vi "Lab Panel V3.1.vi"() -> ()   [LabVIEW 2013]
uses:
  <vilib>/Platform/TimedLoop/XDataNode/timing_clust.ctl
  <vilib>/Platform/TimedLoop/XDataNode/nitl_modes.ctl
  <vilib>/Platform/TimedLoop/XDataNode/wakeup.ctl
  Global 1.vi
  <vilib>/platform/TimedLoop/XDataNode/XDataNode.xnode
  <vilib>/Platform/TimedLoop/XDataNode/XDNodeRunTimeDep.lvlib
panel:
  out "TEMP update":bool
  out "AI update":bool
  in  "stop":bool
  in  "Tab Control 2":T1(tab)
  out "LAB05-2 (SIG)":T2 {"PF" format="%.2f"; "AMPS" format="%.1f"}
  out "LAB05-1 (SIG)":T2 {"PF" format="%.2f"; "AMPS" format="%.1f"}
  out "LAB04-2 (SIG)":T2 {"PF" format="%.2f"; "AMPS" format="%.1f"}
  out "LAB04-1 (SIG)":T2 {"PF" format="%.2f"; "AMPS" format="%.1f"}
  out "LAB03-2 (SIG)":T2 {"PF" format="%.2f"; "AMPS" format="%.1f"}
  out "LAB03-1 (SIG)":T2 {"PF" format="%.2f"; "AMPS" format="%.1f"}
  out "LAB02-2 (SIG)":T2 {"PF" format="%.2f"; "AMPS" format="%.1f"}
  in  "LAB01-1RUN":bool
  in  "LAB05-1 (O/I)":bool
  in  "LAB05-2 (O/I)":bool
  in  "LAB04-1 (O/I)":bool
  in  "LAB04-2 (O/I)":bool
  in  "LAB02-1 (O/I)":bool
  in  "LAB02-2 (O/I)":bool
  in  "LAB01-2 (O/I)":bool
  in  "LAB01-1 (O/I)":bool
  in  "LAB03-1 (O/I)":bool
  in  "LAB05-2 RUN":bool
  in  "LAB05-1 RUN":bool
  in  "LAB04-2 RUN":bool
  in  "LAB04-1 RUN":bool
  in  "LAB03-2 RUN":bool
  in  "LAB03-1 RUN":bool
  in  "LAB02-2 RUN":bool
  in  "LAB02-1 RUN":bool
  in  "LAB01-2 RUN":bool
  in  "LAB05-2 SELECT":T3(radio)
  in  "LAB05-1 SELECT":T3(radio)
  in  "LAB04-2 SELECT":T3(radio)
  in  "LAB04-1 SELECT":T3(radio)
  in  "LAB03-2 SELECT":T3(radio)
  in  "LAB03-1 SELECT":T3(radio)
  in  "LAB02-2 SELECT":T3(radio)
  in  "LAB02-1 SELECT":T3(radio)
  in  "LAB01-2 SELECT":T3(radio)
  in  "LAB01-1 SELECT":T3(radio)
  in  "LAB03-2 (O/I)":bool
  out "LAB01-1 (SIG)":T2 {"PF" format="%.2f"; "AMPS" format="%.1f"}
  out "LAB01-2 (SIG)":T2 {"PF" format="%.2f"; "AMPS" format="%.1f"}
  out "LAB02-1 (SIG)":T2 {"PF" format="%.2f"; "AMPS" format="%.1f"}
  out "LAB05-2 (DISP)":T4 {"MINS" format="%.2g"}
  out "LAB05-1 (DISP)":T4 {"MINS" format="%.2g"}
  out "LAB04-2 (DISP)":T4 {"MINS" format="%.2g"}
  out "LAB04-1 (DISP)":T4 {"MINS" format="%.2g"}
  out "LAB03-2 (DISP)":T4 {"MINS" format="%.2g"}
  out "LAB03-1 (DISP)":T4 {"MINS" format="%.2g"}
  in  "LAB05-2 (SET)":T5
  in  "LAB05-1 (SET)":T5
  in  "LAB04-2 (SET)":T5
  in  "LAB04-1 (SET)":T5
  in  "LAB03-2 (SET)":T5
  in  "LAB03-1 (SET)":T5
  out "LAB02-2 (DISP)":T4 {"MINS" format="%.2g"}
  out "LAB02-1 (DISP)":T4 {"MINS" format="%.2g"}
  in  "LAB02-2 (SET)":T5
  in  "LAB02-1 (SET)":T5
  out "LAB05-2 (RESULT)":bool
  out "LAB05-1 (RESULT)":bool
  out "LAB04-2 (RESULT)":bool
  out "LAB04-1 (RESULT)":bool
  out "LAB03-2 (RESULT)":bool
  out "LAB03-1 (RESULT)":bool
  out "LAB02-2 (RESULT)":bool
  out "LAB02-1 (RESULT)":bool
  out "LAB01-2 (RESULT)":bool
  out "LAB01-1 (RESULT)":bool
  in  "LAB01-1 (SET)":T5
  in  "LAB01-2 (SET)":T5
  out "LAB01-1 (DISP)":T4 {"MINS" format="%.2g"}
  out "LAB01-2 (DISP)":T4 {"MINS" format="%.2f"}
  in  "Network Directory":path
  in  "JIG OFF TIME (S)":dbl=2.0 min=2.0 max=10.0 step=0.5 format="%.1g"
  in  "JIG ON TIME (S)":dbl=1.0 min=1.0 max=10.0 step=0.5 format="%.1g"
  out "LAB05-2 (FAIL)":cluster{"LO":dbl, "HI":dbl}
  out "LAB05-1 (FAIL)":cluster{"LO":dbl, "HI":dbl}
  out "LAB04-2 (FAIL)":cluster{"LO":dbl, "HI":dbl}
  out "LAB04-1 (FAIL)":cluster{"LO":dbl, "HI":dbl}
  out "LAB03-2 (FAIL)":cluster{"LO":dbl, "HI":dbl}
  out "LAB03-1 (FAIL)":cluster{"LO":dbl, "HI":dbl}
  out "LAB02-2 (FAIL)":cluster{"LO":dbl, "HI":dbl}
  out "LAB02-1 (FAIL)":cluster{"LO":dbl, "HI":dbl}
  out "LAB01-2 (FAIL)":cluster{"LO":dbl, "HI":dbl}
  out "LAB01-1 (FAIL)":cluster{"LO":dbl, "HI":dbl}
  out "LAB05-2 (TEMP START)":cluster{"TL":dbl, "TN":dbl}
  out "LAB04-2 (TEMP START)":cluster{"TL":dbl, "TN":dbl}
  out "LAB03-2 (TEMP START)":cluster{"TL":dbl, "TN":dbl}
  out "LAB02-2 (TEMP START)":cluster{"TL":dbl, "TN":dbl}
  out "LAB01-2 (TEMP START)":cluster{"TL":dbl, "TN":dbl}
  out "LAB05-1 (TEMP START)":cluster{"TL":dbl, "TN":dbl}
  out "LAB04-1 (TEMP START)":cluster{"TL":dbl, "TN":dbl}
  out "LAB03-1 (TEMP START)":cluster{"TL":dbl, "TN":dbl}
  out "LAB02-1 (TEMP START)":cluster{"TL":dbl, "TN":dbl}
  out "LAB01-1 (TEMP START)":cluster{"TL":dbl, "TN":dbl}
  out "LAB01-1 (JIG)":bool
  out "LAB01-2 (JIG)":bool
  out "LAB02-1 (JIG)":bool
  out "LAB02-2 (JIG)":bool
  out "LAB03-1 (JIG)":bool
  out "LAB03-2 (JIG)":bool
  out "LAB04-1 (JIG)":bool
  out "LAB04-2 (JIG)":bool
  out "LAB05-1 (JIG)":bool
  out "LAB05-2 (JIG)":bool
  out "LAB01 (CAL)":T6 {"2 (TN) cal" min=0.0 step=0.01 format="%.2f"; "2 (TL) cal" min=0.0 step=0.01 format="%.2f"; "2 (PF) cal" min=0.0 step=0.01 format="%.2f"; "2 (V) cal" min=0.0 step=0.01 format="%.2f"; "2 (A) cal" min=0.0 step=0.01 format="%.2f"; "1 (TN) cal" min=0.0 step=0.01 format="%.2f"; "1 (TL) cal" min=0.0 step=0.01 format="%.2f"; "1 (PF) cal" min=0.0 step=0.01 format="%.2f"; "1 (V) cal" min=0.0 step=0.01 format="%.2f"; "1  (A) cal" min=0.0 step=0.01 format="%.2f"}
  out "LAB03 (CAL)":T6 {"2 (TN) cal" min=0.0 step=0.01 format="%.2f"; "2 (TL) cal" min=0.0 step=0.01 format="%.2f"; "2 (PF) cal" min=0.0 step=0.01 format="%.2f"; "2 (V) cal" min=0.0 step=0.01 format="%.2f"; "2 (A) cal" min=0.0 step=0.01 format="%.2f"; "1 (TN) cal" min=0.0 step=0.01 format="%.2f"; "1 (TL) cal" min=0.0 step=0.01 format="%.2f"; "1 (PF) cal" min=0.0 step=0.01 format="%.2f"; "1 (V) cal" min=0.0 step=0.01 format="%.2f"; "1  (A) cal" min=0.0 step=0.01 format="%.2f"}
  out "LAB02 (CAL)":T7 {"2 (TN) cal" min=0.0 step=0.01 format="%.2f"; "2 (TL) cal" min=0.0 step=0.01 format="%.2f"; "2 (PF) cal" min=0.0 step=0.01 format="%.2f"; "2 (V) cal" min=0.0 step=0.01 format="%.2f"; "2 (A) cal" min=0.0 step=0.01 format="%.2f"; "1 (TN) cal" min=0.0 step=0.01 format="%.2f"; "1 (TL) cal" min=0.0 step=0.01 format="%.2f"; "1 (PF) cal" min=0.0 step=0.01 format="%.2f"; "1 (V) cal" min=0.0 step=0.01 format="%.2f"; "1 (A) cal" min=0.0 step=0.01 format="%.2f"}
  out "LAB05 (CAL)":T6 {"2 (TN) cal" min=0.0 step=0.01 format="%.2f"; "2 (TL) cal" min=0.0 step=0.01 format="%.2f"; "2 (PF) cal" min=0.0 step=0.01 format="%.2f"; "2 (V) cal" min=0.0 step=0.01 format="%.2f"; "2 (A) cal" min=0.0 step=0.01 format="%.2f"; "1 (TN) cal" min=0.0 step=0.01 format="%.2f"; "1 (TL) cal" min=0.0 step=0.01 format="%.2f"; "1 (PF) cal" min=0.0 step=0.01 format="%.2f"; "1 (V) cal" min=0.0 step=0.01 format="%.2f"; "1  (A) cal" min=0.0 step=0.01 format="%.2f"}
  out "LAB04 (CAL)":T6 {"2 (TN) cal" min=0.0 step=0.01 format="%.2f"; "2 (TL) cal" min=0.0 step=0.01 format="%.2f"; "2 (PF) cal" min=0.0 step=0.01 format="%.2f"; "2 (V) cal" min=0.0 step=0.01 format="%.2f"; "2 (A) cal" min=0.0 step=0.01 format="%.2f"; "1 (TN) cal" min=0.0 step=0.01 format="%.2f"; "1 (TL) cal" min=0.0 step=0.01 format="%.2f"; "1 (PF) cal" min=0.0 step=0.01 format="%.2f"; "1 (V) cal" min=0.0 step=0.01 format="%.2f"; "1  (A) cal" min=0.0 step=0.01 format="%.2f"}
  out "calibration file error out":errorcluster
  in  "CALIBRATE":bool
  in  "Tab Control":T8(tab)
  out "LAB01-2 (GRAPH)":dynamicdata(graph)
  out "LAB01-1 (GRAPH)":dynamicdata(graph)
  out "LAB02-2 (GRAPH)":dynamicdata(graph)
  out "LAB02-1 (GRAPH)":dynamicdata(graph)
  out "LAB03-2 (GRAPH)":dynamicdata(graph)
  out "LAB03-1 (GRAPH)":dynamicdata(graph)
  out "LAB04-2 (GRAPH)":dynamicdata(graph)
  out "LAB04-1 (GRAPH)":dynamicdata(graph)
  out "LAB05-2 (GRAPH)":dynamicdata(graph)
  out "LAB05-1 (GRAPH)":dynamicdata(graph)
  out "LAB05 TEMP":T9
  out "LAB04 TEMP":T9
  out "LAB02 TEMP":T9
  out "LAB01 TEMP":T9
  out "LAB03 TEMP":T9
  out "Analog Error Array":errorcluster[](array[cluster])
  out "AI loop time":dbl format="%.6g"
  out "loops":dbl
  in  "loop  delay(mS)":dbl
  out "on loops":dbl
  out "off loops":dbl
  out "jig cycle":dbl
  out "LAB01-1 (TDMS)":refnum<k34>
  out "data file error":errorcluster
  out "LAB02-1 (TDMS)":refnum<k34>
  out "LAB01-2 (TDMS)":refnum<k34>
  out "LAB02-2 (TDMS)":refnum<k34>
  out "LAB03-1 (TDMS)":refnum<k34>
  out "LAB03-2 (TDMS)":refnum<k34>
  out "LAB04-1 (TDMS)":refnum<k34>
  out "LAB04-2 (TDMS)":refnum<k34>
  out "LAB05-1 (TDMS)":refnum<k34>
  out "LAB05-2 (TDMS)":refnum<k34>
  # "LAB01"
  # "LAB02"
  # "LAB05"
  # "LAB03"
  # "LAB04"
  # "LAB01"
  # "LAB02"
  # "LAB03"
  # "LAB04"
  # "LAB05"
  # "JIG SET"
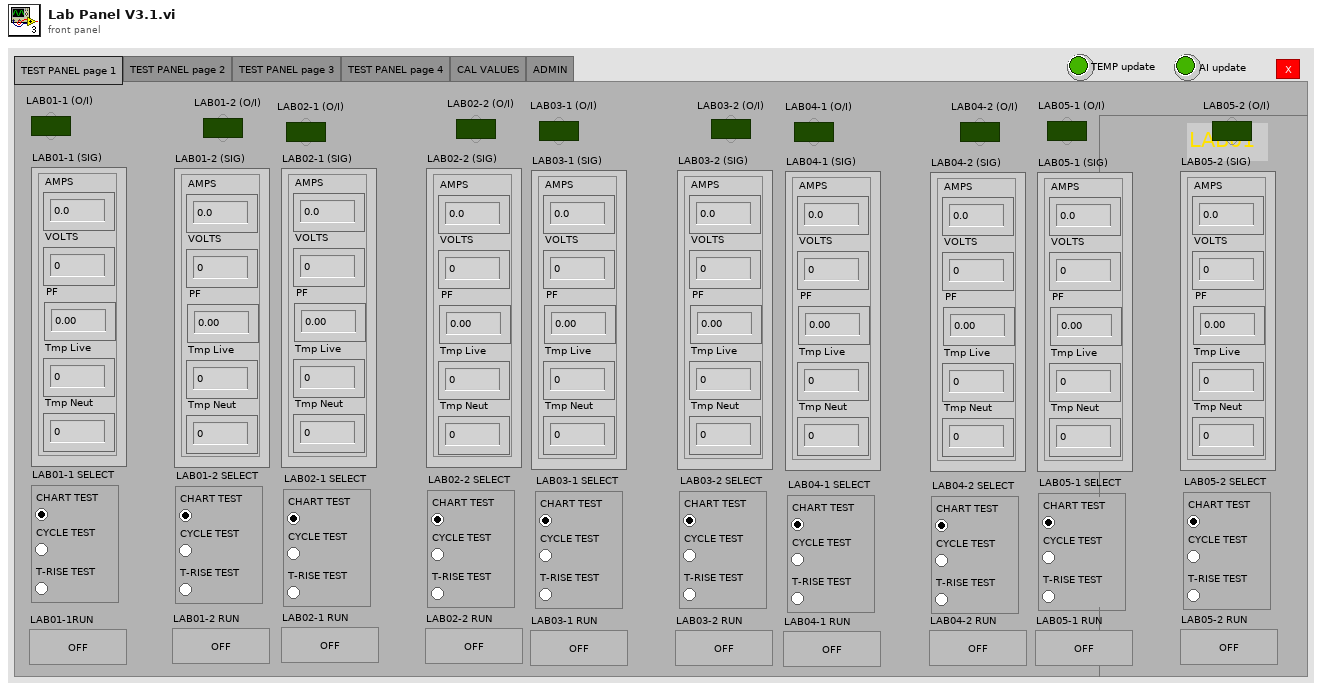
[diagram p1: front panel]
types:
  T1 = enum32{"TEST PANEL page 1", "TEST PANEL page 2", "TEST PANEL page 3", "TEST PANEL page 4", "CAL VALUES", "ADMIN"}
  T2 = cluster{"AMPS":dbl, "VOLTS":dbl, "PF":dbl, "Tmp Live":dbl, "Tmp Neut":dbl}
  T3 = enum32{"CHART TEST", "CYCLE TEST", "T-RISE TEST"}
  T4 = cluster{"CYCLE":dbl, "MINS":dbl, "STATUS":string}
  T5 = cluster{"NAME":string, "DESCRIPTION":string, "CYCLES":dbl, "T-RISE mins":dbl, "T-RISE deg C":dbl}
  T6 = cluster{"1  (A) cal":dbl, "1 (V) cal":dbl, "1 (PF) cal":dbl, "1 (TL) cal":dbl, "1 (TN) cal":dbl, "2 (A) cal":dbl, "2 (V) cal":dbl, "2 (PF) cal":dbl, "2 (TL) cal":dbl, "2 (TN) cal":dbl}
  T7 = cluster{"1 (A) cal":dbl, "1 (V) cal":dbl, "1 (PF) cal":dbl, "1 (TL) cal":dbl, "1 (TN) cal":dbl, "2 (A) cal":dbl, "2 (V) cal":dbl, "2 (PF) cal":dbl, "2 (TL) cal":dbl, "2 (TN) cal":dbl}
  T8 = enum32{"LAB01", "LAB02", "LAB03", "LAB04", "LAB05", "TEMPERATURE", "ERROR"}
  T9 = cluster{"T1 Live":dbl, "T1 Neut":dbl, "T2 Live":dbl, "T2 Neut":dbl, "ID":dbl, "ER":dbl}
  T10 = enum8{"Enabled", "Disabled", "Disabled and Grayed Out"}
  T11 = typedef "XDNodeRunTimeDep.lvlib/timing_clust.ctl" = cluster{"Expected End [f-1]":u64, "Actual End [f-1]":u64, "Finished Late? [f-1]":bool, "Expected End [i-1]":u64, "Actual End [i-1]":u64, "Finished Late? [i-1]":bool, "Expected Start [i]":u64, "Actual Start [i]":u64, "Expected Start [f]":u64, "Actual Start [f]":u64, "Source Name":string, "Structure Name":string, "Period":i64, "Deadline":i64, "Offset":i64, "Start":i64, "Priority":i32, "Timeout":i32, "Mode":T12, "Wakeup Reason":T13, "Error":errorcluster, "Source Type":string, "Secondary Source Type":string, "Global End Time":u64, "Global Start Time":u64, "Frame Duration":u64, "Iteration Duration":u64, "Assigned CPU":i32, "I/O Scan Engine Mode":u32}
  T12 = typedef "XDNodeRunTimeDep.lvlib/nitl_modes.ctl" = enum32{"No Change", "Process missed periods, maintain original phase", "Discard missed periods, maintain original phase", "Process missed periods, ignore original phase", "Discard missed periods, ignore original phase"}
  T13 = typedef "XDNodeRunTimeDep.lvlib/wakeup.ctl" = enum32{"Normal", "Aborted", "Asynchronous wakeup", "Timing source error", "Timed loop error", "Timeout"}
  T14 = enum16{"open", "open or create", "create or replace", "create", "open (read-only)"}
  T15 = enum16{"open", "replace", "create", "open or create", "replace or create", "replace or create with confirmation"}
  T16 = cluster{"LAB01-1 (SET)":cluster{"NAME":string, "DESCRIPTION":string, "CYCLES":dbl, "T-RISE mins":dbl, "T-RISE deg C":dbl}, "LAB01-2 (SET)":cluster{"NAME":string, "DESCRIPTION":string, "CYCLES":dbl, "T-RISE mins":dbl, "T-RISE deg C":dbl}, "LAB02-1 (SET)":cluster{"NAME":string, "DESCRIPTION":string, "CYCLES":dbl, "T-RISE mins":dbl, "T-RISE deg C":dbl}, "LAB02-2 (SET)":cluster{"NAME":string, "DESCRIPTION":string, "CYCLES":dbl, "T-RISE mins":dbl, "T-RISE deg C":dbl}, "LAB03-1 (SET)":cluster{"NAME":string, "DESCRIPTION":string, "CYCLES":dbl, "T-RISE mins":dbl, "T-RISE deg C":dbl}, "LAB03-2 (SET)":cluster{"NAME":string, "DESCRIPTION":string, "CYCLES":dbl, "T-RISE mins":dbl, "T-RISE deg C":dbl}, "LAB04-1 (SET)":cluster{"NAME":string, "DESCRIPTION":string, "CYCLES":dbl, "T-RISE mins":dbl, "T-RISE deg C":dbl}, "LAB04-2 (SET)":cluster{"NAME":string, "DESCRIPTION":string, "CYCLES":dbl, "T-RISE mins":dbl, "T-RISE deg C":dbl}, "LAB05-1 (SET)":cluster{"NAME":string, "DESCRIPTION":string, "CYCLES":dbl, "T-RISE mins":dbl, "T-RISE deg C":dbl}, "LAB05-2 (SET)":cluster{"NAME":string, "DESCRIPTION":string, "CYCLES":dbl, "T-RISE mins":dbl, "T-RISE deg C":dbl}, "Network Directory":path}
  T17 = cluster{"T1":dbl, "T2":dbl, "T3":dbl, "T4":dbl, "ID":dbl, "ER":dbl}
  T18 = cluster{"LAB01-1 (A)":dbl, "LAB01-1 (V)":dbl, "LAB01-1 (PF)":dbl, "LAB01-2 (A)":dbl, "LAB01-2 (V)":dbl, "LAB01-2 (PF)":dbl}
  T19 = cluster{"LAB02-1 (A)":dbl, "LAB02-1 (V)":dbl, "LAB02-1 (PF)":dbl, "LAB02-2 (A)":dbl, "LAB02-2 (V)":dbl, "LAB02-2 (PF)":dbl}
  T20 = cluster{"LAB03-1 (A)":dbl, "LAB03-1 (V)":dbl, "LAB03-1 (PF)":dbl, "LAB03-2 (A)":dbl, "LAB03-2 (V)":dbl, "LAB03-2 (PF)":dbl}
  T21 = cluster{"LAB04-1 (A)":dbl, "LAB04-1 (V)":dbl, "LAB04-1 (PF)":dbl, "LAB04-2 (A)":dbl, "LAB04-2 (V)":dbl, "LAB04-2 (PF)":dbl}
  T22 = cluster{"LAB05-1 (A)":dbl, "LAB05-1 (V)":dbl, "LAB05-1 (PF)":dbl, "LAB05-2 (A)":dbl, "LAB05-2 (V)":dbl, "LAB05-2 (PF)":dbl}
  T23 = cluster{"LAB01-1 (FAIL)":cluster{"LO":dbl, "HI":dbl}, "LAB01-1 (SIG)":cluster{"AMPS":dbl, "VOLTS":dbl, "PF":dbl, "Tmp Live":dbl, "Tmp Neut":dbl}, "LAB01-1 (TEMP START)":cluster{"TL":dbl, "TN":dbl}, "LAB01-1 (DISP)":cluster{"CYCLE":dbl, "MINS":dbl, "STATUS":string}, "LAB01-1 (SET)":cluster{"NAME":string, "DESCRIPTION":string, "CYCLES":dbl, "T-RISE mins":dbl, "T-RISE deg C":dbl}, "LAB01-1 (TDMS)":refnum<k34>}
  T24 = cluster{"LAB01-2 (FAIL)":cluster{"LO":dbl, "HI":dbl}, "LAB01-2 (SIG)":cluster{"AMPS":dbl, "VOLTS":dbl, "PF":dbl, "Tmp Live":dbl, "Tmp Neut":dbl}, "LAB01-2 (TEMP START)":cluster{"TL":dbl, "TN":dbl}, "LAB01-2 (DISP)":cluster{"CYCLE":dbl, "MINS":dbl, "STATUS":string}, "LAB01-2 (SET)":cluster{"NAME":string, "DESCRIPTION":string, "CYCLES":dbl, "T-RISE mins":dbl, "T-RISE deg C":dbl}, "LAB01-2 (TDMS)":refnum<k34>}
  T25 = cluster{"LAB02-1 (FAIL)":cluster{"LO":dbl, "HI":dbl}, "LAB02-1 (SIG)":cluster{"AMPS":dbl, "VOLTS":dbl, "PF":dbl, "Tmp Live":dbl, "Tmp Neut":dbl}, "LAB02-1 (TEMP START)":cluster{"TL":dbl, "TN":dbl}, "LAB02-1 (DISP)":cluster{"CYCLE":dbl, "MINS":dbl, "STATUS":string}, "LAB02-1 (SET)":cluster{"NAME":string, "DESCRIPTION":string, "CYCLES":dbl, "T-RISE mins":dbl, "T-RISE deg C":dbl}, "LAB02-1 (TDMS)":refnum<k34>}
  T26 = cluster{"LAB02-2 (FAIL)":cluster{"LO":dbl, "HI":dbl}, "LAB02-2 (SIG)":cluster{"AMPS":dbl, "VOLTS":dbl, "PF":dbl, "Tmp Live":dbl, "Tmp Neut":dbl}, "LAB02-2 (TEMP START)":cluster{"TL":dbl, "TN":dbl}, "LAB02-2 (DISP)":cluster{"CYCLE":dbl, "MINS":dbl, "STATUS":string}, "LAB02-2 (SET)":cluster{"NAME":string, "DESCRIPTION":string, "CYCLES":dbl, "T-RISE mins":dbl, "T-RISE deg C":dbl}, "LAB02-2 (TDMS)":refnum<k34>}
  T27 = cluster{"LAB03-1 (FAIL)":cluster{"LO":dbl, "HI":dbl}, "LAB03-1 (SIG)":cluster{"AMPS":dbl, "VOLTS":dbl, "PF":dbl, "Tmp Live":dbl, "Tmp Neut":dbl}, "LAB03-1 (TEMP START)":cluster{"TL":dbl, "TN":dbl}, "LAB03-1 (DISP)":cluster{"CYCLE":dbl, "MINS":dbl, "STATUS":string}, "LAB03-1 (SET)":cluster{"NAME":string, "DESCRIPTION":string, "CYCLES":dbl, "T-RISE mins":dbl, "T-RISE deg C":dbl}, "LAB03-1 (TDMS)":refnum<k34>}
  T28 = cluster{"LAB03-2 (FAIL)":cluster{"LO":dbl, "HI":dbl}, "LAB03-2 (SIG)":cluster{"AMPS":dbl, "VOLTS":dbl, "PF":dbl, "Tmp Live":dbl, "Tmp Neut":dbl}, "LAB03-2 (TEMP START)":cluster{"TL":dbl, "TN":dbl}, "LAB03-2 (DISP)":cluster{"CYCLE":dbl, "MINS":dbl, "STATUS":string}, "LAB03-2 (SET)":cluster{"NAME":string, "DESCRIPTION":string, "CYCLES":dbl, "T-RISE mins":dbl, "T-RISE deg C":dbl}, "LAB03-2 (TDMS)":refnum<k34>}
  T29 = cluster{"LAB04-1 (FAIL)":cluster{"LO":dbl, "HI":dbl}, "LAB04-1 (SIG)":cluster{"AMPS":dbl, "VOLTS":dbl, "PF":dbl, "Tmp Live":dbl, "Tmp Neut":dbl}, "LAB04-1 (TEMP START)":cluster{"TL":dbl, "TN":dbl}, "LAB04-1 (DISP)":cluster{"CYCLE":dbl, "MINS":dbl, "STATUS":string}, "LAB04-1 (SET)":cluster{"NAME":string, "DESCRIPTION":string, "CYCLES":dbl, "T-RISE mins":dbl, "T-RISE deg C":dbl}, "LAB04-1 (TDMS)":refnum<k34>}
  T30 = cluster{"LAB04-2 (FAIL)":cluster{"LO":dbl, "HI":dbl}, "LAB04-2 (SIG)":cluster{"AMPS":dbl, "VOLTS":dbl, "PF":dbl, "Tmp Live":dbl, "Tmp Neut":dbl}, "LAB04-2 (TEMP START)":cluster{"TL":dbl, "TN":dbl}, "LAB04-2 (DISP)":cluster{"CYCLE":dbl, "MINS":dbl, "STATUS":string}, "LAB04-2 (SET)":cluster{"NAME":string, "DESCRIPTION":string, "CYCLES":dbl, "T-RISE mins":dbl, "T-RISE deg C":dbl}, "LAB04-2 (TDMS)":refnum<k34>}
  T31 = cluster{"LAB05-1 (FAIL)":cluster{"LO":dbl, "HI":dbl}, "LAB05-1 (SIG)":cluster{"AMPS":dbl, "VOLTS":dbl, "PF":dbl, "Tmp Live":dbl, "Tmp Neut":dbl}, "LAB05-1 (TEMP START)":cluster{"TL":dbl, "TN":dbl}, "LAB05-1 (DISP)":cluster{"CYCLE":dbl, "MINS":dbl, "STATUS":string}, "LAB05-1 (SET)":cluster{"NAME":string, "DESCRIPTION":string, "CYCLES":dbl, "T-RISE mins":dbl, "T-RISE deg C":dbl}, "LAB05-1 (TDMS)":refnum<k34>}
  T32 = cluster{"LAB05-2 (FAIL)":cluster{"LO":dbl, "HI":dbl}, "LAB05-2 (SIG)":cluster{"AMPS":dbl, "VOLTS":dbl, "PF":dbl, "Tmp Live":dbl, "Tmp Neut":dbl}, "LAB05-2 (TEMP START)":cluster{"TL":dbl, "TN":dbl}, "LAB05-2 (DISP)":cluster{"CYCLE":dbl, "MINS":dbl, "STATUS":string}, "LAB05-2 (SET)":cluster{"NAME":string, "DESCRIPTION":string, "CYCLES":dbl, "T-RISE mins":dbl, "T-RISE deg C":dbl}, "LAB05-2 (TDMS)":refnum<k34>}
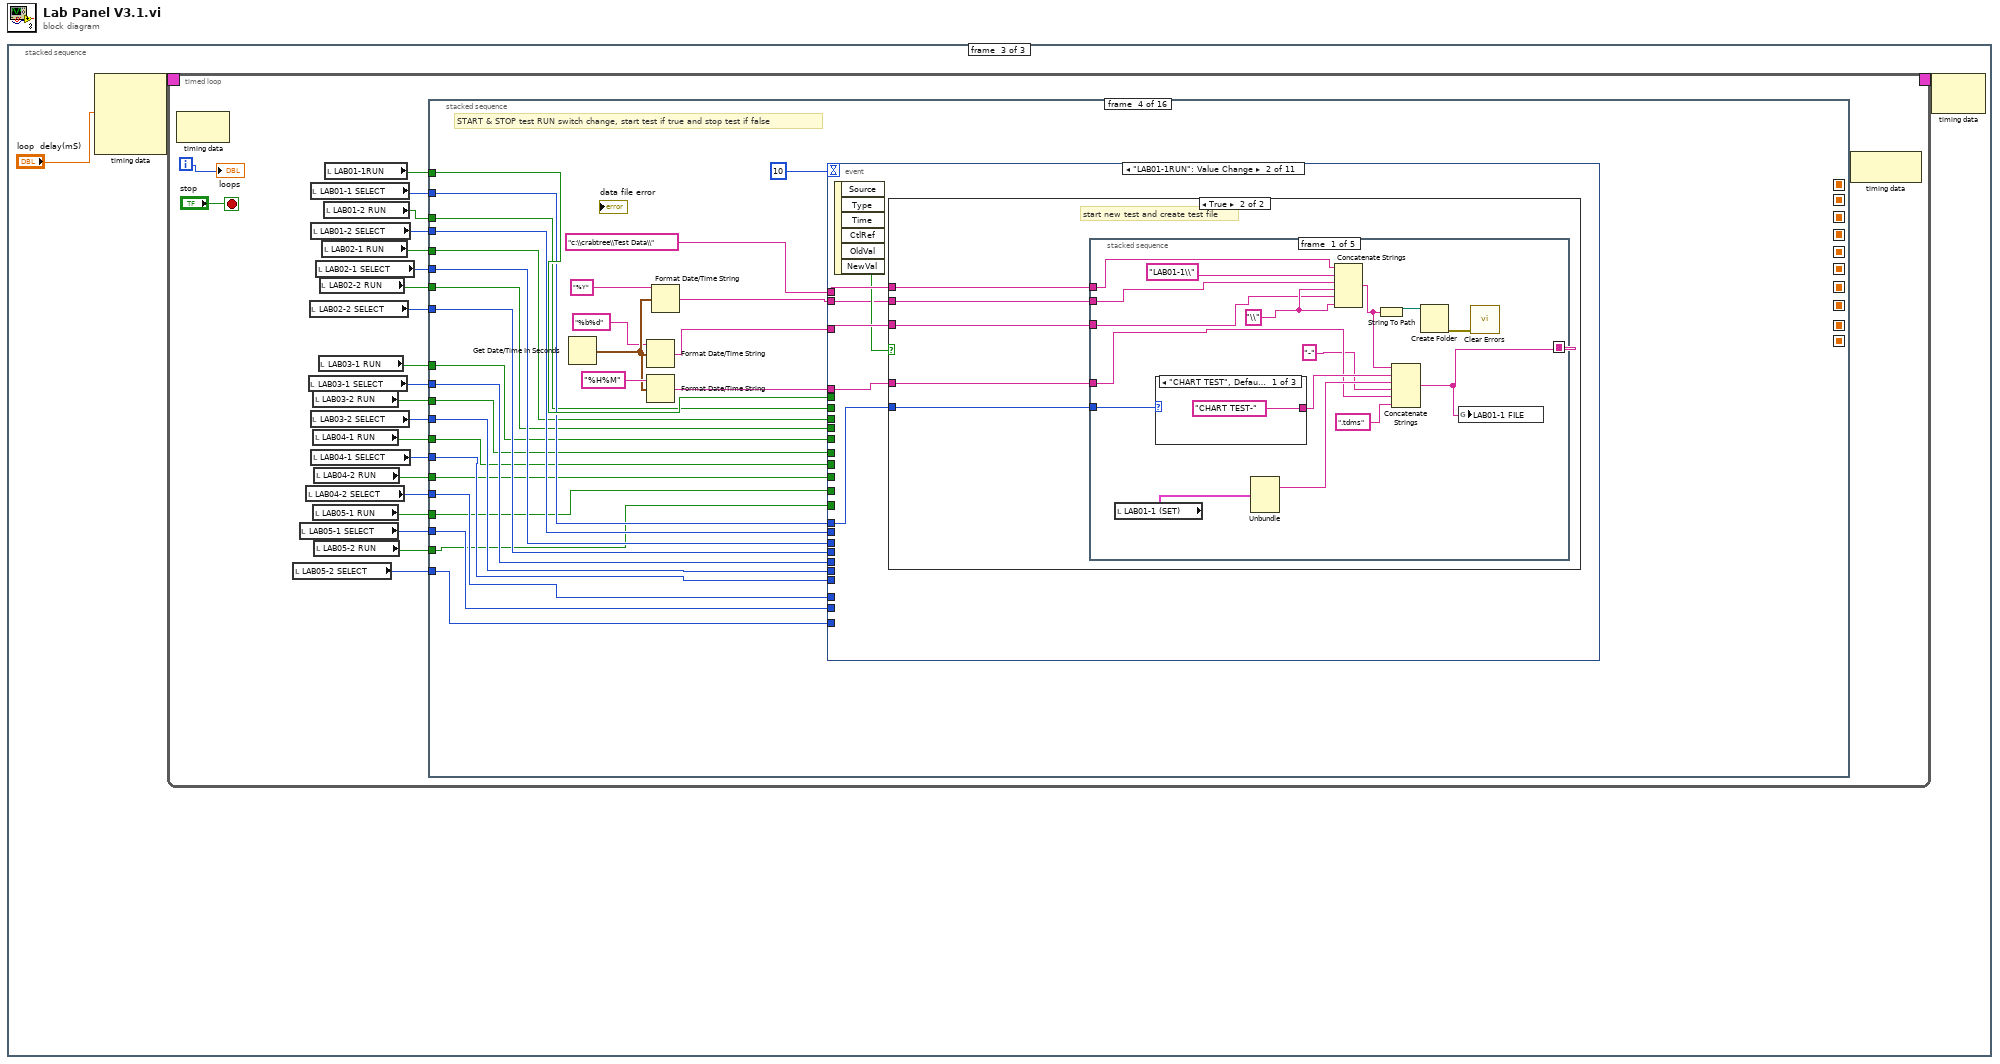
[diagram p0: block diagram]
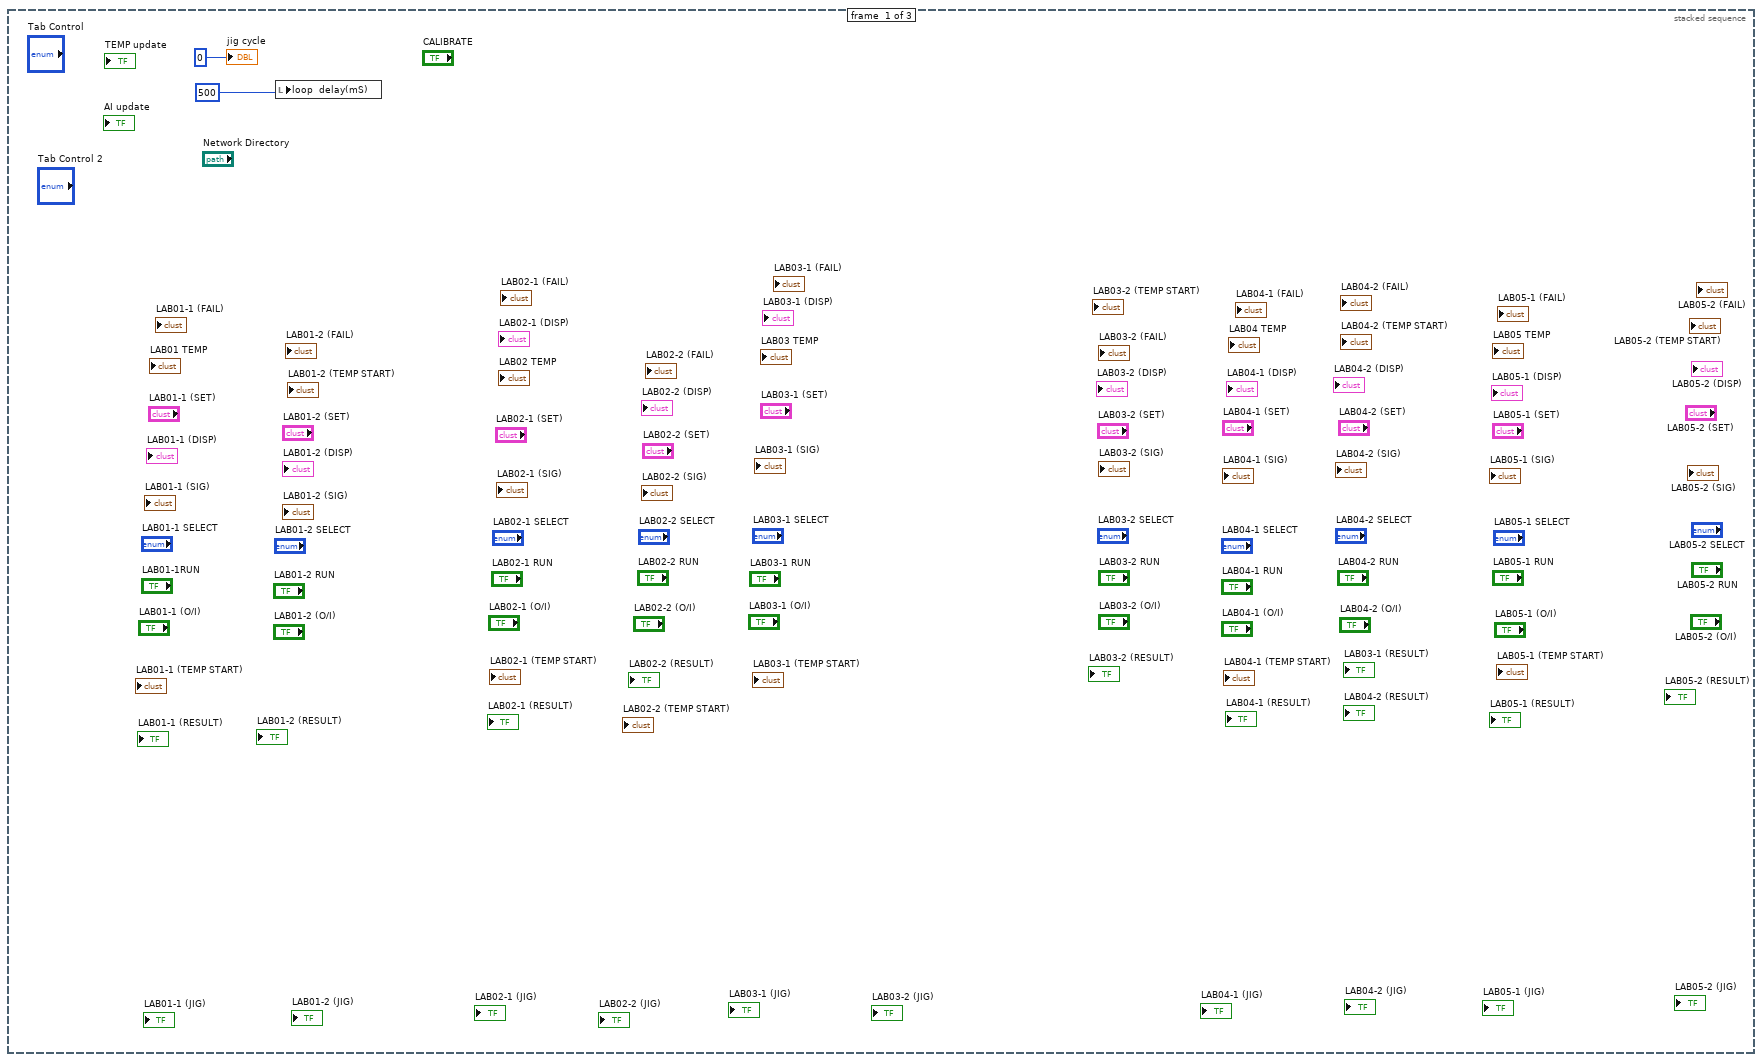
[diagram p2: hidden frame]
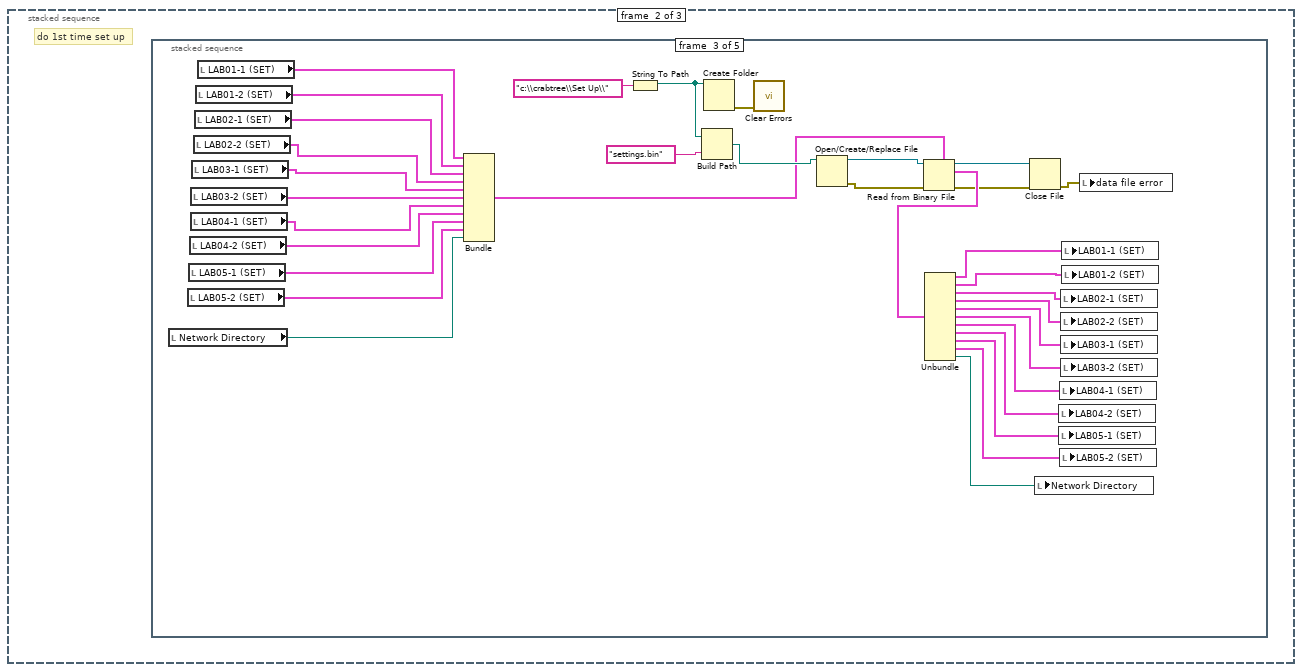
[diagram p3: hidden frame]
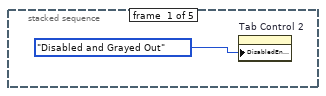
[diagram p4: hidden frame]
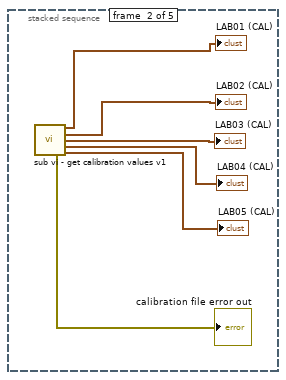
[diagram p5: hidden frame]
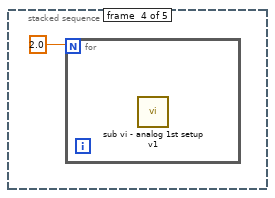
[diagram p6: hidden frame]
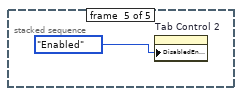
[diagram p7: hidden frame]
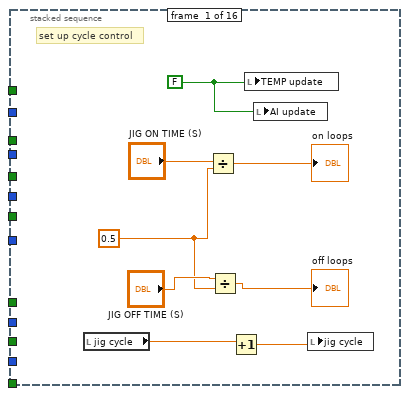
[diagram p8: hidden frame]
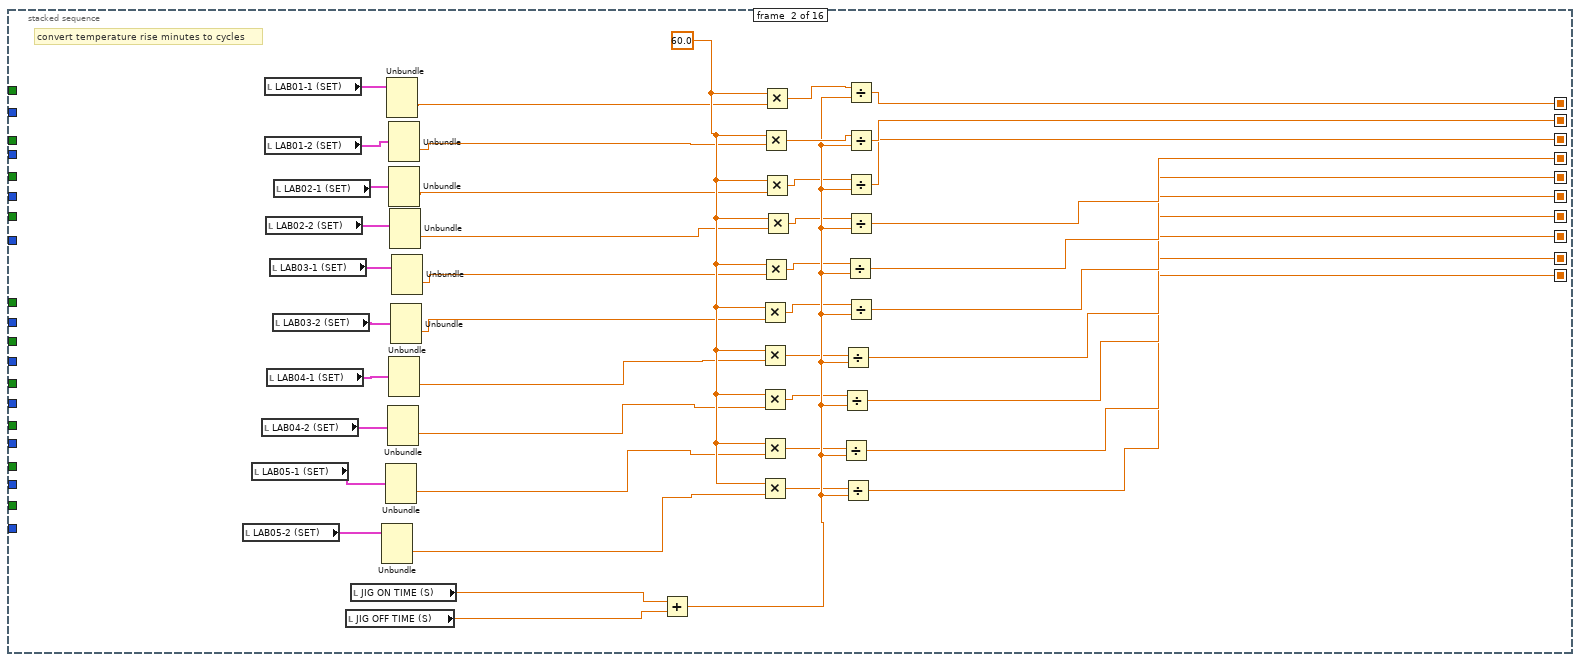
[diagram p9: hidden frame]
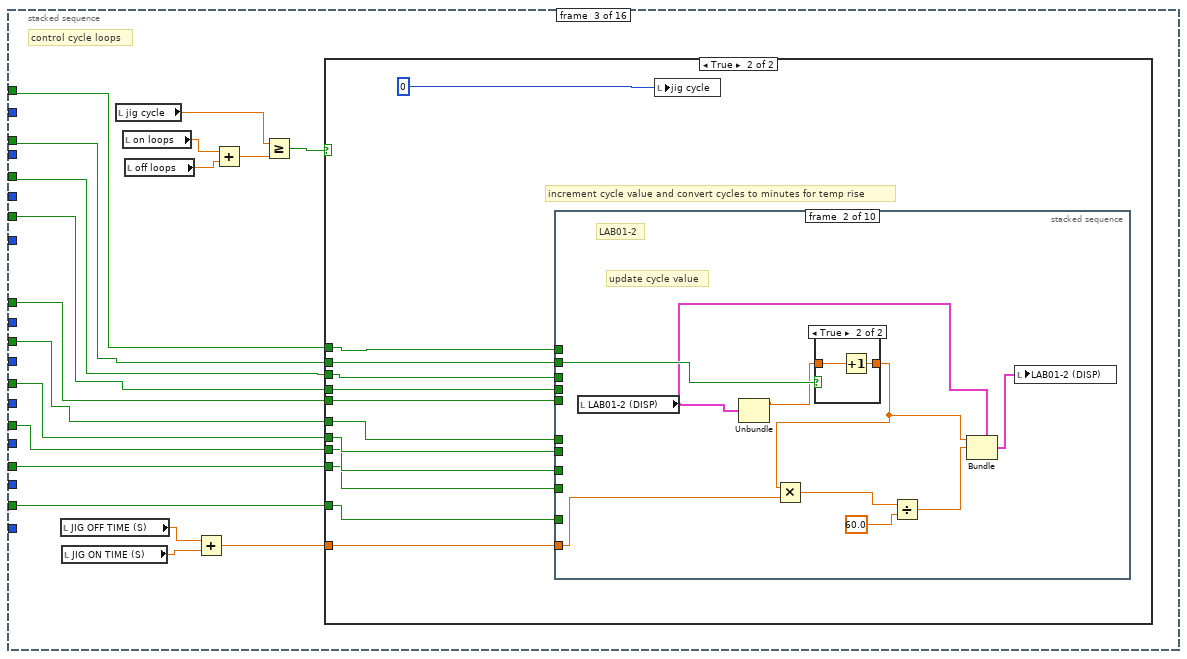
[diagram p10: hidden frame]
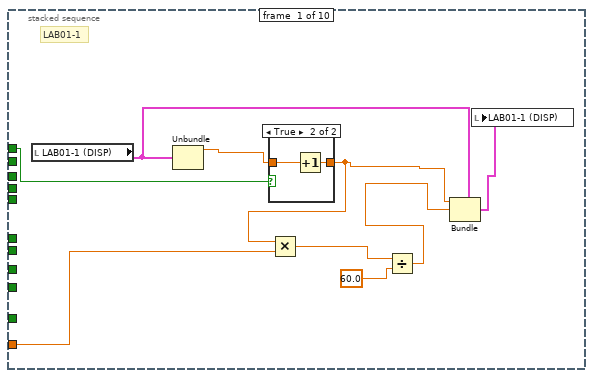
[diagram p12: hidden frame]
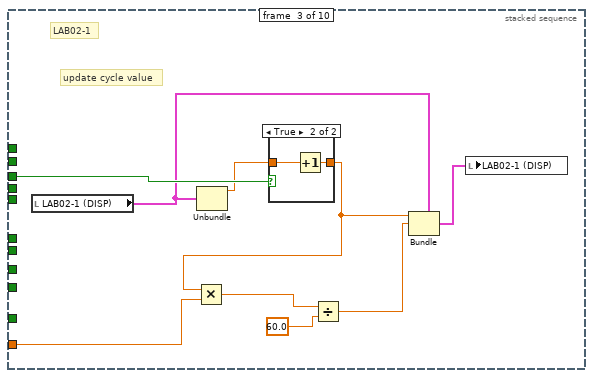
[diagram p15: hidden frame]
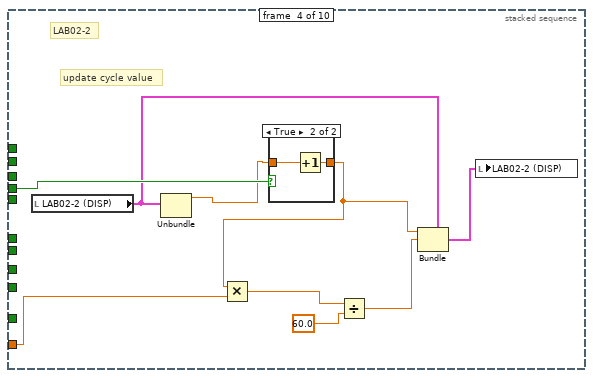
[diagram p17: hidden frame]
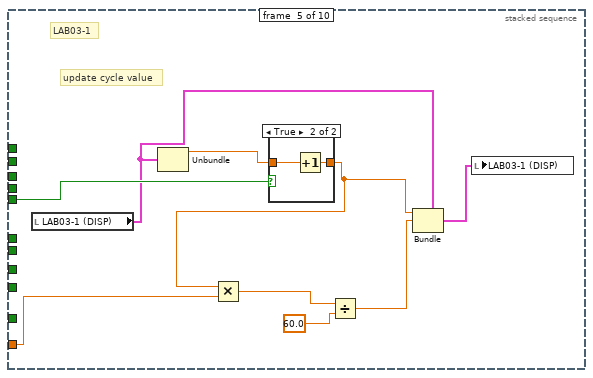
[diagram p19: hidden frame]
diagram:
  n1 = stacked-sequence {
    frame #0 {
      n2 = local write "loop  delay(mS)"(500) -> ()
      "jig cycle" <- 0
    }
    frame #1 {
      # "do 1st time set up"
      n3 = stacked-sequence {
        frame #0 {
          n4 = property on="Tab Control 2" class="TabCtl (strict)"("DisabledEnum"=T10."Disabled and Grayed Out" ("Disabled")) -> ()  [unwired: 2 in, 2 out]
        }
        frame #1 {
          n5 = call "sub vi - get calibration values v1.vi"() -> ("LAB01 (CAL)"=→"LAB01 (CAL)":T6, "LAB02 (CAL)"=→"LAB02 (CAL)":T7, "LAB03 (CAL)"=→"LAB03 (CAL)":T6, "LAB04 (CAL)"=→"LAB04 (CAL)":T6, "calibration file error out"=→"calibration file error out":errorcluster, "LAB05 (CAL)"=→"LAB05 (CAL)":T6)  [unwired: 10 in]
        }
        frame #2 {
          n6 = local read "Network Directory"() -> (w39:path)
          n7 = local read "LAB05-2 (SET)"() -> (w40:T5)
          n8 = local read "LAB05-1 (SET)"() -> (w41:T5)
          n9 = local read "LAB04-2 (SET)"() -> (w42:T5)
          n10 = local read "LAB03-2 (SET)"() -> (w38:T5)
          n11 = local read "LAB04-1 (SET)"() -> (w43:T5)
          n12 = local read "LAB03-1 (SET)"() -> (w37:T5)
          n13 = local read "LAB02-2 (SET)"() -> (w36:T5)
          n14 = local read "LAB02-1 (SET)"() -> (w35:T5)
          n15 = local read "LAB01-2 (SET)"() -> (w34:T5)
          n16 = local read "LAB01-1 (SET)"() -> (w33:T5)
          n17 = Bundle("LAB01-1 (SET)"=w33, "LAB01-2 (SET)"=w34, "LAB02-1 (SET)"=w35, "LAB02-2 (SET)"=w36, "LAB03-1 (SET)"=w37, "LAB03-2 (SET)"=w38, "LAB04-1 (SET)"=w43, "LAB04-2 (SET)"=w42, "LAB05-1 (SET)"=w41, "LAB05-2 (SET)"=w40, "Network Directory"=w39) -> (w26:T16)  [unwired: 1 in]
          n18 = String To Path(string="c:\\crabtree\\Set Up\\") -> (path=w30:path)
          n19 = Build Path(base path=w30, name or relative path="settings.bin") -> (appended path=w28:path)
          n20 = Create Folder(path (use dialog)=w30) -> (error out=w32:errorcluster)  [unwired: 2 in, 2 out]
          n21 = call <vilib>:"Clear Errors.vi"("error in (no error)"=w32) -> ()  [unwired: 6 in, 1 out]
          n22 = Open/Create/Replace File(file path (use dialog)=w28) -> (refnum out=w25:refnum<file>, error out=w27:errorcluster)  [unwired: 5 in, 1 out]
          n23 = Read from Binary File(5:w26, 8:w27, 11:w25) -> (0:w22:errorcluster, 2:w24:T16, 3:w23:refnum<file>)  [unwired: 3 in, 1 out]
          n24 = Unbundle(w24) -> ("LAB01-1 (SET)"=w20:T5, "LAB01-2 (SET)"=w19:T5, "LAB02-1 (SET)"=w18:T5, "LAB02-2 (SET)"=w17:T5, "LAB03-1 (SET)"=w16:T5, "LAB03-2 (SET)"=w15:T5, "LAB04-1 (SET)"=w14:T5, "LAB04-2 (SET)"=w13:T5, "LAB05-1 (SET)"=w12:T5, "LAB05-2 (SET)"=w11:T5, "Network Directory"=w10:path)
          n25 = Close File(refnum=w23, error in=w22) -> (error out=w21:errorcluster)  [unwired: 1 out]
          n26 = local write "Network Directory"(w10) -> ()
          n27 = local write "LAB04-2 (SET)"(w13) -> ()
          n28 = local write "LAB05-1 (SET)"(w12) -> ()
          n29 = local write "LAB04-1 (SET)"(w14) -> ()
          n30 = local write "LAB05-2 (SET)"(w11) -> ()
          n31 = local write "LAB02-1 (SET)"(w18) -> ()
          n32 = local write "LAB02-2 (SET)"(w17) -> ()
          n33 = local write "LAB03-1 (SET)"(w16) -> ()
          n34 = local write "LAB03-2 (SET)"(w15) -> ()
          n35 = local write "LAB01-1 (SET)"(w20) -> ()
          n36 = local write "LAB01-2 (SET)"(w19) -> ()
          n37 = local write "data file error"(w21) -> ()
        }
        frame #3 {
          n38 = for {
            N: 2.0 -> [_]
            n39 = call "sub vi - analog 1st setup v1.vi"() -> ()  [unwired: 11 in, 5 out]
          }
        }
        frame #4 {
          n40 = property on="Tab Control 2" class="TabCtl (strict)"("DisabledEnum"=T10."Enabled" ("Disabled")) -> ()  [unwired: 2 in, 2 out]
        }
      }
    }
    frame #2 {
      n41 = node-c288("loop  delay(mS)") -> (w48:T11)  [unwired: 3 in]
      n42 = timed-loop {
        timing: w48 -> [_]
        timing-out: [_] -> w47
        i -> [w70]
        stop <- "stop" stop-if-true
        n43 = node-c288() -> ()  [unwired: 1 in, 1 out]
        n44 = local read "LAB05-2 SELECT"() -> (w49:T3)
        n45 = local read "LAB05-1 SELECT"() -> (w50:T3)
        n46 = local read "LAB04-2 SELECT"() -> (w51:T3)
        n47 = local read "LAB03-1 SELECT"() -> (w54:T3)
        n48 = local read "LAB02-2 SELECT"() -> (w55:T3)
        n49 = local read "LAB01-1 SELECT"() -> (w58:T3)
        n50 = local read "LAB03-2 SELECT"() -> (w53:T3)
        n51 = local read "LAB01-2 SELECT"() -> (w57:T3)
        n52 = local read "LAB04-1 SELECT"() -> (w52:T3)
        n53 = local read "LAB03-2 RUN"() -> (w63:bool)
        n54 = local read "LAB04-1 RUN"() -> (w62:bool)
        n55 = local read "LAB05-1 RUN"() -> (w60:bool)
        n56 = local read "LAB04-2 RUN"() -> (w61:bool)
        n57 = local read "LAB05-2 RUN"() -> (w59:bool)
        n58 = local read "LAB02-1 SELECT"() -> (w56:T3)
        n59 = local read "LAB03-1 RUN"() -> (w64:bool)
        n60 = local read "LAB02-2 RUN"() -> (w65:bool)
        n61 = local read "LAB02-1 RUN"() -> (w66:bool)
        n62 = local read "LAB01-2 RUN"() -> (w67:bool)
        n63 = local read "LAB01-1RUN"() -> (w68:bool)
        n64 = stacked-sequence {
          seq-local: [_ w122 _ _ _ _ _ _ _ _ _ _ _ _ _ _] -> [_ _ _ _ _ w1553 _ _ _ _ _ _ _ _ _ _]
          seq-local: [_ w121 _ _ _ _ _ _ _ _ _ _ _ _ _ _] -> [_ _ _ _ _ w1552 _ _ _ _ _ _ _ _ _ _]
          seq-local: [_ w108 _ _ _ _ _ _ _ _ _ _ _ _ _ _] -> [_ _ _ _ _ w1551 _ _ _ _ _ _ _ _ _ _]
          seq-local: [_ w107 _ _ _ _ _ _ _ _ _ _ _ _ _ _] -> [_ _ _ _ _ w1550 _ _ _ _ _ _ _ _ _ _]
          seq-local: [_ w106 _ _ _ _ _ _ _ _ _ _ _ _ _ _] -> [_ _ _ _ _ w1549 _ _ _ _ _ _ _ _ _ _]
          seq-local: [_ w105 _ _ _ _ _ _ _ _ _ _ _ _ _ _] -> [_ _ _ _ _ w1548 _ _ _ _ _ _ _ _ _ _]
          seq-local: [_ w104 _ _ _ _ _ _ _ _ _ _ _ _ _ _] -> [_ _ _ _ _ w1547 _ _ _ _ _ _ _ _ _ _]
          seq-local: [_ w103 _ _ _ _ _ _ _ _ _ _ _ _ _ _] -> [_ _ _ _ _ w1546 _ _ _ _ _ _ _ _ _ _]
          seq-local: [_ w102 _ _ _ _ _ _ _ _ _ _ _ _ _ _] -> [_ _ _ _ _ w1545 _ _ _ _ _ _ _ _ _ _]
          seq-local: [_ w101 _ _ _ _ _ _ _ _ _ _ _ _ _ _] -> [_ _ _ _ _ w1544 _ _ _ _ _ _ _ _ _ _]
          tunnel: w68 -> [_ _ w138 w298 w1153 w1573 w1883 w1965 _ _ _ _ w2489 w2977 _ _]
          tunnel: w67 -> [_ _ w137 w296 w1152 w1572 w1882 w1966 _ _ _ _ w2488 w2975 _ _]
          tunnel: w66 -> [_ _ w136 w294 w1151 w1571 w1881 w1964 _ _ _ _ w2487 w2973 _ _]
          tunnel: w65 -> [_ _ w135 w292 w1150 w1570 w1880 w1963 _ _ _ _ w2486 w2971 _ _]
          tunnel: w64 -> [_ _ w134 w290 w1149 w1569 w1879 w1962 _ _ _ _ w2485 w2969 _ _]
          tunnel: w63 -> [_ _ w133 w288 w1148 w1568 w1878 w1961 _ _ _ _ w2484 w2967 _ _]
          tunnel: w62 -> [_ _ w132 w286 w1147 w1567 w1877 w1960 _ _ _ _ w2483 w2965 _ _]
          tunnel: w61 -> [_ _ w131 w284 w1146 w1566 w1876 w1959 _ _ _ _ w2482 w2963 _ _]
          tunnel: w60 -> [_ _ w130 w282 w1145 w1565 w1875 w1958 _ _ _ _ w2481 w2961 _ _]
          tunnel: w59 -> [_ _ w129 w280 w1144 w1564 w1874 w1957 _ _ _ _ w2480 w2959 _ _]
          tunnel: w58 -> [_ _ _ w297 w1143 w1563 _ _ _ _ _ _ _ w2979 _ _]
          tunnel: w57 -> [_ _ _ w295 w1142 w1562 _ _ _ _ _ _ _ w2974 _ _]
          tunnel: w56 -> [_ _ _ w293 w1141 w1561 _ _ _ _ _ _ _ w2972 _ _]
          tunnel: w55 -> [_ _ _ w291 w1140 w1560 _ _ _ _ _ _ _ w2970 _ _]
          tunnel: w54 -> [_ _ _ w289 w1139 w1559 _ _ _ _ _ _ _ w2968 _ _]
          tunnel: w53 -> [_ _ _ w287 w1138 w1558 _ _ _ _ _ _ _ w2966 _ _]
          tunnel: w52 -> [_ _ _ w285 w1137 w1557 _ _ _ _ _ _ _ w2964 _ _]
          tunnel: w51 -> [_ _ _ w283 w1136 w1556 _ _ _ _ _ _ _ w2962 _ _]
          tunnel: w50 -> [_ _ _ w281 w1135 w1555 _ _ _ _ _ _ _ w2960 _ _]
          tunnel: w49 -> [_ _ _ w279 w1134 w1554 _ _ _ _ _ _ _ w2958 _ _]
          frame #0 {
            w73 = FALSE
            w78 = 0.5
            # "set up cycle control"
            n65 = local read "jig cycle"() -> (w77:dbl)
            n66 = Divide(x="JIG ON TIME (S)", y=w78) -> (x/y=→"on loops":dbl)
            n67 = Divide(x="JIG OFF TIME (S)", y=w78) -> (x/y=→"off loops":dbl)
            n68 = Increment(x=w77) -> (x+1=w76:dbl)
            n69 = local write "TEMP update"(w73) -> ()
            n70 = local write "AI update"(w73) -> ()
            n71 = local write "jig cycle"(w76) -> ()
          }
          frame #1 {
            w118 = 60.0
            # "convert temperature rise minutes to cycles"
            n72 = local read "LAB05-2 (SET)"() -> (w82:T5)
            n73 = local read "LAB05-1 (SET)"() -> (w84:T5)
            n74 = local read "LAB04-2 (SET)"() -> (w86:T5)
            n75 = local read "LAB01-1 (SET)"() -> (w100:T5)
            n76 = local read "LAB01-2 (SET)"() -> (w98:T5)
            n77 = local read "LAB02-2 (SET)"() -> (w94:T5)
            n78 = local read "LAB04-1 (SET)"() -> (w88:T5)
            n79 = local read "LAB03-1 (SET)"() -> (w92:T5)
            n80 = local read "LAB03-2 (SET)"() -> (w90:T5)
            n81 = local read "LAB02-1 (SET)"() -> (w96:T5)
            n82 = local read "JIG OFF TIME (S)"() -> (w123:dbl)
            n83 = local read "JIG ON TIME (S)"() -> (w124:dbl)
            n84 = Unbundle(w82) -> ("T-RISE mins"=w81:dbl)  [unwired: 4 out]
            n85 = Unbundle(w84) -> ("T-RISE mins"=w83:dbl)  [unwired: 4 out]
            n86 = Unbundle(w100) -> ("T-RISE mins"=w99:dbl)  [unwired: 4 out]
            n87 = Unbundle(w86) -> ("T-RISE mins"=w85:dbl)  [unwired: 4 out]
            n88 = Unbundle(w98) -> ("T-RISE mins"=w97:dbl)  [unwired: 4 out]
            n89 = Unbundle(w96) -> ("T-RISE mins"=w95:dbl)  [unwired: 4 out]
            n90 = Unbundle(w88) -> ("T-RISE mins"=w87:dbl)  [unwired: 4 out]
            n91 = Unbundle(w94) -> ("T-RISE mins"=w93:dbl)  [unwired: 4 out]
            n92 = Unbundle(w90) -> ("T-RISE mins"=w89:dbl)  [unwired: 4 out]
            n93 = Unbundle(w92) -> ("T-RISE mins"=w91:dbl)  [unwired: 4 out]
            n94 = Add(x=w124, y=w123) -> (x+y=w117:dbl)
            n95 = Multiply(x=w118, y=w89) -> (x*y=w113:dbl)
            n96 = Multiply(x=w118, y=w87) -> (x*y=w112:dbl)
            n97 = Multiply(x=w118, y=w85) -> (x*y=w111:dbl)
            n98 = Multiply(x=w118, y=w83) -> (x*y=w110:dbl)
            n99 = Multiply(x=w118, y=w81) -> (x*y=w109:dbl)
            n100 = Multiply(x=w118, y=w97) -> (x*y=w119:dbl)
            n101 = Multiply(x=w118, y=w91) -> (x*y=w114:dbl)
            n102 = Multiply(x=w118, y=w99) -> (x*y=w120:dbl)
            n103 = Multiply(x=w118, y=w95) -> (x*y=w116:dbl)
            n104 = Multiply(x=w118, y=w93) -> (x*y=w115:dbl)
            n105 = Divide(x=w110, y=w117) -> (x/y=w102:dbl)
            n106 = Divide(x=w111, y=w117) -> (x/y=w103:dbl)
            n107 = Divide(x=w112, y=w117) -> (x/y=w104:dbl)
            n108 = Divide(x=w109, y=w117) -> (x/y=w101:dbl)
            n109 = Divide(x=w114, y=w117) -> (x/y=w106:dbl)
            n110 = Divide(x=w120, y=w117) -> (x/y=w122:dbl)
            n111 = Divide(x=w119, y=w117) -> (x/y=w121:dbl)
            n112 = Divide(x=w116, y=w117) -> (x/y=w108:dbl)
            n113 = Divide(x=w115, y=w117) -> (x/y=w107:dbl)
            n114 = Divide(x=w113, y=w117) -> (x/y=w105:dbl)
          }
          frame #2 {
            # "control cycle loops"
            n115 = local read "JIG OFF TIME (S)"() -> (w127:dbl)
            n116 = local read "JIG ON TIME (S)"() -> (w126:dbl)
            n117 = local read "jig cycle"() -> (w140:dbl)
            n118 = local read "on loops"() -> (w142:dbl)
            n119 = local read "off loops"() -> (w141:dbl)
            n120 = Add(x=w127, y=w126) -> (x+y=w125:dbl)
            n121 = Add(x=w142, y=w141) -> (x+y=w128:dbl)
            n122 = Greater Or Equal?(x=w140, y=w128) -> (x >= y?=w139:bool)
            n123 = case shown="True" w139 {
              tunnel: w138 -> [_ w153]
              tunnel: w137 -> [_ w152]
              tunnel: w136 -> [_ w151]
              tunnel: w135 -> [_ w150]
              tunnel: w134 -> [_ w149]
              tunnel: w133 -> [_ w148]
              tunnel: w132 -> [_ w147]
              tunnel: w131 -> [_ w146]
              tunnel: w130 -> [_ w145]
              tunnel: w129 -> [_ w144]
              tunnel: w125 -> [_ w143]
              frame False {
              }
              frame True {
                # "increment cycle value and convert cycles to minutes for temp rise"
                n124 = stacked-sequence {
                  tunnel: w153 -> [w163 _ _ _ _ _ _ _ _ _]
                  tunnel: w152 -> [_ w175 _ _ _ _ _ _ _ _]
                  tunnel: w151 -> [_ _ w187 _ _ _ _ _ _ _]
                  tunnel: w150 -> [_ _ _ w199 _ _ _ _ _ _]
                  tunnel: w149 -> [_ _ _ _ w211 _ _ _ _ _]
                  tunnel: w148 -> [_ _ _ _ _ w223 _ _ _ _]
                  tunnel: w147 -> [_ _ _ _ _ _ w235 _ _ _]
                  tunnel: w146 -> [_ _ _ _ _ _ _ w247 _ _]
                  tunnel: w145 -> [_ _ _ _ _ _ _ _ w259 _]
                  tunnel: w144 -> [_ _ _ _ _ _ _ _ _ w271]
                  tunnel: w143 -> [w160 w172 w184 w196 w208 w220 w232 w244 w256 w268]
                  frame #0 {
                    # "LAB01-1"
                    n125 = local read "LAB01-1 (DISP)"() -> (w158:T4)
                    n126 = Unbundle(w158) -> ("CYCLE"=w159:dbl)  [unwired: 2 out]
                    n127 = case shown="True" w163 {
                      tunnel: w159 -> [w164 w166]
                      tunnel: [w164 w165] -> w157
                      frame False {
                      }
                      frame True {
                        n128 = Increment(x=w166) -> (x+1=w165:dbl)
                      }
                    }
                    n129 = Multiply(x=w157, y=w160) -> (x*y=w161:dbl)
                    n130 = Divide(x=w161, y=60.0) -> (x/y=w156:dbl)
                    n131 = Bundle(cluster=w158, "CYCLE"=w157, "MINS"=w156) -> (w155:T4)  [unwired: 1 in]
                    n132 = local write "LAB01-1 (DISP)"(w155) -> ()
                  }
                  frame #1 {
                    # "update cycle value"
                    # "LAB01-2"
                    n133 = local read "LAB01-2 (DISP)"() -> (w170:T4)
                    n134 = Unbundle(w170) -> ("CYCLE"=w171:dbl)  [unwired: 2 out]
                    n135 = case shown="True" w175 {
                      tunnel: w171 -> [w176 w178]
                      tunnel: [w176 w177] -> w168
                      frame False {
                      }
                      frame True {
                        n136 = Increment(x=w178) -> (x+1=w177:dbl)
                      }
                    }
                    n137 = Multiply(x=w168, y=w172) -> (x*y=w173:dbl)
                    n138 = Divide(x=w173, y=60.0) -> (x/y=w167:dbl)
                    n139 = Bundle(cluster=w170, "CYCLE"=w168, "MINS"=w167) -> (w169:T4)  [unwired: 1 in]
                    n140 = local write "LAB01-2 (DISP)"(w169) -> ()
                  }
                  frame #2 {
                    # "update cycle value"
                    # "LAB02-1"
                    n141 = local read "LAB02-1 (DISP)"() -> (w182:T4)
                    n142 = Unbundle(w182) -> ("CYCLE"=w183:dbl)  [unwired: 2 out]
                    n143 = case shown="True" w187 {
                      tunnel: [w188 w190] -> w180
                      tunnel: w183 -> [w188 w189]
                      frame False {
                      }
                      frame True {
                        n144 = Increment(x=w189) -> (x+1=w190:dbl)
                      }
                    }
                    n145 = Multiply(x=w180, y=w184) -> (x*y=w185:dbl)
                    n146 = Divide(x=w185, y=60.0) -> (x/y=w179:dbl)
                    n147 = Bundle(cluster=w182, "CYCLE"=w180, "MINS"=w179) -> (w181:T4)  [unwired: 1 in]
                    n148 = local write "LAB02-1 (DISP)"(w181) -> ()
                  }
                  frame #3 {
                    # "update cycle value"
                    # "LAB02-2"
                    n149 = local read "LAB02-2 (DISP)"() -> (w194:T4)
                    n150 = Unbundle(w194) -> ("CYCLE"=w195:dbl)  [unwired: 2 out]
                    n151 = case shown="True" w199 {
                      tunnel: [w200 w202] -> w193
                      tunnel: w195 -> [w200 w201]
                      frame False {
                      }
                      frame True {
                        n152 = Increment(x=w201) -> (x+1=w202:dbl)
                      }
                    }
                    n153 = Multiply(x=w193, y=w196) -> (x*y=w197:dbl)
                    n154 = Divide(x=w197, y=60.0) -> (x/y=w192:dbl)
                    n155 = Bundle(cluster=w194, "CYCLE"=w193, "MINS"=w192) -> (w191:T4)  [unwired: 1 in]
                    n156 = local write "LAB02-2 (DISP)"(w191) -> ()
                  }
                  frame #4 {
                    # "update cycle value"
                    # "LAB03-1"
                    n157 = local read "LAB03-1 (DISP)"() -> (w206:T4)
                    n158 = Unbundle(w206) -> ("CYCLE"=w207:dbl)  [unwired: 2 out]
                    n159 = case shown="True" w211 {
                      tunnel: [w212 w214] -> w203
                      tunnel: w207 -> [w212 w213]
                      frame False {
                      }
                      frame True {
                        n160 = Increment(x=w213) -> (x+1=w214:dbl)
                      }
                    }
                    n161 = Multiply(x=w203, y=w208) -> (x*y=w209:dbl)
                    n162 = Divide(x=w209, y=60.0) -> (x/y=w204:dbl)
                    n163 = Bundle(cluster=w206, "CYCLE"=w203, "MINS"=w204) -> (w205:T4)  [unwired: 1 in]
                    n164 = local write "LAB03-1 (DISP)"(w205) -> ()
                  }
                  frame #5 {
                    # "update cycle value"
                    # "LAB03-2"
                    n165 = local read "LAB03-2 (DISP)"() -> (w218:T4)
                    n166 = Unbundle(w218) -> ("CYCLE"=w219:dbl)  [unwired: 2 out]
                    n167 = case shown="False" w223 {
                      tunnel: [w224 w226] -> w217
                      tunnel: w219 -> [w224 w225]
                      frame False {
                      }
                      frame True {
                        n168 = Increment(x=w225) -> (x+1=w226:dbl)
                      }
                    }
                    n169 = Multiply(x=w217, y=w220) -> (x*y=w221:dbl)
                    n170 = Divide(x=w221, y=60.0) -> (x/y=w216:dbl)
                    n171 = Bundle(cluster=w218, "CYCLE"=w217, "MINS"=w216) -> (w215:T4)  [unwired: 1 in]
                    n172 = local write "LAB03-2 (DISP)"(w215) -> ()
                  }
                  frame #6 {
                    # "update cycle value"
                    # "LAB04-1"
                    n173 = local read "LAB04-1 (DISP)"() -> (w230:T4)
                    n174 = Unbundle(w230) -> ("CYCLE"=w231:dbl)  [unwired: 2 out]
                    n175 = case shown="True" w235 {
                      tunnel: [w236 w238] -> w228
                      tunnel: w231 -> [w236 w237]
                      frame False {
                      }
                      frame True {
                        n176 = Increment(x=w237) -> (x+1=w238:dbl)
                      }
                    }
                    n177 = Multiply(x=w228, y=w232) -> (x*y=w233:dbl)
                    n178 = Divide(x=w233, y=60.0) -> (x/y=w227:dbl)
                    n179 = Bundle(cluster=w230, "CYCLE"=w228, "MINS"=w227) -> (w229:T4)  [unwired: 1 in]
                    n180 = local write "LAB04-1 (DISP)"(w229) -> ()
                  }
                  frame #7 {
                    # "update cycle value"
                    # "LAB04-2"
                    n181 = local read "LAB04-2 (DISP)"() -> (w242:T4)
                    n182 = Unbundle(w242) -> ("CYCLE"=w243:dbl)  [unwired: 2 out]
                    n183 = case shown="True" w247 {
                      tunnel: [w248 w250] -> w240
                      tunnel: w243 -> [w248 w249]
                      frame False {
                      }
                      frame True {
                        n184 = Increment(x=w249) -> (x+1=w250:dbl)
                      }
                    }
                    n185 = Multiply(x=w240, y=w244) -> (x*y=w246:dbl)
                    n186 = Divide(x=w246, y=60.0) -> (x/y=w239:dbl)
                    n187 = Bundle(cluster=w242, "CYCLE"=w240, "MINS"=w239) -> (w241:T4)  [unwired: 1 in]
                    n188 = local write "LAB04-2 (DISP)"(w241) -> ()
                  }
                  frame #8 {
                    # "update cycle value"
                    # "LAB05-1"
                    n189 = local read "LAB05-1 (DISP)"() -> (w254:T4)
                    n190 = Unbundle(w254) -> ("CYCLE"=w255:dbl)  [unwired: 2 out]
                    n191 = case shown="True" w259 {
                      tunnel: [w260 w262] -> w252
                      tunnel: w255 -> [w260 w261]
                      frame False {
                      }
                      frame True {
                        n192 = Increment(x=w261) -> (x+1=w262:dbl)
                      }
                    }
                    n193 = Multiply(x=w252, y=w256) -> (x*y=w257:dbl)
                    n194 = Divide(x=w257, y=60.0) -> (x/y=w251:dbl)
                    n195 = Bundle(cluster=w254, "CYCLE"=w252, "MINS"=w251) -> (w253:T4)  [unwired: 1 in]
                    n196 = local write "LAB05-1 (DISP)"(w253) -> ()
                  }
                  frame #9 {
                    # "update cycle value"
                    # "LAB05-2"
                    n197 = local read "LAB05-2 (DISP)"() -> (w267:T4)
                    n198 = Unbundle(w267) -> ("CYCLE"=w266:dbl)  [unwired: 2 out]
                    n199 = case shown="True" w271 {
                      tunnel: [w272 w274] -> w265
                      tunnel: w266 -> [w272 w273]
                      frame False {
                      }
                      frame True {
                        n200 = Increment(x=w273) -> (x+1=w274:dbl)
                      }
                    }
                    n201 = Multiply(x=w265, y=w268) -> (x*y=w269:dbl)
                    n202 = Divide(x=w269, y=60.0) -> (x/y=w264:dbl)
                    n203 = Bundle(cluster=w267, "CYCLE"=w265, "MINS"=w264) -> (w263:T4)  [unwired: 1 in]
                    n204 = local write "LAB05-2 (DISP)"(w263) -> ()
                  }
                }
                n205 = local write "jig cycle"(0) -> ()
              }
            }
          }
          frame #3 {
            # "START & STOP test RUN switch change, start test if true and stop test if false"
            n206 = Get Date/Time In Seconds() -> (seconds since 1Jan1904=w277:timestamp)
            n207 = Format Date/Time String(time format string (%c)="%b%d", seconds (now)=w277) -> (date/time string=w301:string)  [unwired: 1 in]
            n208 = Format Date/Time String(time format string (%c)="%H%M", seconds (now)=w277) -> (date/time string=w299:string)  [unwired: 1 in]
            n209 = Format Date/Time String(time format string (%c)="%Y", seconds (now)=w277) -> (date/time string=w276:string)  [unwired: 1 in]
            n210 = event shown="[1] \"LAB01-1RUN\": Value Change" {
              selector: _ -> [_ _ _ _ _ _ _ _ _ _ _]
              dyn-events: _ -> [_ _ _ _ _ _ _ _ _ _ _]
              timeout: 10 -> [_ _ _ _ _ _ _ _ _ _ _]
              tunnel: "c:\\crabtree\\Test Data\\" -> [_ w309 w392 w475 w558 w641 w724 w807 w890 w973 w1056]
              tunnel: w301 -> [_ w308 w391 w474 w557 w640 w723 w806 w889 w972 w1055]
              tunnel: w299 -> [_ w306 w390 w473 w556 w639 w722 w805 w888 w971 w1054]
              tunnel: w297 -> [_ w307 _ _ _ _ _ _ _ _ _]
              tunnel: w298 -> [_ _ _ _ _ _ _ _ _ _ _]
              tunnel: w296 -> [_ _ _ _ _ _ _ _ _ _ _]
              tunnel: w295 -> [_ _ w389 _ _ _ _ _ _ _ _]
              tunnel: w294 -> [_ _ _ _ _ _ _ _ _ _ _]
              tunnel: w293 -> [_ _ _ w472 _ _ _ _ _ _ _]
              tunnel: w292 -> [_ _ _ _ _ _ _ _ _ _ _]
              tunnel: w291 -> [_ _ _ _ w555 _ _ _ _ _ _]
              tunnel: w290 -> [_ _ _ _ _ _ _ _ _ _ _]
              tunnel: w289 -> [_ _ _ _ _ w638 _ _ _ _ _]
              tunnel: w288 -> [_ _ _ _ _ _ _ _ _ _ _]
              tunnel: w287 -> [_ _ _ _ _ _ w721 _ _ _ _]
              tunnel: w286 -> [_ _ _ _ _ _ _ _ _ _ _]
              tunnel: w285 -> [_ _ _ _ _ _ _ w804 _ _ _]
              tunnel: w284 -> [_ _ _ _ _ _ _ _ _ _ _]
              tunnel: w283 -> [_ _ _ _ _ _ _ _ w887 _ _]
              tunnel: w282 -> [_ _ _ _ _ _ _ _ _ _ _]
              tunnel: w281 -> [_ _ _ _ _ _ _ _ _ w970 _]
              tunnel: w280 -> [_ _ _ _ _ _ _ _ _ _ _]
              tunnel: w279 -> [_ _ _ _ _ _ _ _ _ _ w1053]
              tunnel: w276 -> [_ w304 w387 w470 w553 w636 w719 w802 w885 w968 w1051]
              event Timeout {
                n211 = event-data() -> ()  [unwired: 1 in, 3 out]
              }
              event "LAB01-1RUN": Value Change {
                n212 = event-data() -> ("NewVal"=w305:bool)  [unwired: 1 in, 5 out]
                n213 = case shown="True" w305 {
                  tunnel: w309 -> [_ w334]
                  tunnel: w308 -> [_ w333]
                  tunnel: w307 -> [w310 w332]
                  tunnel: w306 -> [_ w331]
                  tunnel: w304 -> [_ w330]
                  frame False {
                    # "stop test"
                    n214 = stacked-sequence {
                      tunnel: w310 -> [w316 _]
                      frame #0 {
                        n215 = local read "LAB01-1 (DISP)"() -> (w315:T4)
                        n216 = Unbundle(w315) -> ("CYCLE"=w313:dbl, "MINS"=w314:dbl)  [unwired: 1 out]
                        n217 = case shown="\"CYCLE TEST\"" w316 {
                          tunnel: w314 -> [_ _ w323]
                          tunnel: w313 -> [w321 w322 _]
                          tunnel: [w321 w322 w323] -> w312
                          frame "CHART TEST", Default {
                          }
                          frame "CYCLE TEST" {
                          }
                          frame "T-RISE TEST" {
                          }
                        }
                        n218 = local read "LAB01-1 (TDMS)"() -> (w320:refnum<k34>)
                        n219 = Build Array("STOPPED") -> (w317:string[])
                        n220 = Build Array(w312) -> (w311:dbl[])
                        n221 = TDMS Write(0:w320, 5:"TEST RESULT", 7:w317, 9:w311) -> ()  [unwired: 2 in, 4 out]
                      }
                      frame #1 {
                        n222 = local read "LAB01-1 (DISP)"() -> (w329:T4)
                        n223 = Bundle(cluster=w329, "STATUS"="STOP") -> (w327:T4)  [unwired: 2 in]
                        n224 = call "Save data file to network drive v1.vi"("panel id"="LAB01-1") -> ("network file save error"=w324:errorcluster)  [unwired: 9 in, 1 out]
                        n225 = local write "LAB01-1 (RESULT)"(FALSE) -> ()
                        n226 = local write "LAB01-1 (DISP)"(w327) -> ()
                        n227 = local write "data file error"(w324) -> ()
                      }
                    }
                  }
                  frame True {
                    # "start new test and create test file"
                    n228 = stacked-sequence {
                      seq-local: [w335 _ _ _ _] -> [_ w360 _ _ _]
                      tunnel: w334 -> [w340 _ _ _ _]
                      tunnel: w333 -> [w336 _ _ _ _]
                      tunnel: w332 -> [w350 _ _ _ _]
                      tunnel: w331 -> [w343 _ _ _ _]
                      tunnel: w330 -> [w338 _ _ _ _]
                      frame #0 {
                        w337 = "\\"
                        n229 = local read "LAB01-1 (SET)"() -> (w345:T5)
                        n230 = case shown="\"CHART TEST\", Default" w350 {
                          tunnel: ["CHART TEST-" "CYCLE TEST-" "T-RISE TEST-"] -> w346
                          frame "CHART TEST", Default {
                          }
                          frame "CYCLE TEST" {
                          }
                          frame "T-RISE TEST" {
                          }
                        }
                        n231 = Unbundle(w345) -> ("DESCRIPTION"=w344:string)  [unwired: 4 out]
                        n232 = Concatenate Strings(w340, "LAB01-1\\", w338, w337, w336, w337) -> (w347:string)
                        n233 = String To Path(string=w347) -> (path=w349:path)
                        n234 = Concatenate Strings(w347, w346, w344, "-", w343, ".tdms") -> (w335:string)
                        n235 = Create Folder(path (use dialog)=w349) -> (error out=w348:errorcluster)  [unwired: 2 in, 2 out]
                        n236 = global write "Global 1.vi" "LAB01-1 FILE"(w335) -> ()
                        n237 = call <vilib>:"Clear Errors.vi"("error in (no error)"=w348) -> ()  [unwired: 6 in, 1 out]
                      }
                      frame #1 {
                        n238 = String To Path(string=w360) -> (path=w354:path)
                        n239 = TDMS Open(5:FALSE, 6:FALSE, 10:T14."create or replace" ("operation (0:open)"), 11:w354) -> (0:w356:errorcluster, 3:→"LAB01-1 (TDMS)":refnum<k34>)  [unwired: 3 in]
                        n240 = local write "data file error"(w356) -> ()
                      }
                      frame #2 {
                        n241 = local read "LAB01-1 (SET)"() -> (w366:T5)
                        n242 = local read "LAB01-1 (TDMS)"() -> (w377:refnum<k34>)
                        n243 = Build Array("Testers Name", "Description", "Set Test Cycles", "T-Rise minutes", "T-Rise Deg C") -> (w367:string[])
                        n244 = Unbundle(w366) -> ("NAME"=w365:string, "DESCRIPTION"=w364:string, "CYCLES"=w363:dbl, "T-RISE mins"=w362:dbl, "T-RISE deg C"=w361:dbl)
                        n245 = Number To Decimal String(number=w363) -> (decimal integer string=w376:string)  [unwired: 1 in]
                        n246 = Number To Decimal String(number=w362) -> (decimal integer string=w375:string)  [unwired: 1 in]
                        n247 = Number To Decimal String(number=w361) -> (decimal integer string=w374:string)  [unwired: 1 in]
                        n248 = Build Array(w365, w364, w376, w375, w374) -> (w373:string[])
                        n249 = TDMS Set Properties(5:w373, 7:w367, 11:w377) -> ()  [unwired: 3 in, 4 out]
                      }
                      frame #3 {
                        w378 = 0.0
                        n250 = local read "LAB01-1 (DISP)"() -> (w381:T4)
                        n251 = Bundle(cluster=w381, "CYCLE"=w378, "MINS"=w378, "STATUS"="RUN") -> (w380:T4)
                        n252 = local write "LAB01-1 (DISP)"(w380) -> ()
                      }
                      frame #4 {
                        n253 = local read "LAB01-1 (SIG)"() -> (w384:T2)
                        n254 = local read "LAB01-1 (TEMP START)"() -> (w386:cluster{"TL":dbl, "TN":dbl})
                        n255 = Unbundle(w384) -> ("Tmp Live"=w383:dbl, "Tmp Neut"=w382:dbl)  [unwired: 3 out]
                        n256 = Bundle(cluster=w386, "TL"=w383, "TN"=w382) -> (w385:cluster{"TL":dbl, "TN":dbl})
                        n257 = local write "LAB01-1 (TEMP START)"(w385) -> ()
                      }
                    }
                  }
                }
              }
              event "LAB01-2 RUN": Value Change {
                n258 = event-data() -> ("NewVal"=w388:bool)  [unwired: 1 in, 5 out]
                n259 = case shown="True" w388 {
                  tunnel: w392 -> [_ w417]
                  tunnel: w391 -> [_ w416]
                  tunnel: w389 -> [w393 w415]
                  tunnel: w390 -> [_ w414]
                  tunnel: w387 -> [_ w413]
                  frame False {
                    # "stop test"
                    n260 = stacked-sequence {
                      tunnel: w393 -> [w399 _]
                      frame #0 {
                        n261 = local read "LAB01-2 (DISP)"() -> (w398:T4)
                        n262 = Unbundle(w398) -> ("CYCLE"=w396:dbl, "MINS"=w397:dbl)  [unwired: 1 out]
                        n263 = case shown="\"CHART TEST\", Default" w399 {
                          tunnel: w397 -> [_ _ w406]
                          tunnel: w396 -> [w404 w405 _]
                          tunnel: [w404 w405 w406] -> w395
                          frame "CHART TEST", Default {
                          }
                          frame "CYCLE TEST" {
                          }
                          frame "T-RISE TEST" {
                          }
                        }
                        n264 = local read "LAB01-2 (TDMS)"() -> (w403:refnum<k34>)
                        n265 = Build Array("STOPPED") -> (w400:string[])
                        n266 = Build Array(w395) -> (w394:dbl[])
                        n267 = TDMS Write(0:w403, 5:"TEST RESULT", 7:w400, 9:w394) -> ()  [unwired: 2 in, 4 out]
                      }
                      frame #1 {
                        n268 = local read "LAB01-2 (DISP)"() -> (w412:T4)
                        n269 = Bundle(cluster=w412, "STATUS"="STOP") -> (w410:T4)  [unwired: 2 in]
                        n270 = local write "LAB01-2 (RESULT)"(FALSE) -> ()
                        n271 = call "Save data file to network drive v1.vi"("panel id"="LAB01-2") -> ("network file save error"=w407:errorcluster)  [unwired: 9 in, 1 out]
                        n272 = local write "LAB01-2 (DISP)"(w410) -> ()
                        n273 = local write "data file error"(w407) -> ()
                      }
                    }
                  }
                  frame True {
                    # "start new test and create test file"
                    n274 = stacked-sequence {
                      seq-local: [w418 _ _ _ _] -> [_ w443 _ _ _]
                      tunnel: w417 -> [w423 _ _ _ _]
                      tunnel: w416 -> [w420 _ _ _ _]
                      tunnel: w415 -> [w433 _ _ _ _]
                      tunnel: w414 -> [w426 _ _ _ _]
                      tunnel: w413 -> [w421 _ _ _ _]
                      frame #0 {
                        w419 = "\\"
                        n275 = local read "LAB01-2 (SET)"() -> (w428:T5)
                        n276 = case shown="\"CHART TEST\", Default" w433 {
                          tunnel: ["CHART TEST-" "CYCLE TEST-" "T-RISE TEST-"] -> w429
                          frame "CHART TEST", Default {
                          }
                          frame "CYCLE TEST" {
                          }
                          frame "T-RISE TEST" {
                          }
                        }
                        n277 = Unbundle(w428) -> ("DESCRIPTION"=w427:string)  [unwired: 4 out]
                        n278 = Concatenate Strings(w423, "LAB01-2\\", w421, w419, w420, w419) -> (w430:string)
                        n279 = String To Path(string=w430) -> (path=w432:path)
                        n280 = Concatenate Strings(w430, w429, w427, "-", w426, ".tdms") -> (w418:string)
                        n281 = Create Folder(path (use dialog)=w432) -> (error out=w431:errorcluster)  [unwired: 2 in, 2 out]
                        n282 = global write "Global 1.vi" "LAB01-2 FILE"(w418) -> ()
                        n283 = call <vilib>:"Clear Errors.vi"("error in (no error)"=w431) -> ()  [unwired: 6 in, 1 out]
                      }
                      frame #1 {
                        n284 = String To Path(string=w443) -> (path=w437:path)
                        n285 = TDMS Open(5:FALSE, 6:FALSE, 10:T14."create or replace" ("operation (0:open)"), 11:w437) -> (0:w439:errorcluster, 3:→"LAB01-2 (TDMS)":refnum<k34>)  [unwired: 3 in]
                        n286 = local write "data file error"(w439) -> ()
                      }
                      frame #2 {
                        n287 = local read "LAB01-2 (SET)"() -> (w449:T5)
                        n288 = local read "LAB01-2 (TDMS)"() -> (w460:refnum<k34>)
                        n289 = Build Array("Testers Name", "Description", "Set Test Cycles", "T-Rise minutes", "T-Rise Deg C") -> (w450:string[])
                        n290 = Unbundle(w449) -> ("NAME"=w448:string, "DESCRIPTION"=w447:string, "CYCLES"=w446:dbl, "T-RISE mins"=w445:dbl, "T-RISE deg C"=w444:dbl)
                        n291 = Number To Decimal String(number=w446) -> (decimal integer string=w459:string)  [unwired: 1 in]
                        n292 = Number To Decimal String(number=w445) -> (decimal integer string=w458:string)  [unwired: 1 in]
                        n293 = Number To Decimal String(number=w444) -> (decimal integer string=w457:string)  [unwired: 1 in]
                        n294 = Build Array(w448, w447, w459, w458, w457) -> (w456:string[])
                        n295 = TDMS Set Properties(5:w456, 7:w450, 11:w460) -> ()  [unwired: 3 in, 4 out]
                      }
                      frame #3 {
                        w462 = 0.0
                        n296 = local read "LAB01-2 (DISP)"() -> (w464:T4)
                        n297 = Bundle(cluster=w464, "CYCLE"=w462, "MINS"=w462, "STATUS"="RUN") -> (w463:T4)
                        n298 = local write "LAB01-2 (DISP)"(w463) -> ()
                      }
                      frame #4 {
                        n299 = local read "LAB01-2 (SIG)"() -> (w467:T2)
                        n300 = local read "LAB01-2 (TEMP START)"() -> (w469:cluster{"TL":dbl, "TN":dbl})
                        n301 = Unbundle(w467) -> ("Tmp Live"=w466:dbl, "Tmp Neut"=w465:dbl)  [unwired: 3 out]
                        n302 = Bundle(cluster=w469, "TL"=w466, "TN"=w465) -> (w468:cluster{"TL":dbl, "TN":dbl})
                        n303 = local write "LAB01-2 (TEMP START)"(w468) -> ()
                      }
                    }
                  }
                }
              }
              event "LAB02-1 RUN": Value Change {
                n304 = event-data() -> ("NewVal"=w471:bool)  [unwired: 1 in, 5 out]
                n305 = case shown="True" w471 {
                  tunnel: w475 -> [_ w500]
                  tunnel: w474 -> [_ w499]
                  tunnel: w472 -> [w476 w498]
                  tunnel: w473 -> [_ w497]
                  tunnel: w470 -> [_ w496]
                  frame False {
                    # "stop test"
                    n306 = stacked-sequence {
                      tunnel: w476 -> [w482 _]
                      frame #0 {
                        n307 = local read "LAB02-1 (DISP)"() -> (w481:T4)
                        n308 = Unbundle(w481) -> ("CYCLE"=w479:dbl, "MINS"=w480:dbl)  [unwired: 1 out]
                        n309 = case shown="\"CYCLE TEST\"" w482 {
                          tunnel: w480 -> [_ _ w489]
                          tunnel: w479 -> [w487 w488 _]
                          tunnel: [w487 w488 w489] -> w478
                          frame "CHART TEST", Default {
                          }
                          frame "CYCLE TEST" {
                          }
                          frame "T-RISE TEST" {
                          }
                        }
                        n310 = local read "LAB02-1 (TDMS)"() -> (w486:refnum<k34>)
                        n311 = Build Array("STOPPED") -> (w483:string[])
                        n312 = Build Array(w478) -> (w477:dbl[])
                        n313 = TDMS Write(0:w486, 5:"TEST RESULT", 7:w483, 9:w477) -> ()  [unwired: 2 in, 4 out]
                      }
                      frame #1 {
                        n314 = local read "LAB02-1 (DISP)"() -> (w495:T4)
                        n315 = Bundle(cluster=w495, "STATUS"="STOP") -> (w493:T4)  [unwired: 2 in]
                        n316 = local write "LAB02-1 (RESULT)"(FALSE) -> ()
                        n317 = local write "LAB02-1 (DISP)"(w493) -> ()
                        n318 = call "Save data file to network drive v1.vi"("panel id"="LAB02-1") -> ("network file save error"=w490:errorcluster)  [unwired: 9 in, 1 out]
                        n319 = local write "data file error"(w490) -> ()
                      }
                    }
                  }
                  frame True {
                    # "start new test and create test file"
                    n320 = stacked-sequence {
                      seq-local: [w501 _ _ _ _] -> [_ w526 _ _ _]
                      tunnel: w500 -> [w506 _ _ _ _]
                      tunnel: w499 -> [w503 _ _ _ _]
                      tunnel: w498 -> [w516 _ _ _ _]
                      tunnel: w497 -> [w509 _ _ _ _]
                      tunnel: w496 -> [w504 _ _ _ _]
                      frame #0 {
                        w502 = "\\"
                        n321 = local read "LAB02-1 (SET)"() -> (w511:T5)
                        n322 = case shown="\"CHART TEST\", Default" w516 {
                          tunnel: ["CHART TEST-" "CYCLE TEST-" "T-RISE TEST-"] -> w512
                          frame "CHART TEST", Default {
                          }
                          frame "CYCLE TEST" {
                          }
                          frame "T-RISE TEST" {
                          }
                        }
                        n323 = Unbundle(w511) -> ("DESCRIPTION"=w510:string)  [unwired: 4 out]
                        n324 = Concatenate Strings(w506, "LAB02-1\\", w504, w502, w503, w502) -> (w513:string)
                        n325 = String To Path(string=w513) -> (path=w515:path)
                        n326 = Concatenate Strings(w513, w512, w510, "-", w509, ".tdms") -> (w501:string)
                        n327 = Create Folder(path (use dialog)=w515) -> (error out=w514:errorcluster)  [unwired: 2 in, 2 out]
                        n328 = global write "Global 1.vi" "LAB02-1 FILE"(w501) -> ()
                        n329 = call <vilib>:"Clear Errors.vi"("error in (no error)"=w514) -> ()  [unwired: 6 in, 1 out]
                      }
                      frame #1 {
                        n330 = String To Path(string=w526) -> (path=w520:path)
                        n331 = TDMS Open(5:FALSE, 6:FALSE, 10:T14."create or replace" ("operation (0:open)"), 11:w520) -> (0:w522:errorcluster, 3:→"LAB02-1 (TDMS)":refnum<k34>)  [unwired: 3 in]
                        n332 = local write "data file error"(w522) -> ()
                      }
                      frame #2 {
                        n333 = local read "LAB02-1 (SET)"() -> (w532:T5)
                        n334 = local read "LAB02-1 (TDMS)"() -> (w543:refnum<k34>)
                        n335 = Build Array("Testers Name", "Description", "Set Test Cycles", "T-Rise minutes", "T-Rise Deg C") -> (w533:string[])
                        n336 = Unbundle(w532) -> ("NAME"=w531:string, "DESCRIPTION"=w530:string, "CYCLES"=w529:dbl, "T-RISE mins"=w528:dbl, "T-RISE deg C"=w527:dbl)
                        n337 = Number To Decimal String(number=w529) -> (decimal integer string=w542:string)  [unwired: 1 in]
                        n338 = Number To Decimal String(number=w528) -> (decimal integer string=w541:string)  [unwired: 1 in]
                        n339 = Number To Decimal String(number=w527) -> (decimal integer string=w540:string)  [unwired: 1 in]
                        n340 = Build Array(w531, w530, w542, w541, w540) -> (w539:string[])
                        n341 = TDMS Set Properties(5:w539, 7:w533, 11:w543) -> ()  [unwired: 3 in, 4 out]
                      }
                      frame #3 {
                        w545 = 0.0
                        n342 = local read "LAB02-1 (DISP)"() -> (w547:T4)
                        n343 = Bundle(cluster=w547, "CYCLE"=w545, "MINS"=w545, "STATUS"="RUN") -> (w546:T4)
                        n344 = local write "LAB02-1 (DISP)"(w546) -> ()
                      }
                      frame #4 {
                        n345 = local read "LAB02-1 (SIG)"() -> (w550:T2)
                        n346 = local read "LAB02-1 (TEMP START)"() -> (w552:cluster{"TL":dbl, "TN":dbl})
                        n347 = Unbundle(w550) -> ("Tmp Live"=w549:dbl, "Tmp Neut"=w548:dbl)  [unwired: 3 out]
                        n348 = Bundle(cluster=w552, "TL"=w549, "TN"=w548) -> (w551:cluster{"TL":dbl, "TN":dbl})
                        n349 = local write "LAB02-1 (TEMP START)"(w551) -> ()
                      }
                    }
                  }
                }
              }
              event "LAB02-2 RUN": Value Change {
                n350 = event-data() -> ("NewVal"=w554:bool)  [unwired: 1 in, 5 out]
                n351 = case shown="True" w554 {
                  tunnel: w558 -> [_ w583]
                  tunnel: w557 -> [_ w582]
                  tunnel: w555 -> [w559 w581]
                  tunnel: w556 -> [_ w580]
                  tunnel: w553 -> [_ w579]
                  frame False {
                    # "stop test"
                    n352 = stacked-sequence {
                      tunnel: w559 -> [w565 _]
                      frame #0 {
                        n353 = local read "LAB02-2 (DISP)"() -> (w564:T4)
                        n354 = Unbundle(w564) -> ("CYCLE"=w562:dbl, "MINS"=w563:dbl)  [unwired: 1 out]
                        n355 = case shown="\"CYCLE TEST\"" w565 {
                          tunnel: w563 -> [_ _ w572]
                          tunnel: w562 -> [w570 w571 _]
                          tunnel: [w570 w571 w572] -> w561
                          frame "CHART TEST", Default {
                          }
                          frame "CYCLE TEST" {
                          }
                          frame "T-RISE TEST" {
                          }
                        }
                        n356 = local read "LAB02-2 (TDMS)"() -> (w569:refnum<k34>)
                        n357 = Build Array("STOPPED") -> (w566:string[])
                        n358 = Build Array(w561) -> (w560:dbl[])
                        n359 = TDMS Write(0:w569, 5:"TEST RESULT", 7:w566, 9:w560) -> ()  [unwired: 2 in, 4 out]
                      }
                      frame #1 {
                        n360 = local read "LAB02-2 (DISP)"() -> (w578:T4)
                        n361 = Bundle(cluster=w578, "STATUS"="STOP") -> (w576:T4)  [unwired: 2 in]
                        n362 = local write "LAB02-2 (RESULT)"(FALSE) -> ()
                        n363 = call "Save data file to network drive v1.vi"("panel id"="LAB02-2") -> ("network file save error"=w573:errorcluster)  [unwired: 9 in, 1 out]
                        n364 = local write "LAB02-2 (DISP)"(w576) -> ()
                        n365 = local write "data file error"(w573) -> ()
                      }
                    }
                  }
                  frame True {
                    # "start new test and create test file"
                    n366 = stacked-sequence {
                      seq-local: [w584 _ _ _ _] -> [_ w609 _ _ _]
                      tunnel: w583 -> [w589 _ _ _ _]
                      tunnel: w582 -> [w586 _ _ _ _]
                      tunnel: w581 -> [w599 _ _ _ _]
                      tunnel: w580 -> [w592 _ _ _ _]
                      tunnel: w579 -> [w587 _ _ _ _]
                      frame #0 {
                        w585 = "\\"
                        n367 = local read "LAB02-2 (SET)"() -> (w594:T5)
                        n368 = case shown="\"CHART TEST\", Default" w599 {
                          tunnel: ["CHART TEST-" "CYCLE TEST-" "T-RISE TEST-"] -> w595
                          frame "CHART TEST", Default {
                          }
                          frame "CYCLE TEST" {
                          }
                          frame "T-RISE TEST" {
                          }
                        }
                        n369 = Unbundle(w594) -> ("DESCRIPTION"=w593:string)  [unwired: 4 out]
                        n370 = Concatenate Strings(w589, "LAB02-2\\", w587, w585, w586, w585) -> (w596:string)
                        n371 = String To Path(string=w596) -> (path=w598:path)
                        n372 = Concatenate Strings(w596, w595, w593, "-", w592, ".tdms") -> (w584:string)
                        n373 = Create Folder(path (use dialog)=w598) -> (error out=w597:errorcluster)  [unwired: 2 in, 2 out]
                        n374 = global write "Global 1.vi" "LAB02-2 FILE"(w584) -> ()
                        n375 = call <vilib>:"Clear Errors.vi"("error in (no error)"=w597) -> ()  [unwired: 6 in, 1 out]
                      }
                      frame #1 {
                        n376 = String To Path(string=w609) -> (path=w603:path)
                        n377 = TDMS Open(5:FALSE, 6:FALSE, 10:T14."create or replace" ("operation (0:open)"), 11:w603) -> (0:w605:errorcluster, 3:→"LAB02-2 (TDMS)":refnum<k34>)  [unwired: 3 in]
                        n378 = local write "data file error"(w605) -> ()
                      }
                      frame #2 {
                        n379 = local read "LAB02-2 (SET)"() -> (w615:T5)
                        n380 = local read "LAB02-2 (TDMS)"() -> (w626:refnum<k34>)
                        n381 = Build Array("Testers Name", "Description", "Set Test Cycles", "T-Rise minutes", "T-Rise Deg C") -> (w616:string[])
                        n382 = Unbundle(w615) -> ("NAME"=w614:string, "DESCRIPTION"=w613:string, "CYCLES"=w612:dbl, "T-RISE mins"=w611:dbl, "T-RISE deg C"=w610:dbl)
                        n383 = Number To Decimal String(number=w612) -> (decimal integer string=w625:string)  [unwired: 1 in]
                        n384 = Number To Decimal String(number=w611) -> (decimal integer string=w624:string)  [unwired: 1 in]
                        n385 = Number To Decimal String(number=w610) -> (decimal integer string=w623:string)  [unwired: 1 in]
                        n386 = Build Array(w614, w613, w625, w624, w623) -> (w622:string[])
                        n387 = TDMS Set Properties(5:w622, 7:w616, 11:w626) -> ()  [unwired: 3 in, 4 out]
                      }
                      frame #3 {
                        w628 = 0.0
                        n388 = local read "LAB02-2 (DISP)"() -> (w630:T4)
                        n389 = Bundle(cluster=w630, "CYCLE"=w628, "MINS"=w628, "STATUS"="RUN") -> (w629:T4)
                        n390 = local write "LAB02-2 (DISP)"(w629) -> ()
                      }
                      frame #4 {
                        n391 = local read "LAB02-2 (SIG)"() -> (w633:T2)
                        n392 = local read "LAB02-2 (TEMP START)"() -> (w635:cluster{"TL":dbl, "TN":dbl})
                        n393 = Unbundle(w633) -> ("Tmp Live"=w632:dbl, "Tmp Neut"=w631:dbl)  [unwired: 3 out]
                        n394 = Bundle(cluster=w635, "TL"=w632, "TN"=w631) -> (w634:cluster{"TL":dbl, "TN":dbl})
                        n395 = local write "LAB02-2 (TEMP START)"(w634) -> ()
                      }
                    }
                  }
                }
              }
              event "LAB03-1 RUN": Value Change {
                n396 = event-data() -> ("NewVal"=w637:bool)  [unwired: 1 in, 5 out]
                n397 = case shown="True" w637 {
                  tunnel: w641 -> [_ w666]
                  tunnel: w640 -> [_ w665]
                  tunnel: w638 -> [w642 w664]
                  tunnel: w639 -> [_ w663]
                  tunnel: w636 -> [_ w662]
                  frame False {
                    # "stop test"
                    n398 = stacked-sequence {
                      tunnel: w642 -> [w648 _]
                      frame #0 {
                        n399 = local read "LAB03-1 (DISP)"() -> (w647:T4)
                        n400 = Unbundle(w647) -> ("CYCLE"=w645:dbl, "MINS"=w646:dbl)  [unwired: 1 out]
                        n401 = case shown="\"CYCLE TEST\"" w648 {
                          tunnel: w646 -> [_ _ w655]
                          tunnel: w645 -> [w653 w654 _]
                          tunnel: [w653 w654 w655] -> w644
                          frame "CHART TEST", Default {
                          }
                          frame "CYCLE TEST" {
                          }
                          frame "T-RISE TEST" {
                          }
                        }
                        n402 = local read "LAB03-1 (TDMS)"() -> (w652:refnum<k34>)
                        n403 = Build Array("STOPPED") -> (w649:string[])
                        n404 = Build Array(w644) -> (w643:dbl[])
                        n405 = TDMS Write(0:w652, 5:"TEST RESULT", 7:w649, 9:w643) -> ()  [unwired: 2 in, 4 out]
                      }
                      frame #1 {
                        n406 = local read "LAB03-1 (DISP)"() -> (w661:T4)
                        n407 = Bundle(cluster=w661, "STATUS"="STOP") -> (w659:T4)  [unwired: 2 in]
                        n408 = call "Save data file to network drive v1.vi"("panel id"="LAB03-1") -> ("network file save error"=w656:errorcluster)  [unwired: 9 in, 1 out]
                        n409 = local write "LAB03-1 (RESULT)"(FALSE) -> ()
                        n410 = local write "LAB03-1 (DISP)"(w659) -> ()
                        n411 = local write "data file error"(w656) -> ()
                      }
                    }
                  }
                  frame True {
                    # "start new test and create test file"
                    n412 = stacked-sequence {
                      seq-local: [w667 _ _ _ _] -> [_ w692 _ _ _]
                      tunnel: w666 -> [w672 _ _ _ _]
                      tunnel: w665 -> [w669 _ _ _ _]
                      tunnel: w664 -> [w682 _ _ _ _]
                      tunnel: w663 -> [w675 _ _ _ _]
                      tunnel: w662 -> [w670 _ _ _ _]
                      frame #0 {
                        w668 = "\\"
                        n413 = local read "LAB03-1 (SET)"() -> (w677:T5)
                        n414 = case shown="\"CHART TEST\", Default" w682 {
                          tunnel: ["CHART TEST-" "CYCLE TEST-" "T-RISE TEST-"] -> w678
                          frame "CHART TEST", Default {
                          }
                          frame "CYCLE TEST" {
                          }
                          frame "T-RISE TEST" {
                          }
                        }
                        n415 = Unbundle(w677) -> ("DESCRIPTION"=w676:string)  [unwired: 4 out]
                        n416 = Concatenate Strings(w672, "LAB03-1\\", w670, w668, w669, w668) -> (w679:string)
                        n417 = String To Path(string=w679) -> (path=w681:path)
                        n418 = Concatenate Strings(w679, w678, w676, "-", w675, ".tdms") -> (w667:string)
                        n419 = Create Folder(path (use dialog)=w681) -> (error out=w680:errorcluster)  [unwired: 2 in, 2 out]
                        n420 = global write "Global 1.vi" "LAB03-1 FILE"(w667) -> ()
                        n421 = call <vilib>:"Clear Errors.vi"("error in (no error)"=w680) -> ()  [unwired: 6 in, 1 out]
                      }
                      frame #1 {
                        n422 = String To Path(string=w692) -> (path=w686:path)
                        n423 = TDMS Open(5:FALSE, 6:FALSE, 10:T14."create or replace" ("operation (0:open)"), 11:w686) -> (0:w688:errorcluster, 3:→"LAB03-1 (TDMS)":refnum<k34>)  [unwired: 3 in]
                        n424 = local write "data file error"(w688) -> ()
                      }
                      frame #2 {
                        n425 = local read "LAB03-1 (SET)"() -> (w698:T5)
                        n426 = local read "LAB03-1 (TDMS)"() -> (w709:refnum<k34>)
                        n427 = Build Array("Testers Name", "Description", "Set Test Cycles", "T-Rise minutes", "T-Rise Deg C") -> (w699:string[])
                        n428 = Unbundle(w698) -> ("NAME"=w697:string, "DESCRIPTION"=w696:string, "CYCLES"=w695:dbl, "T-RISE mins"=w694:dbl, "T-RISE deg C"=w693:dbl)
                        n429 = Number To Decimal String(number=w695) -> (decimal integer string=w708:string)  [unwired: 1 in]
                        n430 = Number To Decimal String(number=w694) -> (decimal integer string=w707:string)  [unwired: 1 in]
                        n431 = Number To Decimal String(number=w693) -> (decimal integer string=w706:string)  [unwired: 1 in]
                        n432 = Build Array(w697, w696, w708, w707, w706) -> (w705:string[])
                        n433 = TDMS Set Properties(5:w705, 7:w699, 11:w709) -> ()  [unwired: 3 in, 4 out]
                      }
                      frame #3 {
                        w711 = 0.0
                        n434 = local read "LAB03-1 (DISP)"() -> (w713:T4)
                        n435 = Bundle(cluster=w713, "CYCLE"=w711, "MINS"=w711, "STATUS"="RUN") -> (w712:T4)
                        n436 = local write "LAB03-1 (DISP)"(w712) -> ()
                      }
                      frame #4 {
                        n437 = local read "LAB03-1 (SIG)"() -> (w716:T2)
                        n438 = local read "LAB03-1 (TEMP START)"() -> (w718:cluster{"TL":dbl, "TN":dbl})
                        n439 = Unbundle(w716) -> ("Tmp Live"=w715:dbl, "Tmp Neut"=w714:dbl)  [unwired: 3 out]
                        n440 = Bundle(cluster=w718, "TL"=w715, "TN"=w714) -> (w717:cluster{"TL":dbl, "TN":dbl})
                        n441 = local write "LAB03-1 (TEMP START)"(w717) -> ()
                      }
                    }
                  }
                }
              }
              event "LAB03-2 RUN": Value Change {
                n442 = event-data() -> ("NewVal"=w720:bool)  [unwired: 1 in, 5 out]
                n443 = case shown="True" w720 {
                  tunnel: w724 -> [_ w749]
                  tunnel: w723 -> [_ w748]
                  tunnel: w721 -> [w725 w747]
                  tunnel: w722 -> [_ w746]
                  tunnel: w719 -> [_ w745]
                  frame False {
                    # "stop test"
                    n444 = stacked-sequence {
                      tunnel: w725 -> [w731 _]
                      frame #0 {
                        n445 = local read "LAB03-2 (DISP)"() -> (w730:T4)
                        n446 = Unbundle(w730) -> ("CYCLE"=w728:dbl, "MINS"=w729:dbl)  [unwired: 1 out]
                        n447 = case shown="\"CYCLE TEST\"" w731 {
                          tunnel: w729 -> [_ _ w738]
                          tunnel: w728 -> [w736 w737 _]
                          tunnel: [w736 w737 w738] -> w727
                          frame "CHART TEST", Default {
                          }
                          frame "CYCLE TEST" {
                          }
                          frame "T-RISE TEST" {
                          }
                        }
                        n448 = local read "LAB03-2 (TDMS)"() -> (w735:refnum<k34>)
                        n449 = Build Array("STOPPED") -> (w732:string[])
                        n450 = Build Array(w727) -> (w726:dbl[])
                        n451 = TDMS Write(0:w735, 5:"TEST RESULT", 7:w732, 9:w726) -> ()  [unwired: 2 in, 4 out]
                      }
                      frame #1 {
                        n452 = local read "LAB03-2 (DISP)"() -> (w744:T4)
                        n453 = Bundle(cluster=w744, "STATUS"="STOP") -> (w742:T4)  [unwired: 2 in]
                        n454 = call "Save data file to network drive v1.vi"("panel id"="LAB03-2") -> ("network file save error"=w739:errorcluster)  [unwired: 9 in, 1 out]
                        n455 = local write "LAB03-2 (RESULT)"(FALSE) -> ()
                        n456 = local write "LAB03-2 (DISP)"(w742) -> ()
                        n457 = local write "data file error"(w739) -> ()
                      }
                    }
                  }
                  frame True {
                    # "start new test and create test file"
                    n458 = stacked-sequence {
                      seq-local: [w750 _ _ _ _] -> [_ w775 _ _ _]
                      tunnel: w749 -> [w755 _ _ _ _]
                      tunnel: w748 -> [w752 _ _ _ _]
                      tunnel: w747 -> [w765 _ _ _ _]
                      tunnel: w746 -> [w758 _ _ _ _]
                      tunnel: w745 -> [w753 _ _ _ _]
                      frame #0 {
                        w751 = "\\"
                        n459 = local read "LAB03-2 (SET)"() -> (w760:T5)
                        n460 = case shown="\"CHART TEST\", Default" w765 {
                          tunnel: ["CHART TEST-" "CYCLE TEST-" "T-RISE TEST-"] -> w761
                          frame "CHART TEST", Default {
                          }
                          frame "CYCLE TEST" {
                          }
                          frame "T-RISE TEST" {
                          }
                        }
                        n461 = Unbundle(w760) -> ("DESCRIPTION"=w759:string)  [unwired: 4 out]
                        n462 = Concatenate Strings(w755, "LAB03-2\\", w753, w751, w752, w751) -> (w762:string)
                        n463 = String To Path(string=w762) -> (path=w764:path)
                        n464 = Concatenate Strings(w762, w761, w759, "-", w758, ".tdms") -> (w750:string)
                        n465 = Create Folder(path (use dialog)=w764) -> (error out=w763:errorcluster)  [unwired: 2 in, 2 out]
                        n466 = global write "Global 1.vi" "LAB03-2 FILE"(w750) -> ()
                        n467 = call <vilib>:"Clear Errors.vi"("error in (no error)"=w763) -> ()  [unwired: 6 in, 1 out]
                      }
                      frame #1 {
                        n468 = String To Path(string=w775) -> (path=w769:path)
                        n469 = TDMS Open(5:FALSE, 6:FALSE, 10:T14."create or replace" ("operation (0:open)"), 11:w769) -> (0:w771:errorcluster, 3:→"LAB03-2 (TDMS)":refnum<k34>)  [unwired: 3 in]
                        n470 = local write "data file error"(w771) -> ()
                      }
                      frame #2 {
                        n471 = local read "LAB03-2 (SET)"() -> (w781:T5)
                        n472 = local read "LAB03-2 (TDMS)"() -> (w792:refnum<k34>)
                        n473 = Build Array("Testers Name", "Description", "Set Test Cycles", "T-Rise minutes", "T-Rise Deg C") -> (w782:string[])
                        n474 = Unbundle(w781) -> ("NAME"=w780:string, "DESCRIPTION"=w779:string, "CYCLES"=w778:dbl, "T-RISE mins"=w777:dbl, "T-RISE deg C"=w776:dbl)
                        n475 = Number To Decimal String(number=w778) -> (decimal integer string=w791:string)  [unwired: 1 in]
                        n476 = Number To Decimal String(number=w777) -> (decimal integer string=w790:string)  [unwired: 1 in]
                        n477 = Number To Decimal String(number=w776) -> (decimal integer string=w789:string)  [unwired: 1 in]
                        n478 = Build Array(w780, w779, w791, w790, w789) -> (w788:string[])
                        n479 = TDMS Set Properties(5:w788, 7:w782, 11:w792) -> ()  [unwired: 3 in, 4 out]
                      }
                      frame #3 {
                        w794 = 0.0
                        n480 = local read "LAB03-2 (DISP)"() -> (w796:T4)
                        n481 = Bundle(cluster=w796, "CYCLE"=w794, "MINS"=w794, "STATUS"="RUN") -> (w795:T4)
                        n482 = local write "LAB03-2 (DISP)"(w795) -> ()
                      }
                      frame #4 {
                        n483 = local read "LAB03-2 (SIG)"() -> (w799:T2)
                        n484 = local read "LAB03-2 (TEMP START)"() -> (w801:cluster{"TL":dbl, "TN":dbl})
                        n485 = Unbundle(w799) -> ("Tmp Live"=w798:dbl, "Tmp Neut"=w797:dbl)  [unwired: 3 out]
                        n486 = Bundle(cluster=w801, "TL"=w798, "TN"=w797) -> (w800:cluster{"TL":dbl, "TN":dbl})
                        n487 = local write "LAB03-2 (TEMP START)"(w800) -> ()
                      }
                    }
                  }
                }
              }
              event "LAB04-1 RUN": Value Change {
                n488 = event-data() -> ("NewVal"=w803:bool)  [unwired: 1 in, 5 out]
                n489 = case shown="True" w803 {
                  tunnel: w807 -> [_ w832]
                  tunnel: w806 -> [_ w831]
                  tunnel: w804 -> [w808 w830]
                  tunnel: w805 -> [_ w829]
                  tunnel: w802 -> [_ w828]
                  frame False {
                    # "stop test"
                    n490 = stacked-sequence {
                      tunnel: w808 -> [w814 _]
                      frame #0 {
                        n491 = local read "LAB04-1 (DISP)"() -> (w813:T4)
                        n492 = Unbundle(w813) -> ("CYCLE"=w811:dbl, "MINS"=w812:dbl)  [unwired: 1 out]
                        n493 = case shown="\"CYCLE TEST\"" w814 {
                          tunnel: w812 -> [_ _ w821]
                          tunnel: w811 -> [w819 w820 _]
                          tunnel: [w819 w820 w821] -> w810
                          frame "CHART TEST", Default {
                          }
                          frame "CYCLE TEST" {
                          }
                          frame "T-RISE TEST" {
                          }
                        }
                        n494 = local read "LAB04-1 (TDMS)"() -> (w818:refnum<k34>)
                        n495 = Build Array("STOPPED") -> (w815:string[])
                        n496 = Build Array(w810) -> (w809:dbl[])
                        n497 = TDMS Write(0:w818, 5:"TEST RESULT", 7:w815, 9:w809) -> ()  [unwired: 2 in, 4 out]
                      }
                      frame #1 {
                        n498 = local read "LAB04-1 (DISP)"() -> (w827:T4)
                        n499 = Bundle(cluster=w827, "STATUS"="STOP") -> (w825:T4)  [unwired: 2 in]
                        n500 = call "Save data file to network drive v1.vi"("panel id"="LAB04-1") -> ("network file save error"=w822:errorcluster)  [unwired: 9 in, 1 out]
                        n501 = local write "LAB04-1 (RESULT)"(FALSE) -> ()
                        n502 = local write "LAB04-1 (DISP)"(w825) -> ()
                        n503 = local write "data file error"(w822) -> ()
                      }
                    }
                  }
                  frame True {
                    # "start new test and create test file"
                    n504 = stacked-sequence {
                      seq-local: [w833 _ _ _ _] -> [_ w858 _ _ _]
                      tunnel: w832 -> [w838 _ _ _ _]
                      tunnel: w831 -> [w834 _ _ _ _]
                      tunnel: w830 -> [w848 _ _ _ _]
                      tunnel: w829 -> [w841 _ _ _ _]
                      tunnel: w828 -> [w836 _ _ _ _]
                      frame #0 {
                        w835 = "\\"
                        n505 = local read "LAB04-1 (SET)"() -> (w843:T5)
                        n506 = case shown="\"CHART TEST\", Default" w848 {
                          tunnel: ["CHART TEST-" "CYCLE TEST-" "T-RISE TEST-"] -> w844
                          frame "CHART TEST", Default {
                          }
                          frame "CYCLE TEST" {
                          }
                          frame "T-RISE TEST" {
                          }
                        }
                        n507 = Unbundle(w843) -> ("DESCRIPTION"=w842:string)  [unwired: 4 out]
                        n508 = Concatenate Strings(w838, "LAB04-1\\", w836, w835, w834, w835) -> (w845:string)
                        n509 = String To Path(string=w845) -> (path=w847:path)
                        n510 = Concatenate Strings(w845, w844, w842, "-", w841, ".tdms") -> (w833:string)
                        n511 = Create Folder(path (use dialog)=w847) -> (error out=w846:errorcluster)  [unwired: 2 in, 2 out]
                        n512 = global write "Global 1.vi" "LAB04-1 FILE"(w833) -> ()
                        n513 = call <vilib>:"Clear Errors.vi"("error in (no error)"=w846) -> ()  [unwired: 6 in, 1 out]
                      }
                      frame #1 {
                        n514 = String To Path(string=w858) -> (path=w852:path)
                        n515 = TDMS Open(5:FALSE, 6:FALSE, 10:T14."create or replace" ("operation (0:open)"), 11:w852) -> (0:w854:errorcluster, 3:→"LAB04-1 (TDMS)":refnum<k34>)  [unwired: 3 in]
                        n516 = local write "data file error"(w854) -> ()
                      }
                      frame #2 {
                        n517 = local read "LAB04-1 (SET)"() -> (w864:T5)
                        n518 = local read "LAB04-1 (TDMS)"() -> (w875:refnum<k34>)
                        n519 = Build Array("Testers Name", "Description", "Set Test Cycles", "T-Rise minutes", "T-Rise Deg C") -> (w865:string[])
                        n520 = Unbundle(w864) -> ("NAME"=w863:string, "DESCRIPTION"=w862:string, "CYCLES"=w861:dbl, "T-RISE mins"=w860:dbl, "T-RISE deg C"=w859:dbl)
                        n521 = Number To Decimal String(number=w861) -> (decimal integer string=w874:string)  [unwired: 1 in]
                        n522 = Number To Decimal String(number=w860) -> (decimal integer string=w873:string)  [unwired: 1 in]
                        n523 = Number To Decimal String(number=w859) -> (decimal integer string=w872:string)  [unwired: 1 in]
                        n524 = Build Array(w863, w862, w874, w873, w872) -> (w871:string[])
                        n525 = TDMS Set Properties(5:w871, 7:w865, 11:w875) -> ()  [unwired: 3 in, 4 out]
                      }
                      frame #3 {
                        w877 = 0.0
                        n526 = local read "LAB04-1 (DISP)"() -> (w879:T4)
                        n527 = Bundle(cluster=w879, "CYCLE"=w877, "MINS"=w877, "STATUS"="RUN") -> (w878:T4)
                        n528 = local write "LAB04-1 (DISP)"(w878) -> ()
                      }
                      frame #4 {
                        n529 = local read "LAB04-1 (SIG)"() -> (w882:T2)
                        n530 = local read "LAB04-1 (TEMP START)"() -> (w884:cluster{"TL":dbl, "TN":dbl})
                        n531 = Unbundle(w882) -> ("Tmp Live"=w881:dbl, "Tmp Neut"=w880:dbl)  [unwired: 3 out]
                        n532 = Bundle(cluster=w884, "TL"=w881, "TN"=w880) -> (w883:cluster{"TL":dbl, "TN":dbl})
                        n533 = local write "LAB04-1 (TEMP START)"(w883) -> ()
                      }
                    }
                  }
                }
              }
              event "LAB04-2 RUN": Value Change {
                n534 = event-data() -> ("NewVal"=w886:bool)  [unwired: 1 in, 5 out]
                n535 = case shown="True" w886 {
                  tunnel: w890 -> [_ w915]
                  tunnel: w889 -> [_ w914]
                  tunnel: w887 -> [w891 w913]
                  tunnel: w888 -> [_ w912]
                  tunnel: w885 -> [_ w911]
                  frame False {
                    # "stop test"
                    n536 = stacked-sequence {
                      tunnel: w891 -> [w897 _]
                      frame #0 {
                        n537 = local read "LAB04-2 (DISP)"() -> (w896:T4)
                        n538 = Unbundle(w896) -> ("CYCLE"=w894:dbl, "MINS"=w895:dbl)  [unwired: 1 out]
                        n539 = case shown="\"CYCLE TEST\"" w897 {
                          tunnel: w895 -> [_ _ w904]
                          tunnel: w894 -> [w902 w903 _]
                          tunnel: [w902 w903 w904] -> w893
                          frame "CHART TEST", Default {
                          }
                          frame "CYCLE TEST" {
                          }
                          frame "T-RISE TEST" {
                          }
                        }
                        n540 = local read "LAB04-2 (TDMS)"() -> (w901:refnum<k34>)
                        n541 = Build Array("STOPPED") -> (w898:string[])
                        n542 = Build Array(w893) -> (w892:dbl[])
                        n543 = TDMS Write(0:w901, 5:"TEST RESULT", 7:w898, 9:w892) -> ()  [unwired: 2 in, 4 out]
                      }
                      frame #1 {
                        n544 = local read "LAB04-2 (DISP)"() -> (w910:T4)
                        n545 = Bundle(cluster=w910, "STATUS"="STOP") -> (w908:T4)  [unwired: 2 in]
                        n546 = call "Save data file to network drive v1.vi"("panel id"="LAB04-2") -> ("network file save error"=w905:errorcluster)  [unwired: 9 in, 1 out]
                        n547 = local write "LAB04-2 (RESULT)"(FALSE) -> ()
                        n548 = local write "LAB04-2 (DISP)"(w908) -> ()
                        n549 = local write "data file error"(w905) -> ()
                      }
                    }
                  }
                  frame True {
                    # "start new test and create test file"
                    n550 = stacked-sequence {
                      seq-local: [w916 _ _ _ _] -> [_ w941 _ _ _]
                      tunnel: w915 -> [w921 _ _ _ _]
                      tunnel: w914 -> [w917 _ _ _ _]
                      tunnel: w913 -> [w931 _ _ _ _]
                      tunnel: w912 -> [w924 _ _ _ _]
                      tunnel: w911 -> [w919 _ _ _ _]
                      frame #0 {
                        w918 = "\\"
                        n551 = local read "LAB04-2 (SET)"() -> (w926:T5)
                        n552 = case shown="\"CHART TEST\", Default" w931 {
                          tunnel: ["CHART TEST-" "CYCLE TEST-" "T-RISE TEST-"] -> w927
                          frame "CHART TEST", Default {
                          }
                          frame "CYCLE TEST" {
                          }
                          frame "T-RISE TEST" {
                          }
                        }
                        n553 = Unbundle(w926) -> ("DESCRIPTION"=w925:string)  [unwired: 4 out]
                        n554 = Concatenate Strings(w921, "LAB04-2\\", w919, w918, w917, w918) -> (w928:string)
                        n555 = String To Path(string=w928) -> (path=w930:path)
                        n556 = Concatenate Strings(w928, w927, w925, "-", w924, ".tdms") -> (w916:string)
                        n557 = Create Folder(path (use dialog)=w930) -> (error out=w929:errorcluster)  [unwired: 2 in, 2 out]
                        n558 = global write "Global 1.vi" "LAB04-2 FILE"(w916) -> ()
                        n559 = call <vilib>:"Clear Errors.vi"("error in (no error)"=w929) -> ()  [unwired: 6 in, 1 out]
                      }
                      frame #1 {
                        n560 = String To Path(string=w941) -> (path=w935:path)
                        n561 = TDMS Open(5:FALSE, 6:FALSE, 10:T14."create or replace" ("operation (0:open)"), 11:w935) -> (0:w937:errorcluster, 3:→"LAB04-2 (TDMS)":refnum<k34>)  [unwired: 3 in]
                        n562 = local write "data file error"(w937) -> ()
                      }
                      frame #2 {
                        n563 = local read "LAB04-2 (SET)"() -> (w947:T5)
                        n564 = local read "LAB04-2 (TDMS)"() -> (w958:refnum<k34>)
                        n565 = Build Array("Testers Name", "Description", "Set Test Cycles", "T-Rise minutes", "T-Rise Deg C") -> (w948:string[])
                        n566 = Unbundle(w947) -> ("NAME"=w946:string, "DESCRIPTION"=w945:string, "CYCLES"=w944:dbl, "T-RISE mins"=w943:dbl, "T-RISE deg C"=w942:dbl)
                        n567 = Number To Decimal String(number=w944) -> (decimal integer string=w957:string)  [unwired: 1 in]
                        n568 = Number To Decimal String(number=w943) -> (decimal integer string=w956:string)  [unwired: 1 in]
                        n569 = Number To Decimal String(number=w942) -> (decimal integer string=w955:string)  [unwired: 1 in]
                        n570 = Build Array(w946, w945, w957, w956, w955) -> (w954:string[])
                        n571 = TDMS Set Properties(5:w954, 7:w948, 11:w958) -> ()  [unwired: 3 in, 4 out]
                      }
                      frame #3 {
                        w960 = 0.0
                        n572 = local read "LAB04-2 (DISP)"() -> (w962:T4)
                        n573 = Bundle(cluster=w962, "CYCLE"=w960, "MINS"=w960, "STATUS"="RUN") -> (w961:T4)
                        n574 = local write "LAB04-2 (DISP)"(w961) -> ()
                      }
                      frame #4 {
                        n575 = local read "LAB04-2 (SIG)"() -> (w965:T2)
                        n576 = local read "LAB04-2 (TEMP START)"() -> (w967:cluster{"TL":dbl, "TN":dbl})
                        n577 = Unbundle(w965) -> ("Tmp Live"=w964:dbl, "Tmp Neut"=w963:dbl)  [unwired: 3 out]
                        n578 = Bundle(cluster=w967, "TL"=w964, "TN"=w963) -> (w966:cluster{"TL":dbl, "TN":dbl})
                        n579 = local write "LAB04-2 (TEMP START)"(w966) -> ()
                      }
                    }
                  }
                }
              }
              event "LAB05-1 RUN": Value Change {
                n580 = event-data() -> ("NewVal"=w969:bool)  [unwired: 1 in, 5 out]
                n581 = case shown="True" w969 {
                  tunnel: w973 -> [_ w998]
                  tunnel: w972 -> [_ w997]
                  tunnel: w970 -> [w974 w996]
                  tunnel: w971 -> [_ w995]
                  tunnel: w968 -> [_ w994]
                  frame False {
                    # "stop test"
                    n582 = stacked-sequence {
                      tunnel: w974 -> [w980 _]
                      frame #0 {
                        n583 = local read "LAB05-1 (DISP)"() -> (w979:T4)
                        n584 = Unbundle(w979) -> ("CYCLE"=w977:dbl, "MINS"=w978:dbl)  [unwired: 1 out]
                        n585 = case shown="\"CYCLE TEST\"" w980 {
                          tunnel: w978 -> [_ _ w987]
                          tunnel: w977 -> [w985 w986 _]
                          tunnel: [w985 w986 w987] -> w976
                          frame "CHART TEST", Default {
                          }
                          frame "CYCLE TEST" {
                          }
                          frame "T-RISE TEST" {
                          }
                        }
                        n586 = local read "LAB05-1 (TDMS)"() -> (w984:refnum<k34>)
                        n587 = Build Array("STOPPED") -> (w981:string[])
                        n588 = Build Array(w976) -> (w975:dbl[])
                        n589 = TDMS Write(0:w984, 5:"TEST RESULT", 7:w981, 9:w975) -> ()  [unwired: 2 in, 4 out]
                      }
                      frame #1 {
                        n590 = local read "LAB05-1 (DISP)"() -> (w993:T4)
                        n591 = Bundle(cluster=w993, "STATUS"="STOP") -> (w991:T4)  [unwired: 2 in]
                        n592 = call "Save data file to network drive v1.vi"("panel id"="LAB05-1") -> ("network file save error"=w988:errorcluster)  [unwired: 9 in, 1 out]
                        n593 = local write "LAB05-1 (RESULT)"(FALSE) -> ()
                        n594 = local write "LAB05-1 (DISP)"(w991) -> ()
                        n595 = local write "data file error"(w988) -> ()
                      }
                    }
                  }
                  frame True {
                    # "start new test and create test file"
                    n596 = stacked-sequence {
                      seq-local: [w999 _ _ _ _] -> [_ w1024 _ _ _]
                      tunnel: w998 -> [w1004 _ _ _ _]
                      tunnel: w997 -> [w1000 _ _ _ _]
                      tunnel: w996 -> [w1014 _ _ _ _]
                      tunnel: w995 -> [w1007 _ _ _ _]
                      tunnel: w994 -> [w1002 _ _ _ _]
                      frame #0 {
                        w1001 = "\\"
                        n597 = local read "LAB05-1 (SET)"() -> (w1009:T5)
                        n598 = case shown="\"CHART TEST\", Default" w1014 {
                          tunnel: ["CHART TEST-" "CYCLE TEST-" "T-RISE TEST-"] -> w1010
                          frame "CHART TEST", Default {
                          }
                          frame "CYCLE TEST" {
                          }
                          frame "T-RISE TEST" {
                          }
                        }
                        n599 = Unbundle(w1009) -> ("DESCRIPTION"=w1008:string)  [unwired: 4 out]
                        n600 = Concatenate Strings(w1004, "LAB05-1\\", w1002, w1001, w1000, w1001) -> (w1011:string)
                        n601 = String To Path(string=w1011) -> (path=w1013:path)
                        n602 = Concatenate Strings(w1011, w1010, w1008, "-", w1007, ".tdms") -> (w999:string)
                        n603 = Create Folder(path (use dialog)=w1013) -> (error out=w1012:errorcluster)  [unwired: 2 in, 2 out]
                        n604 = global write "Global 1.vi" "LAB05-1 FILE"(w999) -> ()
                        n605 = call <vilib>:"Clear Errors.vi"("error in (no error)"=w1012) -> ()  [unwired: 6 in, 1 out]
                      }
                      frame #1 {
                        n606 = String To Path(string=w1024) -> (path=w1018:path)
                        n607 = TDMS Open(5:FALSE, 6:FALSE, 10:T14."create or replace" ("operation (0:open)"), 11:w1018) -> (0:w1020:errorcluster, 3:→"LAB05-1 (TDMS)":refnum<k34>)  [unwired: 3 in]
                        n608 = local write "data file error"(w1020) -> ()
                      }
                      frame #2 {
                        n609 = local read "LAB05-1 (SET)"() -> (w1030:T5)
                        n610 = local read "LAB05-1 (TDMS)"() -> (w1041:refnum<k34>)
                        n611 = Build Array("Testers Name", "Description", "Set Test Cycles", "T-Rise minutes", "T-Rise Deg C") -> (w1031:string[])
                        n612 = Unbundle(w1030) -> ("NAME"=w1029:string, "DESCRIPTION"=w1028:string, "CYCLES"=w1027:dbl, "T-RISE mins"=w1026:dbl, "T-RISE deg C"=w1025:dbl)
                        n613 = Number To Decimal String(number=w1027) -> (decimal integer string=w1040:string)  [unwired: 1 in]
                        n614 = Number To Decimal String(number=w1026) -> (decimal integer string=w1039:string)  [unwired: 1 in]
                        n615 = Number To Decimal String(number=w1025) -> (decimal integer string=w1038:string)  [unwired: 1 in]
                        n616 = Build Array(w1029, w1028, w1040, w1039, w1038) -> (w1037:string[])
                        n617 = TDMS Set Properties(5:w1037, 7:w1031, 11:w1041) -> ()  [unwired: 3 in, 4 out]
                      }
                      frame #3 {
                        w1043 = 0.0
                        n618 = local read "LAB05-1 (DISP)"() -> (w1045:T4)
                        n619 = Bundle(cluster=w1045, "CYCLE"=w1043, "MINS"=w1043, "STATUS"="RUN") -> (w1044:T4)
                        n620 = local write "LAB05-1 (DISP)"(w1044) -> ()
                      }
                      frame #4 {
                        n621 = local read "LAB05-1 (SIG)"() -> (w1048:T2)
                        n622 = local read "LAB05-1 (TEMP START)"() -> (w1050:cluster{"TL":dbl, "TN":dbl})
                        n623 = Unbundle(w1048) -> ("Tmp Live"=w1047:dbl, "Tmp Neut"=w1046:dbl)  [unwired: 3 out]
                        n624 = Bundle(cluster=w1050, "TL"=w1047, "TN"=w1046) -> (w1049:cluster{"TL":dbl, "TN":dbl})
                        n625 = local write "LAB05-1 (TEMP START)"(w1049) -> ()
                      }
                    }
                  }
                }
              }
              event "LAB05-2 RUN": Value Change {
                n626 = event-data() -> ("NewVal"=w1052:bool)  [unwired: 1 in, 5 out]
                n627 = case shown="True" w1052 {
                  tunnel: w1056 -> [_ w1081]
                  tunnel: w1055 -> [_ w1080]
                  tunnel: w1053 -> [w1057 w1079]
                  tunnel: w1054 -> [_ w1078]
                  tunnel: w1051 -> [_ w1077]
                  frame False {
                    # "stop test"
                    n628 = stacked-sequence {
                      tunnel: w1057 -> [w1063 _]
                      frame #0 {
                        n629 = local read "LAB05-2 (DISP)"() -> (w1062:T4)
                        n630 = Unbundle(w1062) -> ("CYCLE"=w1060:dbl, "MINS"=w1061:dbl)  [unwired: 1 out]
                        n631 = case shown="\"CYCLE TEST\"" w1063 {
                          tunnel: w1061 -> [_ _ w1070]
                          tunnel: w1060 -> [w1068 w1069 _]
                          tunnel: [w1068 w1069 w1070] -> w1059
                          frame "CHART TEST", Default {
                          }
                          frame "CYCLE TEST" {
                          }
                          frame "T-RISE TEST" {
                          }
                        }
                        n632 = local read "LAB05-2 (TDMS)"() -> (w1067:refnum<k34>)
                        n633 = Build Array("STOPPED") -> (w1064:string[])
                        n634 = Build Array(w1059) -> (w1058:dbl[])
                        n635 = TDMS Write(0:w1067, 5:"TEST RESULT", 7:w1064, 9:w1058) -> ()  [unwired: 2 in, 4 out]
                      }
                      frame #1 {
                        n636 = local read "LAB05-2 (DISP)"() -> (w1076:T4)
                        n637 = Bundle(cluster=w1076, "STATUS"="STOP") -> (w1074:T4)  [unwired: 2 in]
                        n638 = local write "LAB05-2 (RESULT)"(FALSE) -> ()
                        n639 = local write "LAB05-2 (DISP)"(w1074) -> ()
                        n640 = call "Save data file to network drive v1.vi"("panel id"="LAB05-2") -> ("network file save error"=w1071:errorcluster)  [unwired: 9 in, 1 out]
                        n641 = local write "data file error"(w1071) -> ()
                      }
                    }
                  }
                  frame True {
                    # "start new test and create test file"
                    n642 = stacked-sequence {
                      seq-local: [w1082 _ _ _ _] -> [_ w1107 _ _ _]
                      tunnel: w1081 -> [w1087 _ _ _ _]
                      tunnel: w1080 -> [w1083 _ _ _ _]
                      tunnel: w1079 -> [w1097 _ _ _ _]
                      tunnel: w1078 -> [w1090 _ _ _ _]
                      tunnel: w1077 -> [w1085 _ _ _ _]
                      frame #0 {
                        w1084 = "\\"
                        n643 = local read "LAB05-2 (SET)"() -> (w1092:T5)
                        n644 = case shown="\"CHART TEST\", Default" w1097 {
                          tunnel: ["CHART TEST-" "CYCLE TEST-" "T-RISE TEST-"] -> w1093
                          frame "CHART TEST", Default {
                          }
                          frame "CYCLE TEST" {
                          }
                          frame "T-RISE TEST" {
                          }
                        }
                        n645 = Unbundle(w1092) -> ("DESCRIPTION"=w1091:string)  [unwired: 4 out]
                        n646 = Concatenate Strings(w1087, "LAB05-2\\", w1085, w1084, w1083, w1084) -> (w1094:string)
                        n647 = String To Path(string=w1094) -> (path=w1096:path)
                        n648 = Concatenate Strings(w1094, w1093, w1091, "-", w1090, ".tdms") -> (w1082:string)
                        n649 = Create Folder(path (use dialog)=w1096) -> (error out=w1095:errorcluster)  [unwired: 2 in, 2 out]
                        n650 = global write "Global 1.vi" "LAB05-2 FILE"(w1082) -> ()
                        n651 = call <vilib>:"Clear Errors.vi"("error in (no error)"=w1095) -> ()  [unwired: 6 in, 1 out]
                      }
                      frame #1 {
                        n652 = String To Path(string=w1107) -> (path=w1101:path)
                        n653 = TDMS Open(5:FALSE, 6:FALSE, 10:T14."create or replace" ("operation (0:open)"), 11:w1101) -> (0:w1103:errorcluster, 3:→"LAB05-2 (TDMS)":refnum<k34>)  [unwired: 3 in]
                        n654 = local write "data file error"(w1103) -> ()
                      }
                      frame #2 {
                        n655 = local read "LAB05-2 (SET)"() -> (w1113:T5)
                        n656 = local read "LAB05-2 (TDMS)"() -> (w1124:refnum<k34>)
                        n657 = Build Array("Testers Name", "Description", "Set Test Cycles", "T-Rise minutes", "T-Rise Deg C") -> (w1114:string[])
                        n658 = Unbundle(w1113) -> ("NAME"=w1112:string, "DESCRIPTION"=w1111:string, "CYCLES"=w1110:dbl, "T-RISE mins"=w1109:dbl, "T-RISE deg C"=w1108:dbl)
                        n659 = Number To Decimal String(number=w1110) -> (decimal integer string=w1123:string)  [unwired: 1 in]
                        n660 = Number To Decimal String(number=w1109) -> (decimal integer string=w1122:string)  [unwired: 1 in]
                        n661 = Number To Decimal String(number=w1108) -> (decimal integer string=w1121:string)  [unwired: 1 in]
                        n662 = Build Array(w1112, w1111, w1123, w1122, w1121) -> (w1120:string[])
                        n663 = TDMS Set Properties(5:w1120, 7:w1114, 11:w1124) -> ()  [unwired: 3 in, 4 out]
                      }
                      frame #3 {
                        w1126 = 0.0
                        n664 = local read "LAB05-2 (DISP)"() -> (w1128:T4)
                        n665 = Bundle(cluster=w1128, "CYCLE"=w1126, "MINS"=w1126, "STATUS"="RUN") -> (w1127:T4)
                        n666 = local write "LAB05-2 (DISP)"(w1127) -> ()
                      }
                      frame #4 {
                        n667 = local read "LAB05-2 (SIG)"() -> (w1131:T2)
                        n668 = local read "LAB05-2 (TEMP START)"() -> (w1133:cluster{"TL":dbl, "TN":dbl})
                        n669 = Unbundle(w1131) -> ("Tmp Live"=w1130:dbl, "Tmp Neut"=w1129:dbl)  [unwired: 3 out]
                        n670 = Bundle(cluster=w1133, "TL"=w1130, "TN"=w1129) -> (w1132:cluster{"TL":dbl, "TN":dbl})
                        n671 = local write "LAB05-2 (TEMP START)"(w1132) -> ()
                      }
                    }
                  }
                }
              }
            }
          }
          frame #4 {
            # "check if test cycles reached for cycle tests, if so then test pass"
            n672 = stacked-sequence {
              tunnel: w1153 -> [_ _ _ _ _ _ _ _ _ _]
              tunnel: w1152 -> [_ _ _ _ _ _ _ _ _ _]
              tunnel: w1151 -> [_ _ _ _ _ _ _ _ _ _]
              tunnel: w1150 -> [_ _ _ _ _ _ _ _ _ _]
              tunnel: w1149 -> [_ _ _ _ _ _ _ _ _ _]
              tunnel: w1148 -> [_ _ _ _ _ _ _ _ _ _]
              tunnel: w1147 -> [_ _ _ _ _ _ _ _ _ _]
              tunnel: w1146 -> [_ _ _ _ _ _ _ _ _ _]
              tunnel: w1145 -> [_ _ _ _ _ _ _ _ _ _]
              tunnel: w1144 -> [_ _ _ _ _ _ _ _ _ _]
              tunnel: w1143 -> [w1158 _ _ _ _ _ _ _ _ _]
              tunnel: w1142 -> [_ w1193 _ _ _ _ _ _ _ _]
              tunnel: w1141 -> [_ _ w1232 _ _ _ _ _ _ _]
              tunnel: w1140 -> [_ _ _ w1271 _ _ _ _ _ _]
              tunnel: w1139 -> [_ _ _ _ w1310 _ _ _ _ _]
              tunnel: w1138 -> [_ _ _ _ _ w1349 _ _ _ _]
              tunnel: w1137 -> [_ _ _ _ _ _ w1388 _ _ _]
              tunnel: w1136 -> [_ _ _ _ _ _ _ w1427 _ _]
              tunnel: w1135 -> [_ _ _ _ _ _ _ _ w1466 _]
              tunnel: w1134 -> [_ _ _ _ _ _ _ _ _ w1505]
              frame #0 {
                # "LAB01-1"
                n673 = Less?(x=w1158, y=2) -> (x < y?=w1156:bool)
                n674 = local read "LAB01-1 (DISP)"() -> (w1159:T4)
                n675 = Unbundle(w1159) -> ("STATUS"=w1160:string)  [unwired: 2 out]
                n676 = Equal?(x=w1160, y="RUN") -> (x = y?=w1155:bool)
                n677 = And(x=w1155, y=w1156) -> (x .and. y?=w1154:bool)
                n678 = case shown="True" w1154 {
                  tunnel: w1159 -> [_ w1163]
                  tunnel: w1158 -> [_ w1168]
                  frame False {
                  }
                  frame True {
                    n679 = local read "LAB01-1 (SET)"() -> (w1170:T5)
                    n680 = local read "LAB01-1 (TDMS)"() -> (w1162:refnum<k34>)
                    n681 = Unbundle(w1163) -> ("CYCLE"=w1169:dbl)  [unwired: 2 out]
                    n682 = Unbundle(w1170) -> ("CYCLES"=w1165:dbl, "T-RISE mins"=w1167:dbl)  [unwired: 3 out]
                    n683 = case shown="\"CHART TEST\", Default" w1168 {
                      tunnel: w1167 -> [_ _ w1177]
                      tunnel: [w1172 w1174 w1177] -> w1166
                      tunnel: w1165 -> [w1172 w1174 _]
                      tunnel: ["CHART TEST" "CYCLES" "T-RISE TEST"] -> w1164
                      frame "CHART TEST", Default {
                      }
                      frame "CYCLE TEST" {
                      }
                      frame "T-RISE TEST" {
                      }
                    }
                    n684 = Greater Or Equal?(x=w1169, y=w1165) -> (x >= y?=w1171:bool)
                    n685 = case shown="True" w1171 {
                      tunnel: w1166 -> [w1181 _]
                      tunnel: w1164 -> [w1180 _]
                      tunnel: w1163 -> [w1179 _]
                      tunnel: w1162 -> [w1178 _]
                      frame True {
                        n686 = stacked-sequence {
                          tunnel: w1181 -> [w1185 _]
                          tunnel: w1180 -> [w1183 _]
                          tunnel: w1179 -> [_ w1191]
                          tunnel: w1178 -> [w1182 _]
                          frame #0 {
                            n687 = Build Array(w1183) -> (w1186:string[])
                            n688 = Build Array(w1185) -> (w1184:dbl[])
                            n689 = TDMS Write(0:w1182, 5:"TEST PASS", 7:w1186, 9:w1184) -> (15:w1188:errorcluster)  [unwired: 2 in, 3 out]
                            n690 = local write "data file error"(w1188) -> ()
                          }
                          frame #1 {
                            n691 = Bundle(cluster=w1191, "STATUS"="CYCLE PASS") -> (w1189:T4)  [unwired: 2 in]
                            n692 = local write "LAB01-1 (RESULT)"(TRUE) -> ()
                            n693 = local write "LAB01-1 (DISP)"(w1189) -> ()
                          }
                        }
                      }
                      frame False {
                      }
                    }
                  }
                }
              }
              frame #1 {
                # "LAB01-2"
                n694 = Less?(x=w1193, y=2) -> (x < y?=w1196:bool)
                n695 = local read "LAB01-2 (DISP)"() -> (w1198:T4)
                n696 = Unbundle(w1198) -> ("STATUS"=w1199:string)  [unwired: 2 out]
                n697 = Equal?(x=w1199, y="RUN") -> (x = y?=w1195:bool)
                n698 = And(x=w1195, y=w1196) -> (x .and. y?=w1194:bool)
                n699 = case shown="True" w1194 {
                  tunnel: w1198 -> [_ w1202]
                  tunnel: w1193 -> [_ w1207]
                  frame False {
                  }
                  frame True {
                    n700 = local read "LAB01-2 (SET)"() -> (w1209:T5)
                    n701 = local read "LAB01-2 (TDMS)"() -> (w1201:refnum<k34>)
                    n702 = Unbundle(w1202) -> ("CYCLE"=w1208:dbl)  [unwired: 2 out]
                    n703 = Unbundle(w1209) -> ("CYCLES"=w1204:dbl, "T-RISE mins"=w1206:dbl)  [unwired: 3 out]
                    n704 = case shown="\"CHART TEST\", Default" w1207 {
                      tunnel: w1206 -> [_ _ w1216]
                      tunnel: [w1211 w1213 w1216] -> w1205
                      tunnel: w1204 -> [w1211 w1213 _]
                      tunnel: ["CHART TEST " "CYCLES" "T-RISE TEST"] -> w1203
                      frame "CHART TEST", Default {
                      }
                      frame "CYCLE TEST" {
                      }
                      frame "T-RISE TEST" {
                      }
                    }
                    n705 = Greater Or Equal?(x=w1208, y=w1204) -> (x >= y?=w1210:bool)
                    n706 = case shown="True" w1210 {
                      tunnel: w1205 -> [w1220 _]
                      tunnel: w1203 -> [w1219 _]
                      tunnel: w1202 -> [w1218 _]
                      tunnel: w1201 -> [w1217 _]
                      frame True {
                        n707 = stacked-sequence {
                          tunnel: w1220 -> [w1224 _]
                          tunnel: w1219 -> [w1222 _]
                          tunnel: w1218 -> [_ w1230]
                          tunnel: w1217 -> [w1221 _]
                          frame #0 {
                            n708 = Build Array(w1222) -> (w1225:string[])
                            n709 = Build Array(w1224) -> (w1223:dbl[])
                            n710 = TDMS Write(0:w1221, 5:"TEST PASS", 7:w1225, 9:w1223) -> (15:w1227:errorcluster)  [unwired: 2 in, 3 out]
                            n711 = local write "data file error"(w1227) -> ()
                          }
                          frame #1 {
                            n712 = Bundle(cluster=w1230, "STATUS"="CYCLE PASS") -> (w1228:T4)  [unwired: 2 in]
                            n713 = local write "LAB01-2 (RESULT)"(TRUE) -> ()
                            n714 = local write "LAB01-2 (DISP)"(w1228) -> ()
                          }
                        }
                      }
                      frame False {
                      }
                    }
                  }
                }
              }
              frame #2 {
                # "LAB02-1"
                n715 = Less?(x=w1232, y=2) -> (x < y?=w1235:bool)
                n716 = local read "LAB02-1 (DISP)"() -> (w1237:T4)
                n717 = Unbundle(w1237) -> ("STATUS"=w1238:string)  [unwired: 2 out]
                n718 = Equal?(x=w1238, y="RUN") -> (x = y?=w1234:bool)
                n719 = And(x=w1234, y=w1235) -> (x .and. y?=w1233:bool)
                n720 = case shown="True" w1233 {
                  tunnel: w1237 -> [_ w1241]
                  tunnel: w1232 -> [_ w1246]
                  frame False {
                  }
                  frame True {
                    n721 = local read "LAB02-1 (SET)"() -> (w1248:T5)
                    n722 = local read "LAB02-1 (TDMS)"() -> (w1240:refnum<k34>)
                    n723 = Unbundle(w1241) -> ("CYCLE"=w1247:dbl)  [unwired: 2 out]
                    n724 = Unbundle(w1248) -> ("CYCLES"=w1243:dbl, "T-RISE mins"=w1245:dbl)  [unwired: 3 out]
                    n725 = case shown="\"CHART TEST\", Default" w1246 {
                      tunnel: w1245 -> [_ _ w1255]
                      tunnel: [w1250 w1252 w1255] -> w1244
                      tunnel: w1243 -> [w1250 w1252 _]
                      tunnel: ["CHART TEST" "CYCLES" "T-RISE TEST"] -> w1242
                      frame "CHART TEST", Default {
                      }
                      frame "CYCLE TEST" {
                      }
                      frame "T-RISE TEST" {
                      }
                    }
                    n726 = Greater Or Equal?(x=w1247, y=w1243) -> (x >= y?=w1249:bool)
                    n727 = case shown="True" w1249 {
                      tunnel: w1244 -> [w1259 _]
                      tunnel: w1242 -> [w1258 _]
                      tunnel: w1241 -> [w1257 _]
                      tunnel: w1240 -> [w1256 _]
                      frame True {
                        n728 = stacked-sequence {
                          tunnel: w1259 -> [w1263 _]
                          tunnel: w1258 -> [w1261 _]
                          tunnel: w1257 -> [_ w1269]
                          tunnel: w1256 -> [w1260 _]
                          frame #0 {
                            n729 = Build Array(w1261) -> (w1264:string[])
                            n730 = Build Array(w1263) -> (w1262:dbl[])
                            n731 = TDMS Write(0:w1260, 5:"TEST PASS", 7:w1264, 9:w1262) -> (15:w1266:errorcluster)  [unwired: 2 in, 3 out]
                            n732 = local write "data file error"(w1266) -> ()
                          }
                          frame #1 {
                            n733 = Bundle(cluster=w1269, "STATUS"="CYCLE PASS") -> (w1267:T4)  [unwired: 2 in]
                            n734 = local write "LAB02-1 (RESULT)"(TRUE) -> ()
                            n735 = local write "LAB02-1 (DISP)"(w1267) -> ()
                          }
                        }
                      }
                      frame False {
                      }
                    }
                  }
                }
              }
              frame #3 {
                # "LAB02-2"
                n736 = Less?(x=w1271, y=2) -> (x < y?=w1274:bool)
                n737 = local read "LAB02-2 (DISP)"() -> (w1276:T4)
                n738 = Unbundle(w1276) -> ("STATUS"=w1277:string)  [unwired: 2 out]
                n739 = Equal?(x=w1277, y="RUN") -> (x = y?=w1273:bool)
                n740 = And(x=w1273, y=w1274) -> (x .and. y?=w1272:bool)
                n741 = case shown="True" w1272 {
                  tunnel: w1276 -> [_ w1280]
                  tunnel: w1271 -> [_ w1285]
                  frame False {
                  }
                  frame True {
                    n742 = local read "LAB02-2 (SET)"() -> (w1287:T5)
                    n743 = local read "LAB02-2 (TDMS)"() -> (w1279:refnum<k34>)
                    n744 = Unbundle(w1280) -> ("CYCLE"=w1286:dbl)  [unwired: 2 out]
                    n745 = Unbundle(w1287) -> ("CYCLES"=w1282:dbl, "T-RISE mins"=w1284:dbl)  [unwired: 3 out]
                    n746 = case shown="\"CHART TEST\", Default" w1285 {
                      tunnel: w1284 -> [_ _ w1294]
                      tunnel: [w1289 w1291 w1294] -> w1283
                      tunnel: w1282 -> [w1289 w1291 _]
                      tunnel: ["CHART TEST" "CYCLES" "T-RISE TEST"] -> w1281
                      frame "CHART TEST", Default {
                      }
                      frame "CYCLE TEST" {
                      }
                      frame "T-RISE TEST" {
                      }
                    }
                    n747 = Greater Or Equal?(x=w1286, y=w1282) -> (x >= y?=w1288:bool)
                    n748 = case shown="True" w1288 {
                      tunnel: w1283 -> [w1298 _]
                      tunnel: w1281 -> [w1297 _]
                      tunnel: w1280 -> [w1296 _]
                      tunnel: w1279 -> [w1295 _]
                      frame True {
                        n749 = stacked-sequence {
                          tunnel: w1298 -> [w1302 _]
                          tunnel: w1297 -> [w1300 _]
                          tunnel: w1296 -> [_ w1308]
                          tunnel: w1295 -> [w1299 _]
                          frame #0 {
                            n750 = Build Array(w1300) -> (w1303:string[])
                            n751 = Build Array(w1302) -> (w1301:dbl[])
                            n752 = TDMS Write(0:w1299, 5:"TEST PASS", 7:w1303, 9:w1301) -> (15:w1305:errorcluster)  [unwired: 2 in, 3 out]
                            n753 = local write "data file error"(w1305) -> ()
                          }
                          frame #1 {
                            n754 = Bundle(cluster=w1308, "STATUS"="CYCLE PASS") -> (w1306:T4)  [unwired: 2 in]
                            n755 = local write "LAB02-2 (RESULT)"(TRUE) -> ()
                            n756 = local write "LAB02-2 (DISP)"(w1306) -> ()
                          }
                        }
                      }
                      frame False {
                      }
                    }
                  }
                }
              }
              frame #4 {
                # "LAB03-1"
                n757 = Less?(x=w1310, y=2) -> (x < y?=w1313:bool)
                n758 = local read "LAB03-1 (DISP)"() -> (w1315:T4)
                n759 = Unbundle(w1315) -> ("STATUS"=w1316:string)  [unwired: 2 out]
                n760 = Equal?(x=w1316, y="RUN") -> (x = y?=w1312:bool)
                n761 = And(x=w1312, y=w1313) -> (x .and. y?=w1311:bool)
                n762 = case shown="True" w1311 {
                  tunnel: w1315 -> [_ w1319]
                  tunnel: w1310 -> [_ w1324]
                  frame False {
                  }
                  frame True {
                    n763 = local read "LAB03-1 (SET)"() -> (w1326:T5)
                    n764 = local read "LAB03-1 (TDMS)"() -> (w1318:refnum<k34>)
                    n765 = Unbundle(w1319) -> ("CYCLE"=w1325:dbl)  [unwired: 2 out]
                    n766 = Unbundle(w1326) -> ("CYCLES"=w1321:dbl, "T-RISE mins"=w1323:dbl)  [unwired: 3 out]
                    n767 = case shown="\"CHART TEST\", Default" w1324 {
                      tunnel: w1323 -> [_ _ w1333]
                      tunnel: [w1328 w1330 w1333] -> w1322
                      tunnel: w1321 -> [w1328 w1330 _]
                      tunnel: ["CHART TEST" "CYCLES" "T-RISE TEST"] -> w1320
                      frame "CHART TEST", Default {
                      }
                      frame "CYCLE TEST" {
                      }
                      frame "T-RISE TEST" {
                      }
                    }
                    n768 = Greater Or Equal?(x=w1325, y=w1321) -> (x >= y?=w1327:bool)
                    n769 = case shown="True" w1327 {
                      tunnel: w1322 -> [w1337 _]
                      tunnel: w1320 -> [w1336 _]
                      tunnel: w1319 -> [w1335 _]
                      tunnel: w1318 -> [w1334 _]
                      frame True {
                        n770 = stacked-sequence {
                          tunnel: w1337 -> [w1341 _]
                          tunnel: w1336 -> [w1339 _]
                          tunnel: w1335 -> [_ w1347]
                          tunnel: w1334 -> [w1338 _]
                          frame #0 {
                            n771 = Build Array(w1339) -> (w1342:string[])
                            n772 = Build Array(w1341) -> (w1340:dbl[])
                            n773 = TDMS Write(0:w1338, 5:"TEST PASS", 7:w1342, 9:w1340) -> (15:w1344:errorcluster)  [unwired: 2 in, 3 out]
                            n774 = local write "data file error"(w1344) -> ()
                          }
                          frame #1 {
                            n775 = Bundle(cluster=w1347, "STATUS"="CYCLE PASS") -> (w1345:T4)  [unwired: 2 in]
                            n776 = local write "LAB03-1 (RESULT)"(TRUE) -> ()
                            n777 = local write "LAB03-1 (DISP)"(w1345) -> ()
                          }
                        }
                      }
                      frame False {
                      }
                    }
                  }
                }
              }
              frame #5 {
                # "LAB03-2"
                n778 = Less?(x=w1349, y=2) -> (x < y?=w1352:bool)
                n779 = local read "LAB03-2 (DISP)"() -> (w1354:T4)
                n780 = Unbundle(w1354) -> ("STATUS"=w1355:string)  [unwired: 2 out]
                n781 = Equal?(x=w1355, y="RUN") -> (x = y?=w1351:bool)
                n782 = And(x=w1351, y=w1352) -> (x .and. y?=w1350:bool)
                n783 = case shown="True" w1350 {
                  tunnel: w1354 -> [_ w1358]
                  tunnel: w1349 -> [_ w1363]
                  frame False {
                  }
                  frame True {
                    n784 = local read "LAB03-2 (SET)"() -> (w1365:T5)
                    n785 = local read "LAB03-2 (TDMS)"() -> (w1357:refnum<k34>)
                    n786 = Unbundle(w1358) -> ("CYCLE"=w1364:dbl)  [unwired: 2 out]
                    n787 = Unbundle(w1365) -> ("CYCLES"=w1360:dbl, "T-RISE mins"=w1362:dbl)  [unwired: 3 out]
                    n788 = case shown="\"CHART TEST\", Default" w1363 {
                      tunnel: w1362 -> [_ _ w1372]
                      tunnel: [w1367 w1369 w1372] -> w1361
                      tunnel: w1360 -> [w1367 w1369 _]
                      tunnel: ["CHART TEST" "CYCLES" "T-RISE TEST"] -> w1359
                      frame "CHART TEST", Default {
                      }
                      frame "CYCLE TEST" {
                      }
                      frame "T-RISE TEST" {
                      }
                    }
                    n789 = Greater Or Equal?(x=w1364, y=w1360) -> (x >= y?=w1366:bool)
                    n790 = case shown="True" w1366 {
                      tunnel: w1361 -> [w1376 _]
                      tunnel: w1359 -> [w1375 _]
                      tunnel: w1358 -> [w1374 _]
                      tunnel: w1357 -> [w1373 _]
                      frame True {
                        n791 = stacked-sequence {
                          tunnel: w1376 -> [w1380 _]
                          tunnel: w1375 -> [w1378 _]
                          tunnel: w1374 -> [_ w1386]
                          tunnel: w1373 -> [w1377 _]
                          frame #0 {
                            n792 = Build Array(w1378) -> (w1381:string[])
                            n793 = Build Array(w1380) -> (w1379:dbl[])
                            n794 = TDMS Write(0:w1377, 5:"TEST PASS", 7:w1381, 9:w1379) -> (15:w1383:errorcluster)  [unwired: 2 in, 3 out]
                            n795 = local write "data file error"(w1383) -> ()
                          }
                          frame #1 {
                            n796 = Bundle(cluster=w1386, "STATUS"="CYCLE PASS") -> (w1384:T4)  [unwired: 2 in]
                            n797 = local write "LAB03-2 (RESULT)"(TRUE) -> ()
                            n798 = local write "LAB03-2 (DISP)"(w1384) -> ()
                          }
                        }
                      }
                      frame False {
                      }
                    }
                  }
                }
              }
              frame #6 {
                # "LAB04-1"
                n799 = Less?(x=w1388, y=2) -> (x < y?=w1391:bool)
                n800 = local read "LAB04-1 (DISP)"() -> (w1393:T4)
                n801 = Unbundle(w1393) -> ("STATUS"=w1394:string)  [unwired: 2 out]
                n802 = Equal?(x=w1394, y="RUN") -> (x = y?=w1390:bool)
                n803 = And(x=w1390, y=w1391) -> (x .and. y?=w1389:bool)
                n804 = case shown="True" w1389 {
                  tunnel: w1393 -> [_ w1397]
                  tunnel: w1388 -> [_ w1402]
                  frame False {
                  }
                  frame True {
                    n805 = local read "LAB04-1 (SET)"() -> (w1404:T5)
                    n806 = local read "LAB04-1 (TDMS)"() -> (w1396:refnum<k34>)
                    n807 = Unbundle(w1397) -> ("CYCLE"=w1403:dbl)  [unwired: 2 out]
                    n808 = Unbundle(w1404) -> ("CYCLES"=w1399:dbl, "T-RISE mins"=w1401:dbl)  [unwired: 3 out]
                    n809 = case shown="\"CHART TEST\", Default" w1402 {
                      tunnel: w1401 -> [_ _ w1411]
                      tunnel: [w1406 w1408 w1411] -> w1400
                      tunnel: w1399 -> [w1406 w1408 _]
                      tunnel: ["CHART TEST" "CYCLES" "T-RISE TEST"] -> w1398
                      frame "CHART TEST", Default {
                      }
                      frame "CYCLE TEST" {
                      }
                      frame "T-RISE TEST" {
                      }
                    }
                    n810 = Greater Or Equal?(x=w1403, y=w1399) -> (x >= y?=w1405:bool)
                    n811 = case shown="True" w1405 {
                      tunnel: w1400 -> [w1415 _]
                      tunnel: w1398 -> [w1414 _]
                      tunnel: w1397 -> [w1413 _]
                      tunnel: w1396 -> [w1412 _]
                      frame True {
                        n812 = stacked-sequence {
                          tunnel: w1415 -> [w1419 _]
                          tunnel: w1414 -> [w1417 _]
                          tunnel: w1413 -> [_ w1425]
                          tunnel: w1412 -> [w1416 _]
                          frame #0 {
                            n813 = Build Array(w1417) -> (w1420:string[])
                            n814 = Build Array(w1419) -> (w1418:dbl[])
                            n815 = TDMS Write(0:w1416, 5:"TEST PASS", 7:w1420, 9:w1418) -> (15:w1422:errorcluster)  [unwired: 2 in, 3 out]
                            n816 = local write "data file error"(w1422) -> ()
                          }
                          frame #1 {
                            n817 = Bundle(cluster=w1425, "STATUS"="CYCLE PASS") -> (w1423:T4)  [unwired: 2 in]
                            n818 = local write "LAB04-1 (RESULT)"(TRUE) -> ()
                            n819 = local write "LAB04-1 (DISP)"(w1423) -> ()
                          }
                        }
                      }
                      frame False {
                      }
                    }
                  }
                }
              }
              frame #7 {
                # "LAB04-2"
                n820 = Less?(x=w1427, y=2) -> (x < y?=w1430:bool)
                n821 = local read "LAB04-2 (DISP)"() -> (w1432:T4)
                n822 = Unbundle(w1432) -> ("STATUS"=w1433:string)  [unwired: 2 out]
                n823 = Equal?(x=w1433, y="RUN") -> (x = y?=w1429:bool)
                n824 = And(x=w1429, y=w1430) -> (x .and. y?=w1428:bool)
                n825 = case shown="True" w1428 {
                  tunnel: w1432 -> [_ w1436]
                  tunnel: w1427 -> [_ w1441]
                  frame False {
                  }
                  frame True {
                    n826 = local read "LAB04-2 (SET)"() -> (w1443:T5)
                    n827 = local read "LAB04-2 (TDMS)"() -> (w1435:refnum<k34>)
                    n828 = Unbundle(w1436) -> ("CYCLE"=w1442:dbl)  [unwired: 2 out]
                    n829 = Unbundle(w1443) -> ("CYCLES"=w1438:dbl, "T-RISE mins"=w1440:dbl)  [unwired: 3 out]
                    n830 = case shown="\"CHART TEST\", Default" w1441 {
                      tunnel: w1440 -> [_ _ w1450]
                      tunnel: [w1445 w1447 w1450] -> w1439
                      tunnel: w1438 -> [w1445 w1447 _]
                      tunnel: ["CHART TEST" "CYCLES" "T-RISE TEST"] -> w1437
                      frame "CHART TEST", Default {
                      }
                      frame "CYCLE TEST" {
                      }
                      frame "T-RISE TEST" {
                      }
                    }
                    n831 = Greater Or Equal?(x=w1442, y=w1438) -> (x >= y?=w1444:bool)
                    n832 = case shown="True" w1444 {
                      tunnel: w1439 -> [w1454 _]
                      tunnel: w1437 -> [w1453 _]
                      tunnel: w1436 -> [w1452 _]
                      tunnel: w1435 -> [w1451 _]
                      frame True {
                        n833 = stacked-sequence {
                          tunnel: w1454 -> [w1458 _]
                          tunnel: w1453 -> [w1456 _]
                          tunnel: w1452 -> [_ w1464]
                          tunnel: w1451 -> [w1455 _]
                          frame #0 {
                            n834 = Build Array(w1456) -> (w1459:string[])
                            n835 = Build Array(w1458) -> (w1457:dbl[])
                            n836 = TDMS Write(0:w1455, 5:"TEST PASS", 7:w1459, 9:w1457) -> (15:w1461:errorcluster)  [unwired: 2 in, 3 out]
                            n837 = local write "data file error"(w1461) -> ()
                          }
                          frame #1 {
                            n838 = Bundle(cluster=w1464, "STATUS"="CYCLE PASS") -> (w1462:T4)  [unwired: 2 in]
                            n839 = local write "LAB04-2 (RESULT)"(TRUE) -> ()
                            n840 = local write "LAB04-2 (DISP)"(w1462) -> ()
                          }
                        }
                      }
                      frame False {
                      }
                    }
                  }
                }
              }
              frame #8 {
                # "LAB05-1"
                n841 = Less?(x=w1466, y=2) -> (x < y?=w1469:bool)
                n842 = local read "LAB05-1 (DISP)"() -> (w1471:T4)
                n843 = Unbundle(w1471) -> ("STATUS"=w1472:string)  [unwired: 2 out]
                n844 = Equal?(x=w1472, y="RUN") -> (x = y?=w1468:bool)
                n845 = And(x=w1468, y=w1469) -> (x .and. y?=w1467:bool)
                n846 = case shown="True" w1467 {
                  tunnel: w1471 -> [_ w1475]
                  tunnel: w1466 -> [_ w1480]
                  frame False {
                  }
                  frame True {
                    n847 = local read "LAB05-1 (SET)"() -> (w1482:T5)
                    n848 = local read "LAB05-1 (TDMS)"() -> (w1474:refnum<k34>)
                    n849 = Unbundle(w1475) -> ("CYCLE"=w1481:dbl)  [unwired: 2 out]
                    n850 = Unbundle(w1482) -> ("CYCLES"=w1477:dbl, "T-RISE mins"=w1479:dbl)  [unwired: 3 out]
                    n851 = case shown="\"CHART TEST\", Default" w1480 {
                      tunnel: w1479 -> [_ _ w1489]
                      tunnel: [w1484 w1486 w1489] -> w1478
                      tunnel: w1477 -> [w1484 w1486 _]
                      tunnel: ["CHART TEST" "CYCLES" "T-RISE TEST"] -> w1476
                      frame "CHART TEST", Default {
                      }
                      frame "CYCLE TEST" {
                      }
                      frame "T-RISE TEST" {
                      }
                    }
                    n852 = Greater Or Equal?(x=w1481, y=w1477) -> (x >= y?=w1483:bool)
                    n853 = case shown="True" w1483 {
                      tunnel: w1478 -> [w1493 _]
                      tunnel: w1476 -> [w1492 _]
                      tunnel: w1475 -> [w1491 _]
                      tunnel: w1474 -> [w1490 _]
                      frame True {
                        n854 = stacked-sequence {
                          tunnel: w1493 -> [w1497 _]
                          tunnel: w1492 -> [w1495 _]
                          tunnel: w1491 -> [_ w1503]
                          tunnel: w1490 -> [w1494 _]
                          frame #0 {
                            n855 = Build Array(w1495) -> (w1498:string[])
                            n856 = Build Array(w1497) -> (w1496:dbl[])
                            n857 = TDMS Write(0:w1494, 5:"TEST PASS", 7:w1498, 9:w1496) -> (15:w1500:errorcluster)  [unwired: 2 in, 3 out]
                            n858 = local write "data file error"(w1500) -> ()
                          }
                          frame #1 {
                            n859 = Bundle(cluster=w1503, "STATUS"="CYCLE PASS") -> (w1501:T4)  [unwired: 2 in]
                            n860 = local write "LAB05-1 (RESULT)"(TRUE) -> ()
                            n861 = local write "LAB05-1 (DISP)"(w1501) -> ()
                          }
                        }
                      }
                      frame False {
                      }
                    }
                  }
                }
              }
              frame #9 {
                # "LAB05-2"
                n862 = Less?(x=w1505, y=2) -> (x < y?=w1508:bool)
                n863 = local read "LAB05-2 (DISP)"() -> (w1510:T4)
                n864 = Unbundle(w1510) -> ("STATUS"=w1511:string)  [unwired: 2 out]
                n865 = Equal?(x=w1511, y="RUN") -> (x = y?=w1507:bool)
                n866 = And(x=w1507, y=w1508) -> (x .and. y?=w1506:bool)
                n867 = case shown="True" w1506 {
                  tunnel: w1510 -> [_ w1514]
                  tunnel: w1505 -> [_ w1519]
                  frame False {
                  }
                  frame True {
                    n868 = local read "LAB05-2 (SET)"() -> (w1521:T5)
                    n869 = local read "LAB05-2 (TDMS)"() -> (w1513:refnum<k34>)
                    n870 = Unbundle(w1514) -> ("CYCLE"=w1520:dbl)  [unwired: 2 out]
                    n871 = Unbundle(w1521) -> ("CYCLES"=w1516:dbl, "T-RISE mins"=w1518:dbl)  [unwired: 3 out]
                    n872 = case shown="\"CHART TEST\", Default" w1519 {
                      tunnel: w1518 -> [_ _ w1528]
                      tunnel: [w1523 w1525 w1528] -> w1517
                      tunnel: w1516 -> [w1523 w1525 _]
                      tunnel: ["CHART TEST" "CYCLES" "T-RISE TEST"] -> w1515
                      frame "CHART TEST", Default {
                      }
                      frame "CYCLE TEST" {
                      }
                      frame "T-RISE TEST" {
                      }
                    }
                    n873 = Greater Or Equal?(x=w1520, y=w1516) -> (x >= y?=w1522:bool)
                    n874 = case shown="True" w1522 {
                      tunnel: w1517 -> [w1532 _]
                      tunnel: w1515 -> [w1531 _]
                      tunnel: w1514 -> [w1530 _]
                      tunnel: w1513 -> [w1529 _]
                      frame True {
                        n875 = stacked-sequence {
                          tunnel: w1532 -> [w1536 _]
                          tunnel: w1531 -> [w1534 _]
                          tunnel: w1530 -> [_ w1542]
                          tunnel: w1529 -> [w1533 _]
                          frame #0 {
                            n876 = Build Array(w1534) -> (w1537:string[])
                            n877 = Build Array(w1536) -> (w1535:dbl[])
                            n878 = TDMS Write(0:w1533, 5:"TEST PASS", 7:w1537, 9:w1535) -> (15:w1539:errorcluster)  [unwired: 2 in, 3 out]
                            n879 = local write "data file error"(w1539) -> ()
                          }
                          frame #1 {
                            n880 = Bundle(cluster=w1542, "STATUS"="CYCLE PASS") -> (w1540:T4)  [unwired: 2 in]
                            n881 = local write "LAB05-2 (RESULT)"(TRUE) -> ()
                            n882 = local write "LAB05-2 (DISP)"(w1540) -> ()
                          }
                        }
                      }
                      frame False {
                      }
                    }
                  }
                }
              }
            }
          }
          frame #5 {
            # "check if test cycles reached for temperature rise test"
            n883 = stacked-sequence {
              tunnel: w1573 -> [_ _ _ _ _ _ _ _ _ _]
              tunnel: w1572 -> [_ _ _ _ _ _ _ _ _ _]
              tunnel: w1571 -> [_ _ _ _ _ _ _ _ _ _]
              tunnel: w1570 -> [_ _ _ _ _ _ _ _ _ _]
              tunnel: w1569 -> [_ _ _ _ _ _ _ _ _ _]
              tunnel: w1568 -> [_ _ _ _ _ _ _ _ _ _]
              tunnel: w1567 -> [_ _ _ _ _ _ _ _ _ _]
              tunnel: w1566 -> [_ _ _ _ _ _ _ _ _ _]
              tunnel: w1565 -> [_ _ _ _ _ _ _ _ _ _]
              tunnel: w1564 -> [_ _ _ _ _ _ _ _ _ _]
              tunnel: w1563 -> [w1579 _ _ _ _ _ _ _ _ _]
              tunnel: w1553 -> [w1574 _ _ _ _ _ _ _ _ _]
              tunnel: w1562 -> [_ w1605 _ _ _ _ _ _ _ _]
              tunnel: w1561 -> [_ _ w1635 _ _ _ _ _ _ _]
              tunnel: w1560 -> [_ _ _ w1665 _ _ _ _ _ _]
              tunnel: w1559 -> [_ _ _ _ w1695 _ _ _ _ _]
              tunnel: w1558 -> [_ _ _ _ _ w1725 _ _ _ _]
              tunnel: w1557 -> [_ _ _ _ _ _ w1755 _ _ _]
              tunnel: w1556 -> [_ _ _ _ _ _ _ w1785 _ _]
              tunnel: w1555 -> [_ _ _ _ _ _ _ _ w1815 _]
              tunnel: w1554 -> [_ _ _ _ _ _ _ _ _ w1845]
              tunnel: w1552 -> [_ w1604 _ _ _ _ _ _ _ _]
              tunnel: w1551 -> [_ _ w1634 _ _ _ _ _ _ _]
              tunnel: w1550 -> [_ _ _ w1664 _ _ _ _ _ _]
              tunnel: w1549 -> [_ _ _ _ w1694 _ _ _ _ _]
              tunnel: w1548 -> [_ _ _ _ _ w1724 _ _ _ _]
              tunnel: w1547 -> [_ _ _ _ _ _ w1754 _ _ _]
              tunnel: w1546 -> [_ _ _ _ _ _ _ w1784 _ _]
              tunnel: w1545 -> [_ _ _ _ _ _ _ _ w1814 _]
              tunnel: w1544 -> [_ _ _ _ _ _ _ _ _ w1844]
              frame #0 {
                # "LAB01-1"
                n884 = Equal?(x=w1579, y=2) -> (x = y?=w1577:bool)
                n885 = local read "LAB01-1 (DISP)"() -> (w1580:T4)
                n886 = Unbundle(w1580) -> ("STATUS"=w1581:string)  [unwired: 2 out]
                n887 = Equal?(x=w1581, y="RUN") -> (x = y?=w1576:bool)
                n888 = And(x=w1576, y=w1577) -> (x .and. y?=w1575:bool)
                n889 = case shown="True" w1575 {
                  tunnel: w1580 -> [_ w1584]
                  tunnel: w1574 -> [_ w1587]
                  frame False {
                  }
                  frame True {
                    n890 = local read "LAB01-1 (SET)"() -> (w1586:T5)
                    n891 = local read "LAB01-1 (TDMS)"() -> (w1583:refnum<k34>)
                    n892 = Unbundle(w1584) -> ("CYCLE"=w1588:dbl)  [unwired: 2 out]
                    n893 = Unbundle(w1586) -> ("T-RISE mins"=w1585:dbl)  [unwired: 4 out]
                    n894 = Greater Or Equal?(x=w1588, y=w1587) -> (x >= y?=w1589:bool)
                    n895 = case shown="True" w1589 {
                      tunnel: w1585 -> [w1592 _]
                      tunnel: w1584 -> [w1591 _]
                      tunnel: w1583 -> [w1590 _]
                      frame True {
                        n896 = stacked-sequence {
                          tunnel: w1592 -> [w1595 _]
                          tunnel: w1591 -> [_ w1600]
                          tunnel: w1590 -> [w1593 _]
                          frame #0 {
                            n897 = Build Array("T-RISE") -> (w1597:string[])
                            n898 = Build Array(w1595) -> (w1596:dbl[])
                            n899 = TDMS Write(0:w1593, 5:"TEST PASS", 7:w1597, 9:w1596) -> (15:w1599:errorcluster)  [unwired: 2 in, 3 out]
                            n900 = local write "data file error"(w1599) -> ()
                          }
                          frame #1 {
                            n901 = Bundle(cluster=w1600, "STATUS"="T-RISE PASS") -> (w1602:T4)  [unwired: 2 in]
                            n902 = local write "LAB01-1 (RESULT)"(TRUE) -> ()
                            n903 = local write "LAB01-1 (DISP)"(w1602) -> ()
                          }
                        }
                      }
                      frame False {
                      }
                    }
                  }
                }
              }
              frame #1 {
                # "LAB01-2"
                n904 = Equal?(x=w1605, y=2) -> (x = y?=w1608:bool)
                n905 = local read "LAB01-2 (DISP)"() -> (w1610:T4)
                n906 = Unbundle(w1610) -> ("STATUS"=w1611:string)  [unwired: 2 out]
                n907 = Equal?(x=w1611, y="RUN") -> (x = y?=w1607:bool)
                n908 = And(x=w1607, y=w1608) -> (x .and. y?=w1606:bool)
                n909 = case shown="True" w1606 {
                  tunnel: w1610 -> [_ w1614]
                  tunnel: w1604 -> [_ w1617]
                  frame False {
                  }
                  frame True {
                    n910 = local read "LAB01-2 (SET)"() -> (w1616:T5)
                    n911 = local read "LAB01-2 (TDMS)"() -> (w1613:refnum<k34>)
                    n912 = Unbundle(w1614) -> ("CYCLE"=w1618:dbl)  [unwired: 2 out]
                    n913 = Unbundle(w1616) -> ("T-RISE mins"=w1615:dbl)  [unwired: 4 out]
                    n914 = Greater Or Equal?(x=w1618, y=w1617) -> (x >= y?=w1619:bool)
                    n915 = case shown="True" w1619 {
                      tunnel: w1615 -> [w1622 _]
                      tunnel: w1614 -> [w1621 _]
                      tunnel: w1613 -> [w1620 _]
                      frame True {
                        n916 = stacked-sequence {
                          tunnel: w1622 -> [w1625 _]
                          tunnel: w1621 -> [_ w1630]
                          tunnel: w1620 -> [w1623 _]
                          frame #0 {
                            n917 = Build Array("T-RISE") -> (w1627:string[])
                            n918 = Build Array(w1625) -> (w1626:dbl[])
                            n919 = TDMS Write(0:w1623, 5:"TEST PASS", 7:w1627, 9:w1626) -> (15:w1629:errorcluster)  [unwired: 2 in, 3 out]
                            n920 = local write "data file error"(w1629) -> ()
                          }
                          frame #1 {
                            n921 = Bundle(cluster=w1630, "STATUS"="T-RISE PASS") -> (w1632:T4)  [unwired: 2 in]
                            n922 = local write "LAB01-2 (RESULT)"(TRUE) -> ()
                            n923 = local write "LAB01-2 (DISP)"(w1632) -> ()
                          }
                        }
                      }
                      frame False {
                      }
                    }
                  }
                }
              }
              frame #2 {
                # "LAB02-1"
                n924 = Equal?(x=w1635, y=2) -> (x = y?=w1638:bool)
                n925 = local read "LAB02-1 (DISP)"() -> (w1640:T4)
                n926 = Unbundle(w1640) -> ("STATUS"=w1641:string)  [unwired: 2 out]
                n927 = Equal?(x=w1641, y="RUN") -> (x = y?=w1637:bool)
                n928 = And(x=w1637, y=w1638) -> (x .and. y?=w1636:bool)
                n929 = case shown="True" w1636 {
                  tunnel: w1640 -> [_ w1644]
                  tunnel: w1634 -> [_ w1647]
                  frame False {
                  }
                  frame True {
                    n930 = local read "LAB02-1 (SET)"() -> (w1646:T5)
                    n931 = local read "LAB02-1 (TDMS)"() -> (w1643:refnum<k34>)
                    n932 = Unbundle(w1644) -> ("CYCLE"=w1648:dbl)  [unwired: 2 out]
                    n933 = Unbundle(w1646) -> ("T-RISE mins"=w1645:dbl)  [unwired: 4 out]
                    n934 = Greater Or Equal?(x=w1648, y=w1647) -> (x >= y?=w1649:bool)
                    n935 = case shown="True" w1649 {
                      tunnel: w1645 -> [w1652 _]
                      tunnel: w1644 -> [w1651 _]
                      tunnel: w1643 -> [w1650 _]
                      frame True {
                        n936 = stacked-sequence {
                          tunnel: w1652 -> [w1655 _]
                          tunnel: w1651 -> [_ w1660]
                          tunnel: w1650 -> [w1653 _]
                          frame #0 {
                            n937 = Build Array("T-RISE") -> (w1657:string[])
                            n938 = Build Array(w1655) -> (w1656:dbl[])
                            n939 = TDMS Write(0:w1653, 5:"TEST PASS", 7:w1657, 9:w1656) -> (15:w1659:errorcluster)  [unwired: 2 in, 3 out]
                            n940 = local write "data file error"(w1659) -> ()
                          }
                          frame #1 {
                            n941 = Bundle(cluster=w1660, "STATUS"="T-RISE PASS") -> (w1662:T4)  [unwired: 2 in]
                            n942 = local write "LAB02-1 (RESULT)"(TRUE) -> ()
                            n943 = local write "LAB02-1 (DISP)"(w1662) -> ()
                          }
                        }
                      }
                      frame False {
                      }
                    }
                  }
                }
              }
              frame #3 {
                # "LAB02-2"
                n944 = Equal?(x=w1665, y=2) -> (x = y?=w1668:bool)
                n945 = local read "LAB02-2 (DISP)"() -> (w1670:T4)
                n946 = Unbundle(w1670) -> ("STATUS"=w1671:string)  [unwired: 2 out]
                n947 = Equal?(x=w1671, y="RUN") -> (x = y?=w1667:bool)
                n948 = And(x=w1667, y=w1668) -> (x .and. y?=w1666:bool)
                n949 = case shown="True" w1666 {
                  tunnel: w1670 -> [_ w1674]
                  tunnel: w1664 -> [_ w1677]
                  frame False {
                  }
                  frame True {
                    n950 = local read "LAB02-2 (SET)"() -> (w1676:T5)
                    n951 = local read "LAB02-2 (TDMS)"() -> (w1673:refnum<k34>)
                    n952 = Unbundle(w1674) -> ("CYCLE"=w1678:dbl)  [unwired: 2 out]
                    n953 = Unbundle(w1676) -> ("T-RISE mins"=w1675:dbl)  [unwired: 4 out]
                    n954 = Greater Or Equal?(x=w1678, y=w1677) -> (x >= y?=w1679:bool)
                    n955 = case shown="True" w1679 {
                      tunnel: w1675 -> [w1682 _]
                      tunnel: w1674 -> [w1681 _]
                      tunnel: w1673 -> [w1680 _]
                      frame True {
                        n956 = stacked-sequence {
                          tunnel: w1682 -> [w1685 _]
                          tunnel: w1681 -> [_ w1690]
                          tunnel: w1680 -> [w1683 _]
                          frame #0 {
                            n957 = Build Array("T-RISE") -> (w1687:string[])
                            n958 = Build Array(w1685) -> (w1686:dbl[])
                            n959 = TDMS Write(0:w1683, 5:"TEST PASS", 7:w1687, 9:w1686) -> (15:w1689:errorcluster)  [unwired: 2 in, 3 out]
                            n960 = local write "data file error"(w1689) -> ()
                          }
                          frame #1 {
                            n961 = Bundle(cluster=w1690, "STATUS"="T-RISE PASS") -> (w1692:T4)  [unwired: 2 in]
                            n962 = local write "LAB02-2 (RESULT)"(TRUE) -> ()
                            n963 = local write "LAB02-2 (DISP)"(w1692) -> ()
                          }
                        }
                      }
                      frame False {
                      }
                    }
                  }
                }
              }
              frame #4 {
                # "LAB03-1"
                n964 = Equal?(x=w1695, y=2) -> (x = y?=w1698:bool)
                n965 = local read "LAB03-1 (DISP)"() -> (w1700:T4)
                n966 = Unbundle(w1700) -> ("STATUS"=w1701:string)  [unwired: 2 out]
                n967 = Equal?(x=w1701, y="RUN") -> (x = y?=w1697:bool)
                n968 = And(x=w1697, y=w1698) -> (x .and. y?=w1696:bool)
                n969 = case shown="True" w1696 {
                  tunnel: w1700 -> [_ w1704]
                  tunnel: w1694 -> [_ w1707]
                  frame False {
                  }
                  frame True {
                    n970 = local read "LAB03-1 (SET)"() -> (w1706:T5)
                    n971 = local read "LAB03-1 (TDMS)"() -> (w1703:refnum<k34>)
                    n972 = Unbundle(w1704) -> ("CYCLE"=w1708:dbl)  [unwired: 2 out]
                    n973 = Unbundle(w1706) -> ("T-RISE mins"=w1705:dbl)  [unwired: 4 out]
                    n974 = Greater Or Equal?(x=w1708, y=w1707) -> (x >= y?=w1709:bool)
                    n975 = case shown="True" w1709 {
                      tunnel: w1705 -> [w1712 _]
                      tunnel: w1704 -> [w1711 _]
                      tunnel: w1703 -> [w1710 _]
                      frame True {
                        n976 = stacked-sequence {
                          tunnel: w1712 -> [w1715 _]
                          tunnel: w1711 -> [_ w1720]
                          tunnel: w1710 -> [w1713 _]
                          frame #0 {
                            n977 = Build Array("T-RISE") -> (w1717:string[])
                            n978 = Build Array(w1715) -> (w1716:dbl[])
                            n979 = TDMS Write(0:w1713, 5:"TEST PASS", 7:w1717, 9:w1716) -> (15:w1719:errorcluster)  [unwired: 2 in, 3 out]
                            n980 = local write "data file error"(w1719) -> ()
                          }
                          frame #1 {
                            n981 = Bundle(cluster=w1720, "STATUS"="T-RISE PASS") -> (w1722:T4)  [unwired: 2 in]
                            n982 = local write "LAB03-1 (RESULT)"(TRUE) -> ()
                            n983 = local write "LAB03-1 (DISP)"(w1722) -> ()
                          }
                        }
                      }
                      frame False {
                      }
                    }
                  }
                }
              }
              frame #5 {
                # "LAB03-2"
                n984 = Equal?(x=w1725, y=2) -> (x = y?=w1728:bool)
                n985 = local read "LAB03-2 (DISP)"() -> (w1730:T4)
                n986 = Unbundle(w1730) -> ("STATUS"=w1731:string)  [unwired: 2 out]
                n987 = Equal?(x=w1731, y="RUN") -> (x = y?=w1727:bool)
                n988 = And(x=w1727, y=w1728) -> (x .and. y?=w1726:bool)
                n989 = case shown="True" w1726 {
                  tunnel: w1730 -> [_ w1734]
                  tunnel: w1724 -> [_ w1737]
                  frame False {
                  }
                  frame True {
                    n990 = local read "LAB03-2 (SET)"() -> (w1736:T5)
                    n991 = local read "LAB03-2 (TDMS)"() -> (w1733:refnum<k34>)
                    n992 = Unbundle(w1734) -> ("CYCLE"=w1738:dbl)  [unwired: 2 out]
                    n993 = Unbundle(w1736) -> ("T-RISE mins"=w1735:dbl)  [unwired: 4 out]
                    n994 = Greater Or Equal?(x=w1738, y=w1737) -> (x >= y?=w1739:bool)
                    n995 = case shown="True" w1739 {
                      tunnel: w1735 -> [w1742 _]
                      tunnel: w1734 -> [w1741 _]
                      tunnel: w1733 -> [w1740 _]
                      frame True {
                        n996 = stacked-sequence {
                          tunnel: w1742 -> [w1745 _]
                          tunnel: w1741 -> [_ w1750]
                          tunnel: w1740 -> [w1743 _]
                          frame #0 {
                            n997 = Build Array("T-RISE") -> (w1747:string[])
                            n998 = Build Array(w1745) -> (w1746:dbl[])
                            n999 = TDMS Write(0:w1743, 5:"TEST PASS", 7:w1747, 9:w1746) -> (15:w1749:errorcluster)  [unwired: 2 in, 3 out]
                            n1000 = local write "data file error"(w1749) -> ()
                          }
                          frame #1 {
                            n1001 = Bundle(cluster=w1750, "STATUS"="T-RISE PASS") -> (w1752:T4)  [unwired: 2 in]
                            n1002 = local write "LAB03-2 (RESULT)"(TRUE) -> ()
                            n1003 = local write "LAB03-2 (DISP)"(w1752) -> ()
                          }
                        }
                      }
                      frame False {
                      }
                    }
                  }
                }
              }
              frame #6 {
                # "LAB04-1"
                n1004 = Equal?(x=w1755, y=2) -> (x = y?=w1758:bool)
                n1005 = local read "LAB04-1 (DISP)"() -> (w1760:T4)
                n1006 = Unbundle(w1760) -> ("STATUS"=w1761:string)  [unwired: 2 out]
                n1007 = Equal?(x=w1761, y="RUN") -> (x = y?=w1757:bool)
                n1008 = And(x=w1757, y=w1758) -> (x .and. y?=w1756:bool)
                n1009 = case shown="True" w1756 {
                  tunnel: w1760 -> [_ w1764]
                  tunnel: w1754 -> [_ w1767]
                  frame False {
                  }
                  frame True {
                    n1010 = local read "LAB04-1 (SET)"() -> (w1766:T5)
                    n1011 = local read "LAB04-1 (TDMS)"() -> (w1763:refnum<k34>)
                    n1012 = Unbundle(w1764) -> ("CYCLE"=w1768:dbl)  [unwired: 2 out]
                    n1013 = Unbundle(w1766) -> ("T-RISE mins"=w1765:dbl)  [unwired: 4 out]
                    n1014 = Greater Or Equal?(x=w1768, y=w1767) -> (x >= y?=w1769:bool)
                    n1015 = case shown="True" w1769 {
                      tunnel: w1765 -> [w1772 _]
                      tunnel: w1764 -> [w1771 _]
                      tunnel: w1763 -> [w1770 _]
                      frame True {
                        n1016 = stacked-sequence {
                          tunnel: w1772 -> [w1775 _]
                          tunnel: w1771 -> [_ w1780]
                          tunnel: w1770 -> [w1773 _]
                          frame #0 {
                            n1017 = Build Array("T-RISE") -> (w1777:string[])
                            n1018 = Build Array(w1775) -> (w1776:dbl[])
                            n1019 = TDMS Write(0:w1773, 5:"TEST PASS", 7:w1777, 9:w1776) -> (15:w1779:errorcluster)  [unwired: 2 in, 3 out]
                            n1020 = local write "data file error"(w1779) -> ()
                          }
                          frame #1 {
                            n1021 = Bundle(cluster=w1780, "STATUS"="T-RISE PASS") -> (w1782:T4)  [unwired: 2 in]
                            n1022 = local write "LAB04-1 (RESULT)"(TRUE) -> ()
                            n1023 = local write "LAB04-1 (DISP)"(w1782) -> ()
                          }
                        }
                      }
                      frame False {
                      }
                    }
                  }
                }
              }
              frame #7 {
                # "LAB04-2"
                n1024 = Equal?(x=w1785, y=2) -> (x = y?=w1788:bool)
                n1025 = local read "LAB04-2 (DISP)"() -> (w1790:T4)
                n1026 = Unbundle(w1790) -> ("STATUS"=w1791:string)  [unwired: 2 out]
                n1027 = Equal?(x=w1791, y="RUN") -> (x = y?=w1787:bool)
                n1028 = And(x=w1787, y=w1788) -> (x .and. y?=w1786:bool)
                n1029 = case shown="True" w1786 {
                  tunnel: w1790 -> [_ w1794]
                  tunnel: w1784 -> [_ w1797]
                  frame False {
                  }
                  frame True {
                    n1030 = local read "LAB04-2 (SET)"() -> (w1796:T5)
                    n1031 = local read "LAB04-2 (TDMS)"() -> (w1793:refnum<k34>)
                    n1032 = Unbundle(w1794) -> ("CYCLE"=w1798:dbl)  [unwired: 2 out]
                    n1033 = Unbundle(w1796) -> ("T-RISE mins"=w1795:dbl)  [unwired: 4 out]
                    n1034 = Greater Or Equal?(x=w1798, y=w1797) -> (x >= y?=w1799:bool)
                    n1035 = case shown="True" w1799 {
                      tunnel: w1795 -> [w1802 _]
                      tunnel: w1794 -> [w1801 _]
                      tunnel: w1793 -> [w1800 _]
                      frame True {
                        n1036 = stacked-sequence {
                          tunnel: w1802 -> [w1805 _]
                          tunnel: w1801 -> [_ w1810]
                          tunnel: w1800 -> [w1803 _]
                          frame #0 {
                            n1037 = Build Array("T-RISE") -> (w1807:string[])
                            n1038 = Build Array(w1805) -> (w1806:dbl[])
                            n1039 = TDMS Write(0:w1803, 5:"TEST PASS", 7:w1807, 9:w1806) -> (15:w1809:errorcluster)  [unwired: 2 in, 3 out]
                            n1040 = local write "data file error"(w1809) -> ()
                          }
                          frame #1 {
                            n1041 = Bundle(cluster=w1810, "STATUS"="T-RISE PASS") -> (w1812:T4)  [unwired: 2 in]
                            n1042 = local write "LAB04-2 (RESULT)"(TRUE) -> ()
                            n1043 = local write "LAB04-2 (DISP)"(w1812) -> ()
                          }
                        }
                      }
                      frame False {
                      }
                    }
                  }
                }
              }
              frame #8 {
                # "LAB05-1"
                n1044 = Equal?(x=w1815, y=2) -> (x = y?=w1818:bool)
                n1045 = local read "LAB05-1 (DISP)"() -> (w1820:T4)
                n1046 = Unbundle(w1820) -> ("STATUS"=w1821:string)  [unwired: 2 out]
                n1047 = Equal?(x=w1821, y="RUN") -> (x = y?=w1817:bool)
                n1048 = And(x=w1817, y=w1818) -> (x .and. y?=w1816:bool)
                n1049 = case shown="True" w1816 {
                  tunnel: w1820 -> [_ w1824]
                  tunnel: w1814 -> [_ w1827]
                  frame False {
                  }
                  frame True {
                    n1050 = local read "LAB05-1 (SET)"() -> (w1826:T5)
                    n1051 = local read "LAB05-1 (TDMS)"() -> (w1823:refnum<k34>)
                    n1052 = Unbundle(w1824) -> ("CYCLE"=w1828:dbl)  [unwired: 2 out]
                    n1053 = Unbundle(w1826) -> ("T-RISE mins"=w1825:dbl)  [unwired: 4 out]
                    n1054 = Greater Or Equal?(x=w1828, y=w1827) -> (x >= y?=w1829:bool)
                    n1055 = case shown="True" w1829 {
                      tunnel: w1825 -> [w1832 _]
                      tunnel: w1824 -> [w1831 _]
                      tunnel: w1823 -> [w1830 _]
                      frame True {
                        n1056 = stacked-sequence {
                          tunnel: w1832 -> [w1835 _]
                          tunnel: w1831 -> [_ w1840]
                          tunnel: w1830 -> [w1833 _]
                          frame #0 {
                            n1057 = Build Array("T-RISE") -> (w1837:string[])
                            n1058 = Build Array(w1835) -> (w1836:dbl[])
                            n1059 = TDMS Write(0:w1833, 5:"TEST PASS", 7:w1837, 9:w1836) -> (15:w1839:errorcluster)  [unwired: 2 in, 3 out]
                            n1060 = local write "data file error"(w1839) -> ()
                          }
                          frame #1 {
                            n1061 = Bundle(cluster=w1840, "STATUS"="T-RISE PASS") -> (w1842:T4)  [unwired: 2 in]
                            n1062 = local write "LAB05-1 (RESULT)"(TRUE) -> ()
                            n1063 = local write "LAB05-1 (DISP)"(w1842) -> ()
                          }
                        }
                      }
                      frame False {
                      }
                    }
                  }
                }
              }
              frame #9 {
                # "LAB05-2"
                n1064 = Equal?(x=w1845, y=2) -> (x = y?=w1848:bool)
                n1065 = local read "LAB05-2 (DISP)"() -> (w1850:T4)
                n1066 = Unbundle(w1850) -> ("STATUS"=w1851:string)  [unwired: 2 out]
                n1067 = Equal?(x=w1851, y="RUN") -> (x = y?=w1847:bool)
                n1068 = And(x=w1847, y=w1848) -> (x .and. y?=w1846:bool)
                n1069 = case shown="True" w1846 {
                  tunnel: w1850 -> [_ w1854]
                  tunnel: w1844 -> [_ w1857]
                  frame False {
                  }
                  frame True {
                    n1070 = local read "LAB05-2 (SET)"() -> (w1856:T5)
                    n1071 = local read "LAB05-2 (TDMS)"() -> (w1853:refnum<k34>)
                    n1072 = Unbundle(w1854) -> ("CYCLE"=w1858:dbl)  [unwired: 2 out]
                    n1073 = Unbundle(w1856) -> ("T-RISE mins"=w1855:dbl)  [unwired: 4 out]
                    n1074 = Greater Or Equal?(x=w1858, y=w1857) -> (x >= y?=w1859:bool)
                    n1075 = case shown="True" w1859 {
                      tunnel: w1855 -> [w1862 _]
                      tunnel: w1854 -> [w1861 _]
                      tunnel: w1853 -> [w1860 _]
                      frame True {
                        n1076 = stacked-sequence {
                          tunnel: w1862 -> [w1865 _]
                          tunnel: w1861 -> [_ w1870]
                          tunnel: w1860 -> [w1863 _]
                          frame #0 {
                            n1077 = Build Array("T-RISE") -> (w1867:string[])
                            n1078 = Build Array(w1865) -> (w1866:dbl[])
                            n1079 = TDMS Write(0:w1863, 5:"TEST PASS", 7:w1867, 9:w1866) -> (15:w1869:errorcluster)  [unwired: 2 in, 3 out]
                            n1080 = local write "data file error"(w1869) -> ()
                          }
                          frame #1 {
                            n1081 = Bundle(cluster=w1870, "STATUS"="T-RISE PASS") -> (w1872:T4)  [unwired: 2 in]
                            n1082 = local write "LAB05-2 (RESULT)"(TRUE) -> ()
                            n1083 = local write "LAB05-2 (DISP)"(w1872) -> ()
                          }
                        }
                      }
                      frame False {
                      }
                    }
                  }
                }
              }
            }
          }
          frame #6 {
            # "disable functions"
            n1084 = stacked-sequence {
              tunnel: w1883 -> [w1897 _ w1953]
              tunnel: w1882 -> [w1892 _ w1952]
              tunnel: w1881 -> [w1891 _ w1951]
              tunnel: w1880 -> [w1889 _ w1950]
              tunnel: w1879 -> [w1890 _ w1949]
              tunnel: w1878 -> [_ w1914 w1948]
              tunnel: w1877 -> [_ w1915 w1947]
              tunnel: w1876 -> [_ w1916 w1946]
              tunnel: w1875 -> [_ w1917 w1945]
              tunnel: w1874 -> [_ w1918 w1944]
              frame #0 {
                n1085 = Select(t=2, s=w1889, f=0) -> (s? t:f=w1885:i32)
                n1086 = Select(t=2, s=w1891, f=0) -> (s? t:f=w1886:i32)
                n1087 = Select(t=2, s=w1890, f=0) -> (s? t:f=w1884:i32)
                n1088 = Select(t=2, s=w1897, f=0) -> (s? t:f=w1888:i32)
                n1089 = Select(t=2, s=w1892, f=0) -> (s? t:f=w1887:i32)
                n1090 = property on="LAB02-2 SELECT" class="RadioBtnsControl (strict)"("DisabledEnum"=w1885) -> ()  [unwired: 2 in, 2 out]
                n1091 = property on="LAB02-1 SELECT" class="RadioBtnsControl (strict)"("DisabledEnum"=w1886) -> ()  [unwired: 2 in, 2 out]
                n1092 = property on="LAB03-1 SELECT" class="RadioBtnsControl (strict)"("DisabledEnum"=w1884) -> ()  [unwired: 2 in, 2 out]
                n1093 = property on="LAB01-1 SELECT" class="RadioBtnsControl (strict)"("DisabledEnum"=w1888) -> ()  [unwired: 2 in, 2 out]
                n1094 = property on="LAB01-2 SELECT" class="RadioBtnsControl (strict)"("DisabledEnum"=w1887) -> ()  [unwired: 2 in, 2 out]
                n1095 = Not(x=w1897) -> (.not. x?=w1898:bool)
                n1096 = property on="LAB01-1 (RESULT)" class="Bool (strict)"("Visible"=w1898) -> ()  [unwired: 2 in, 2 out]
                n1097 = Not(x=w1892) -> (.not. x?=w1896:bool)
                n1098 = Not(x=w1891) -> (.not. x?=w1895:bool)
                n1099 = Not(x=w1889) -> (.not. x?=w1894:bool)
                n1100 = property on="LAB01-2 (RESULT)" class="Bool (strict)"("Visible"=w1896) -> ()  [unwired: 2 in, 2 out]
                n1101 = Not(x=w1890) -> (.not. x?=w1893:bool)
                n1102 = property on="LAB02-1 (RESULT)" class="Bool (strict)"("Visible"=w1895) -> ()  [unwired: 2 in, 2 out]
                n1103 = property on="LAB02-2 (RESULT)" class="Bool (strict)"("Visible"=w1894) -> ()  [unwired: 2 in, 2 out]
                n1104 = property on="LAB03-1 (RESULT)" class="Bool (strict)"("Visible"=w1893) -> ()  [unwired: 2 in, 2 out]
                n1105 = property on="LAB01-1 (SET)" class="Clust (strict)"("DisabledEnum"=w1888) -> ()  [unwired: 2 in, 2 out]
                n1106 = property on="LAB01-2 (SET)" class="Clust (strict)"("DisabledEnum"=w1887) -> ()  [unwired: 2 in, 2 out]
                n1107 = property on="LAB02-1 (SET)" class="Clust (strict)"("DisabledEnum"=w1886) -> ()  [unwired: 2 in, 2 out]
                n1108 = property on="LAB02-2 (SET)" class="Clust (strict)"("DisabledEnum"=w1885) -> ()  [unwired: 2 in, 2 out]
                n1109 = property on="LAB03-1 (SET)" class="Clust (strict)"("DisabledEnum"=w1884) -> ()  [unwired: 2 in, 2 out]
                n1110 = property on="LAB01-1 (O/I)" class="Bool (strict)"("DisabledEnum"=w1888) -> ()  [unwired: 2 in, 2 out]
                n1111 = property on="LAB01-2 (O/I)" class="Bool (strict)"("DisabledEnum"=w1887) -> ()  [unwired: 2 in, 2 out]
                n1112 = property on="LAB02-1 (O/I)" class="Bool (strict)"("DisabledEnum"=w1886) -> ()  [unwired: 2 in, 2 out]
                n1113 = property on="LAB02-2 (O/I)" class="Bool (strict)"("DisabledEnum"=w1885) -> ()  [unwired: 2 in, 2 out]
                n1114 = property on="LAB03-1 (O/I)" class="Bool (strict)"("DisabledEnum"=w1884) -> ()  [unwired: 2 in, 2 out]
              }
              frame #1 {
                n1115 = Select(t=2, s=w1918, f=0) -> (s? t:f=w1909:i32)
                n1116 = Select(t=2, s=w1917, f=0) -> (s? t:f=w1910:i32)
                n1117 = Select(t=2, s=w1914, f=0) -> (s? t:f=w1913:i32)
                n1118 = Select(t=2, s=w1915, f=0) -> (s? t:f=w1912:i32)
                n1119 = Select(t=2, s=w1916, f=0) -> (s? t:f=w1911:i32)
                n1120 = property on="LAB05-2 SELECT" class="RadioBtnsControl (strict)"("DisabledEnum"=w1909) -> ()  [unwired: 2 in, 2 out]
                n1121 = property on="LAB05-1 SELECT" class="RadioBtnsControl (strict)"("DisabledEnum"=w1910) -> ()  [unwired: 2 in, 2 out]
                n1122 = property on="LAB03-2 SELECT" class="RadioBtnsControl (strict)"("DisabledEnum"=w1913) -> ()  [unwired: 2 in, 2 out]
                n1123 = property on="LAB04-1 SELECT" class="RadioBtnsControl (strict)"("DisabledEnum"=w1912) -> ()  [unwired: 2 in, 2 out]
                n1124 = property on="LAB04-2 SELECT" class="RadioBtnsControl (strict)"("DisabledEnum"=w1911) -> ()  [unwired: 2 in, 2 out]
                n1125 = property on="LAB05-2 (SET)" class="Clust (strict)"("DisabledEnum"=w1909) -> ()  [unwired: 2 in, 2 out]
                n1126 = property on="LAB05-1 (SET)" class="Clust (strict)"("DisabledEnum"=w1910) -> ()  [unwired: 2 in, 2 out]
                n1127 = property on="LAB03-2 (SET)" class="Clust (strict)"("DisabledEnum"=w1913) -> ()  [unwired: 2 in, 2 out]
                n1128 = property on="LAB04-1 (SET)" class="Clust (strict)"("DisabledEnum"=w1912) -> ()  [unwired: 2 in, 2 out]
                n1129 = property on="LAB04-2 (SET)" class="Clust (strict)"("DisabledEnum"=w1911) -> ()  [unwired: 2 in, 2 out]
                n1130 = property on="LAB05-2 (O/I)" class="Bool (strict)"("DisabledEnum"=w1909) -> ()  [unwired: 2 in, 2 out]
                n1131 = property on="LAB05-1 (O/I)" class="Bool (strict)"("DisabledEnum"=w1910) -> ()  [unwired: 2 in, 2 out]
                n1132 = property on="LAB04-1 (O/I)" class="Bool (strict)"("DisabledEnum"=w1912) -> ()  [unwired: 2 in, 2 out]
                n1133 = property on="LAB04-2 (O/I)" class="Bool (strict)"("DisabledEnum"=w1911) -> ()  [unwired: 2 in, 2 out]
                n1134 = property on="LAB03-2 (O/I)" class="Bool (strict)"("DisabledEnum"=w1913) -> ()  [unwired: 2 in, 2 out]
                n1135 = Not(x=w1918) -> (.not. x?=w1919:bool)
                n1136 = Not(x=w1917) -> (.not. x?=w1920:bool)
                n1137 = Not(x=w1916) -> (.not. x?=w1921:bool)
                n1138 = property on="LAB05-2 (RESULT)" class="Bool (strict)"("Visible"=w1919) -> ()  [unwired: 2 in, 2 out]
                n1139 = property on="LAB05-1 (RESULT)" class="Bool (strict)"("Visible"=w1920) -> ()  [unwired: 2 in, 2 out]
                n1140 = Not(x=w1915) -> (.not. x?=w1922:bool)
                n1141 = property on="LAB04-2 (RESULT)" class="Bool (strict)"("Visible"=w1921) -> ()  [unwired: 2 in, 2 out]
                n1142 = Not(x=w1914) -> (.not. x?=w1923:bool)
                n1143 = property on="LAB04-1 (RESULT)" class="Bool (strict)"("Visible"=w1922) -> ()  [unwired: 2 in, 2 out]
                n1144 = property on="LAB03-2 (RESULT)" class="Bool (strict)"("Visible"=w1923) -> ()  [unwired: 2 in, 2 out]
              }
              frame #2 {
                # "disable calibrate if any test running"
                n1145 = Or(x=w1945, y=w1944) -> (x .or. y?=w1938:bool)
                n1146 = Or(x=w1947, y=w1946) -> (x .or. y?=w1940:bool)
                n1147 = Or(x=w1951, y=w1950) -> (x .or. y?=w1942:bool)
                n1148 = Or(x=w1949, y=w1948) -> (x .or. y?=w1941:bool)
                n1149 = Or(x=w1953, y=w1952) -> (x .or. y?=w1943:bool)
                n1150 = Or(x=w1941, y=w1940) -> (x .or. y?=w1939:bool)
                n1151 = Or(x=w1943, y=w1942) -> (x .or. y?=w1937:bool)
                n1152 = Or(x=w1939, y=w1938) -> (x .or. y?=w1936:bool)
                n1153 = Or(x=w1937, y=w1936) -> (x .or. y?=w1935:bool)
                n1154 = case shown="False" w1935 {
                  tunnel: [0 2] -> w1934
                  frame False {
                  }
                  frame True {
                  }
                }
                n1155 = property on="CALIBRATE" class="Bool (strict)"("DisabledEnum"=w1934) -> ()  [unwired: 2 in, 2 out]
              }
            }
          }
          frame #7 {
            # "end test & close test files"
            n1156 = stacked-sequence {
              tunnel: w1965 -> [w1967 _ _ _ _ _ _ _ _ _]
              tunnel: w1966 -> [_ w1982 _ _ _ _ _ _ _ _]
              tunnel: w1964 -> [_ _ w1997 _ _ _ _ _ _ _]
              tunnel: w1963 -> [_ _ _ w2012 _ _ _ _ _ _]
              tunnel: w1962 -> [_ _ _ _ w2027 _ _ _ _ _]
              tunnel: w1961 -> [_ _ _ _ _ w2042 _ _ _ _]
              tunnel: w1960 -> [_ _ _ _ _ _ w2057 _ _ _]
              tunnel: w1959 -> [_ _ _ _ _ _ _ w2072 _ _]
              tunnel: w1958 -> [_ _ _ _ _ _ _ _ w2087 _]
              tunnel: w1957 -> [_ _ _ _ _ _ _ _ _ w2102]
              frame #0 {
                # "LAB01-1"
                n1157 = case shown="True" w1967 {
                  frame False {
                  }
                  frame True {
                    n1158 = local read "LAB01-1 (DISP)"() -> (w1970:T4)
                    n1159 = local read "LAB01-1 (TDMS)"() -> (w1969:refnum<k34>)
                    n1160 = Unbundle(w1970) -> ("STATUS"=w1968:string)  [unwired: 2 out]
                    n1161 = Not Equal?(x=w1968, y="RUN") -> (x != y?=w1971:bool)
                    n1162 = case shown="True" w1971 {
                      tunnel: w1970 -> [_ w1974]
                      tunnel: w1969 -> [_ w1973]
                      frame False {
                      }
                      frame True {
                        n1163 = stacked-sequence {
                          tunnel: w1974 -> [w1976 _ _]
                          tunnel: w1973 -> [_ w1978 _]
                          frame #0 {
                            (unwired) "END"
                            n1164 = Bundle(cluster=w1976) -> (w1975:T4)  [unwired: 3 in]
                            n1165 = local write "LAB01-1 (DISP)"(w1975) -> ()
                            n1166 = local write "LAB01-1RUN"(FALSE) -> ()
                          }
                          frame #1 {
                            n1167 = TDMS Close(11:w1978) -> (0:w1979:errorcluster)  [unwired: 1 in, 1 out]
                            n1168 = local write "data file error"(w1979) -> ()
                          }
                          frame #2 {
                            n1169 = call "Save data file to network drive v1.vi"("panel id"="LAB01-1") -> ("network file save error"=w1980:errorcluster)  [unwired: 9 in, 1 out]
                            n1170 = local write "data file error"(w1980) -> ()
                          }
                        }
                      }
                    }
                  }
                }
              }
              frame #1 {
                # "LAB01-2"
                n1171 = case shown="True" w1982 {
                  frame False {
                  }
                  frame True {
                    n1172 = local read "LAB01-2 (DISP)"() -> (w1984:T4)
                    n1173 = local read "LAB01-2 (TDMS)"() -> (w1983:refnum<k34>)
                    n1174 = Unbundle(w1984) -> ("STATUS"=w1985:string)  [unwired: 2 out]
                    n1175 = Not Equal?(x=w1985, y="RUN") -> (x != y?=w1986:bool)
                    n1176 = case shown="True" w1986 {
                      tunnel: w1984 -> [_ w1989]
                      tunnel: w1983 -> [_ w1988]
                      frame False {
                      }
                      frame True {
                        n1177 = stacked-sequence {
                          tunnel: w1989 -> [w1991 _ _]
                          tunnel: w1988 -> [_ w1993 _]
                          frame #0 {
                            (unwired) "END"
                            n1178 = Bundle(cluster=w1991) -> (w1992:T4)  [unwired: 3 in]
                            n1179 = local write "LAB01-2 RUN"(FALSE) -> ()
                            n1180 = local write "LAB01-2 (DISP)"(w1992) -> ()
                          }
                          frame #1 {
                            n1181 = TDMS Close(11:w1993) -> (0:w1994:errorcluster)  [unwired: 1 in, 1 out]
                            n1182 = local write "data file error"(w1994) -> ()
                          }
                          frame #2 {
                            n1183 = call "Save data file to network drive v1.vi"("panel id"="LAB01-2") -> ("network file save error"=w1995:errorcluster)  [unwired: 9 in, 1 out]
                            n1184 = local write "data file error"(w1995) -> ()
                          }
                        }
                      }
                    }
                  }
                }
              }
              frame #2 {
                # "LAB02-1"
                n1185 = case shown="True" w1997 {
                  frame False {
                  }
                  frame True {
                    n1186 = local read "LAB02-1 (DISP)"() -> (w1999:T4)
                    n1187 = local read "LAB02-1 (TDMS)"() -> (w1998:refnum<k34>)
                    n1188 = Unbundle(w1999) -> ("STATUS"=w2000:string)  [unwired: 2 out]
                    n1189 = Not Equal?(x=w2000, y="RUN") -> (x != y?=w2001:bool)
                    n1190 = case shown="True" w2001 {
                      tunnel: w1999 -> [_ w2004]
                      tunnel: w1998 -> [_ w2003]
                      frame False {
                      }
                      frame True {
                        n1191 = stacked-sequence {
                          tunnel: w2004 -> [w2006 _ _]
                          tunnel: w2003 -> [_ w2008 _]
                          frame #0 {
                            (unwired) "END"
                            n1192 = Bundle(cluster=w2006) -> (w2007:T4)  [unwired: 3 in]
                            n1193 = local write "LAB02-1 RUN"(FALSE) -> ()
                            n1194 = local write "LAB02-1 (DISP)"(w2007) -> ()
                          }
                          frame #1 {
                            n1195 = TDMS Close(11:w2008) -> (0:w2009:errorcluster)  [unwired: 1 in, 1 out]
                            n1196 = local write "data file error"(w2009) -> ()
                          }
                          frame #2 {
                            n1197 = call "Save data file to network drive v1.vi"("panel id"="LAB02-1") -> ("network file save error"=w2010:errorcluster)  [unwired: 9 in, 1 out]
                            n1198 = local write "data file error"(w2010) -> ()
                          }
                        }
                      }
                    }
                  }
                }
              }
              frame #3 {
                # "LAB02-2"
                n1199 = case shown="True" w2012 {
                  frame False {
                  }
                  frame True {
                    n1200 = local read "LAB02-2 (DISP)"() -> (w2014:T4)
                    n1201 = local read "LAB02-2 (TDMS)"() -> (w2013:refnum<k34>)
                    n1202 = Unbundle(w2014) -> ("STATUS"=w2015:string)  [unwired: 2 out]
                    n1203 = Not Equal?(x=w2015, y="RUN") -> (x != y?=w2016:bool)
                    n1204 = case shown="True" w2016 {
                      tunnel: w2014 -> [_ w2019]
                      tunnel: w2013 -> [_ w2018]
                      frame False {
                      }
                      frame True {
                        n1205 = stacked-sequence {
                          tunnel: w2019 -> [w2021 _ _]
                          tunnel: w2018 -> [_ w2023 _]
                          frame #0 {
                            (unwired) "END"
                            n1206 = Bundle(cluster=w2021) -> (w2022:T4)  [unwired: 3 in]
                            n1207 = local write "LAB02-2 RUN"(FALSE) -> ()
                            n1208 = local write "LAB02-2 (DISP)"(w2022) -> ()
                          }
                          frame #1 {
                            n1209 = TDMS Close(11:w2023) -> (0:w2024:errorcluster)  [unwired: 1 in, 1 out]
                            n1210 = local write "data file error"(w2024) -> ()
                          }
                          frame #2 {
                            n1211 = call "Save data file to network drive v1.vi"("panel id"="LAB02-2") -> ("network file save error"=w2025:errorcluster)  [unwired: 9 in, 1 out]
                            n1212 = local write "data file error"(w2025) -> ()
                          }
                        }
                      }
                    }
                  }
                }
              }
              frame #4 {
                # "LAB03-1"
                n1213 = case shown="True" w2027 {
                  frame False {
                  }
                  frame True {
                    n1214 = local read "LAB03-1 (DISP)"() -> (w2029:T4)
                    n1215 = local read "LAB03-1 (TDMS)"() -> (w2028:refnum<k34>)
                    n1216 = Unbundle(w2029) -> ("STATUS"=w2030:string)  [unwired: 2 out]
                    n1217 = Not Equal?(x=w2030, y="RUN") -> (x != y?=w2031:bool)
                    n1218 = case shown="True" w2031 {
                      tunnel: w2029 -> [_ w2034]
                      tunnel: w2028 -> [_ w2033]
                      frame False {
                      }
                      frame True {
                        n1219 = stacked-sequence {
                          tunnel: w2034 -> [w2036 _ _]
                          tunnel: w2033 -> [_ w2038 _]
                          frame #0 {
                            (unwired) "END"
                            n1220 = Bundle(cluster=w2036) -> (w2037:T4)  [unwired: 3 in]
                            n1221 = local write "LAB03-1 RUN"(FALSE) -> ()
                            n1222 = local write "LAB03-1 (DISP)"(w2037) -> ()
                          }
                          frame #1 {
                            n1223 = TDMS Close(11:w2038) -> (0:w2039:errorcluster)  [unwired: 1 in, 1 out]
                            n1224 = local write "data file error"(w2039) -> ()
                          }
                          frame #2 {
                            n1225 = call "Save data file to network drive v1.vi"("panel id"="LAB03-1") -> ("network file save error"=w2040:errorcluster)  [unwired: 9 in, 1 out]
                            n1226 = local write "data file error"(w2040) -> ()
                          }
                        }
                      }
                    }
                  }
                }
              }
              frame #5 {
                # "LAB03-2"
                n1227 = case shown="True" w2042 {
                  frame False {
                  }
                  frame True {
                    n1228 = local read "LAB03-2 (DISP)"() -> (w2044:T4)
                    n1229 = local read "LAB03-2 (TDMS)"() -> (w2043:refnum<k34>)
                    n1230 = Unbundle(w2044) -> ("STATUS"=w2045:string)  [unwired: 2 out]
                    n1231 = Not Equal?(x=w2045, y="RUN") -> (x != y?=w2046:bool)
                    n1232 = case shown="True" w2046 {
                      tunnel: w2044 -> [_ w2049]
                      tunnel: w2043 -> [_ w2048]
                      frame False {
                      }
                      frame True {
                        n1233 = stacked-sequence {
                          tunnel: w2049 -> [w2051 _ _]
                          tunnel: w2048 -> [_ w2053 _]
                          frame #0 {
                            (unwired) "END"
                            n1234 = Bundle(cluster=w2051) -> (w2052:T4)  [unwired: 3 in]
                            n1235 = local write "LAB03-2 RUN"(FALSE) -> ()
                            n1236 = local write "LAB03-2 (DISP)"(w2052) -> ()
                          }
                          frame #1 {
                            n1237 = TDMS Close(11:w2053) -> (0:w2054:errorcluster)  [unwired: 1 in, 1 out]
                            n1238 = local write "data file error"(w2054) -> ()
                          }
                          frame #2 {
                            n1239 = call "Save data file to network drive v1.vi"("panel id"="LAB03-2") -> ("network file save error"=w2055:errorcluster)  [unwired: 9 in, 1 out]
                            n1240 = local write "data file error"(w2055) -> ()
                          }
                        }
                      }
                    }
                  }
                }
              }
              frame #6 {
                # "LAB04-1"
                n1241 = case shown="True" w2057 {
                  frame False {
                  }
                  frame True {
                    n1242 = local read "LAB04-1 (DISP)"() -> (w2059:T4)
                    n1243 = local read "LAB04-1 (TDMS)"() -> (w2058:refnum<k34>)
                    n1244 = Unbundle(w2059) -> ("STATUS"=w2060:string)  [unwired: 2 out]
                    n1245 = Not Equal?(x=w2060, y="RUN") -> (x != y?=w2061:bool)
                    n1246 = case shown="True" w2061 {
                      tunnel: w2059 -> [_ w2064]
                      tunnel: w2058 -> [_ w2063]
                      frame False {
                      }
                      frame True {
                        n1247 = stacked-sequence {
                          tunnel: w2064 -> [w2066 _ _]
                          tunnel: w2063 -> [_ w2068 _]
                          frame #0 {
                            (unwired) "END"
                            n1248 = Bundle(cluster=w2066) -> (w2067:T4)  [unwired: 3 in]
                            n1249 = local write "LAB04-1 RUN"(FALSE) -> ()
                            n1250 = local write "LAB04-1 (DISP)"(w2067) -> ()
                          }
                          frame #1 {
                            n1251 = TDMS Close(11:w2068) -> (0:w2069:errorcluster)  [unwired: 1 in, 1 out]
                            n1252 = local write "data file error"(w2069) -> ()
                          }
                          frame #2 {
                            n1253 = call "Save data file to network drive v1.vi"("panel id"="LAB04-1") -> ("network file save error"=w2070:errorcluster)  [unwired: 9 in, 1 out]
                            n1254 = local write "data file error"(w2070) -> ()
                          }
                        }
                      }
                    }
                  }
                }
              }
              frame #7 {
                # "LAB04-2"
                n1255 = case shown="True" w2072 {
                  frame False {
                  }
                  frame True {
                    n1256 = local read "LAB04-2 (DISP)"() -> (w2074:T4)
                    n1257 = local read "LAB04-2 (TDMS)"() -> (w2073:refnum<k34>)
                    n1258 = Unbundle(w2074) -> ("STATUS"=w2075:string)  [unwired: 2 out]
                    n1259 = Not Equal?(x=w2075, y="RUN") -> (x != y?=w2076:bool)
                    n1260 = case shown="True" w2076 {
                      tunnel: w2074 -> [_ w2079]
                      tunnel: w2073 -> [_ w2078]
                      frame False {
                      }
                      frame True {
                        n1261 = stacked-sequence {
                          tunnel: w2079 -> [w2081 _ _]
                          tunnel: w2078 -> [_ w2083 _]
                          frame #0 {
                            (unwired) "END"
                            n1262 = Bundle(cluster=w2081) -> (w2082:T4)  [unwired: 3 in]
                            n1263 = local write "LAB04-2 RUN"(FALSE) -> ()
                            n1264 = local write "LAB04-2 (DISP)"(w2082) -> ()
                          }
                          frame #1 {
                            n1265 = TDMS Close(11:w2083) -> (0:w2084:errorcluster)  [unwired: 1 in, 1 out]
                            n1266 = local write "data file error"(w2084) -> ()
                          }
                          frame #2 {
                            n1267 = call "Save data file to network drive v1.vi"("panel id"="LAB04-2") -> ("network file save error"=w2085:errorcluster)  [unwired: 9 in, 1 out]
                            n1268 = local write "data file error"(w2085) -> ()
                          }
                        }
                      }
                    }
                  }
                }
              }
              frame #8 {
                # "LAB05-1"
                n1269 = case shown="True" w2087 {
                  frame False {
                  }
                  frame True {
                    n1270 = local read "LAB05-1 (DISP)"() -> (w2089:T4)
                    n1271 = local read "LAB05-1 (TDMS)"() -> (w2088:refnum<k34>)
                    n1272 = Unbundle(w2089) -> ("STATUS"=w2090:string)  [unwired: 2 out]
                    n1273 = Not Equal?(x=w2090, y="RUN") -> (x != y?=w2091:bool)
                    n1274 = case shown="True" w2091 {
                      tunnel: w2089 -> [_ w2094]
                      tunnel: w2088 -> [_ w2093]
                      frame False {
                      }
                      frame True {
                        n1275 = stacked-sequence {
                          tunnel: w2094 -> [w2096 _ _]
                          tunnel: w2093 -> [_ w2098 _]
                          frame #0 {
                            (unwired) "END"
                            n1276 = Bundle(cluster=w2096) -> (w2097:T4)  [unwired: 3 in]
                            n1277 = local write "LAB05-1 RUN"(FALSE) -> ()
                            n1278 = local write "LAB05-1 (DISP)"(w2097) -> ()
                          }
                          frame #1 {
                            n1279 = TDMS Close(11:w2098) -> (0:w2099:errorcluster)  [unwired: 1 in, 1 out]
                            n1280 = local write "data file error"(w2099) -> ()
                          }
                          frame #2 {
                            n1281 = call "Save data file to network drive v1.vi"("panel id"="LAB05-1") -> ("network file save error"=w2100:errorcluster)  [unwired: 9 in, 1 out]
                            n1282 = local write "data file error"(w2100) -> ()
                          }
                        }
                      }
                    }
                  }
                }
              }
              frame #9 {
                # "LAB05-2"
                n1283 = case shown="True" w2102 {
                  frame False {
                  }
                  frame True {
                    n1284 = local read "LAB05-2 (DISP)"() -> (w2104:T4)
                    n1285 = local read "LAB05-2 (TDMS)"() -> (w2103:refnum<k34>)
                    n1286 = Unbundle(w2104) -> ("STATUS"=w2105:string)  [unwired: 2 out]
                    n1287 = Not Equal?(x=w2105, y="RUN") -> (x != y?=w2106:bool)
                    n1288 = case shown="True" w2106 {
                      tunnel: w2104 -> [_ w2109]
                      tunnel: w2103 -> [_ w2108]
                      frame False {
                      }
                      frame True {
                        n1289 = stacked-sequence {
                          tunnel: w2109 -> [w2111 _ _]
                          tunnel: w2108 -> [_ w2113 _]
                          frame #0 {
                            (unwired) "END"
                            n1290 = Bundle(cluster=w2111) -> (w2112:T4)  [unwired: 3 in]
                            n1291 = local write "LAB05-2 RUN"(FALSE) -> ()
                            n1292 = local write "LAB05-2 (DISP)"(w2112) -> ()
                          }
                          frame #1 {
                            n1293 = TDMS Close(11:w2113) -> (0:w2114:errorcluster)  [unwired: 1 in, 1 out]
                            n1294 = local write "data file error"(w2114) -> ()
                          }
                          frame #2 {
                            n1295 = call "Save data file to network drive v1.vi"("panel id"="LAB05-2") -> ("network file save error"=w2115:errorcluster)  [unwired: 9 in, 1 out]
                            n1296 = local write "data file error"(w2115) -> ()
                          }
                        }
                      }
                    }
                  }
                }
              }
            }
            n1297 = local read "Network Directory"() -> (w1956:path)
            n1298 = global write "Global 1.vi" "Network Drive"(w1956) -> ()
          }
          frame #8 {
            # "drive jigs"
            n1299 = stacked-sequence {
              frame #0 {
                # "jig on"
                n1300 = local read "jig cycle"() -> (w2117:dbl)
                n1301 = Equal?(x=w2117, y=0) -> (x = y?=w2119:bool)
                n1302 = case shown="True" w2119 {
                  frame False {
                  }
                  frame True {
                    n1303 = local read "LAB01-1RUN"() -> (w2120:bool)
                    n1304 = local read "LAB01-2 RUN"() -> (w2121:bool)
                    n1305 = local read "LAB03-1 RUN"() -> (w2127:bool)
                    n1306 = local read "LAB03-2 RUN"() -> (w2126:bool)
                    n1307 = local read "LAB02-1 RUN"() -> (w2129:bool)
                    n1308 = local read "LAB02-2 RUN"() -> (w2128:bool)
                    n1309 = local read "LAB04-1 RUN"() -> (w2125:bool)
                    n1310 = local read "LAB04-2 RUN"() -> (w2124:bool)
                    n1311 = local read "LAB05-1 RUN"() -> (w2123:bool)
                    n1312 = local read "LAB05-2 RUN"() -> (w2122:bool)
                    n1313 = local write "LAB05-1 (JIG)"(w2123) -> ()
                    n1314 = local write "LAB05-2 (JIG)"(w2122) -> ()
                    n1315 = local write "LAB04-2 (JIG)"(w2124) -> ()
                    n1316 = local write "LAB02-1 (JIG)"(w2129) -> ()
                    n1317 = local write "LAB03-1 (JIG)"(w2127) -> ()
                    n1318 = local write "LAB04-1 (JIG)"(w2125) -> ()
                    n1319 = local write "LAB03-2 (JIG)"(w2126) -> ()
                    n1320 = local write "LAB02-2 (JIG)"(w2128) -> ()
                    n1321 = local write "LAB01-1 (JIG)"(w2120) -> ()
                    n1322 = local write "LAB01-2 (JIG)"(w2121) -> ()
                  }
                }
              }
              frame #1 {
                # "jig off"
                n1323 = local read "jig cycle"() -> (w2132:dbl)
                n1324 = local read "on loops"() -> (w2131:dbl)
                n1325 = Equal?(x=w2132, y=w2131) -> (x = y?=w2130:bool)
                n1326 = case shown="True" w2130 {
                  frame False {
                  }
                  frame True {
                    w2183 = FALSE
                    w2184 = TRUE
                    w2182 = 2
                    n1327 = local read "LAB05-2 SELECT"() -> (w2173:T3)
                    n1328 = local read "LAB04-2 SELECT"() -> (w2175:T3)
                    n1329 = local read "LAB04-1 SELECT"() -> (w2176:T3)
                    n1330 = local read "LAB05-1 SELECT"() -> (w2174:T3)
                    n1331 = local read "LAB03-2 SELECT"() -> (w2177:T3)
                    n1332 = local read "LAB02-1 SELECT"() -> (w2180:T3)
                    n1333 = local read "LAB03-1 SELECT"() -> (w2178:T3)
                    n1334 = local read "LAB02-2 SELECT"() -> (w2179:T3)
                    n1335 = local read "LAB01-2 SELECT"() -> (w2181:T3)
                    n1336 = local read "LAB05-1 RUN"() -> (w2143:bool)
                    n1337 = local read "LAB05-2 RUN"() -> (w2142:bool)
                    n1338 = local read "LAB04-2 RUN"() -> (w2144:bool)
                    n1339 = local read "LAB04-1 RUN"() -> (w2145:bool)
                    n1340 = local read "LAB01-2 RUN"() -> (w2150:bool)
                    n1341 = local read "LAB03-2 RUN"() -> (w2146:bool)
                    n1342 = local read "LAB01-1RUN"() -> (w2161:bool)
                    n1343 = local read "LAB01-1 SELECT"() -> (w2185:T3)
                    n1344 = local read "LAB03-1 RUN"() -> (w2147:bool)
                    n1345 = local read "LAB02-1 RUN"() -> (w2149:bool)
                    n1346 = local read "LAB02-2 RUN"() -> (w2148:bool)
                    n1347 = Equal?(x=w2182, y=w2178) -> (x = y?=w2156:bool)
                    n1348 = Equal?(x=w2182, y=w2177) -> (x = y?=w2155:bool)
                    n1349 = Equal?(x=w2182, y=w2176) -> (x = y?=w2154:bool)
                    n1350 = Equal?(x=w2182, y=w2175) -> (x = y?=w2153:bool)
                    n1351 = Equal?(x=w2182, y=w2174) -> (x = y?=w2152:bool)
                    n1352 = Equal?(x=w2182, y=w2173) -> (x = y?=w2151:bool)
                    n1353 = Equal?(x=w2182, y=w2185) -> (x = y?=w2162:bool)
                    n1354 = Equal?(x=w2182, y=w2180) -> (x = y?=w2158:bool)
                    n1355 = Equal?(x=w2182, y=w2179) -> (x = y?=w2157:bool)
                    n1356 = Equal?(x=w2182, y=w2181) -> (x = y?=w2159:bool)
                    n1357 = And(x=w2153, y=w2144) -> (x .and. y?=w2135:bool)
                    n1358 = And(x=w2156, y=w2147) -> (x .and. y?=w2138:bool)
                    n1359 = And(x=w2154, y=w2145) -> (x .and. y?=w2136:bool)
                    n1360 = And(x=w2151, y=w2142) -> (x .and. y?=w2133:bool)
                    n1361 = And(x=w2157, y=w2148) -> (x .and. y?=w2139:bool)
                    n1362 = And(x=w2155, y=w2146) -> (x .and. y?=w2137:bool)
                    n1363 = And(x=w2152, y=w2143) -> (x .and. y?=w2134:bool)
                    n1364 = And(x=w2159, y=w2150) -> (x .and. y?=w2141:bool)
                    n1365 = And(x=w2162, y=w2161) -> (x .and. y?=w2160:bool)
                    n1366 = And(x=w2158, y=w2149) -> (x .and. y?=w2140:bool)
                    n1367 = Select(t=w2184, s=w2160, f=w2183) -> (s? t:f=w2163:bool)
                    n1368 = Select(t=w2184, s=w2141, f=w2183) -> (s? t:f=w2164:bool)
                    n1369 = Select(t=w2184, s=w2140, f=w2183) -> (s? t:f=w2165:bool)
                    n1370 = Select(t=w2184, s=w2139, f=w2183) -> (s? t:f=w2166:bool)
                    n1371 = Select(t=w2184, s=w2138, f=w2183) -> (s? t:f=w2167:bool)
                    n1372 = Select(t=w2184, s=w2137, f=w2183) -> (s? t:f=w2168:bool)
                    n1373 = Select(t=w2184, s=w2136, f=w2183) -> (s? t:f=w2169:bool)
                    n1374 = Select(t=w2184, s=w2135, f=w2183) -> (s? t:f=w2170:bool)
                    n1375 = Select(t=w2184, s=w2134, f=w2183) -> (s? t:f=w2171:bool)
                    n1376 = Select(t=w2184, s=w2133, f=w2183) -> (s? t:f=w2172:bool)
                    n1377 = local write "LAB03-2 (JIG)"(w2168) -> ()
                    n1378 = local write "LAB02-1 (JIG)"(w2165) -> ()
                    n1379 = local write "LAB02-2 (JIG)"(w2166) -> ()
                    n1380 = local write "LAB01-2 (JIG)"(w2164) -> ()
                    n1381 = local write "LAB03-1 (JIG)"(w2167) -> ()
                    n1382 = local write "LAB01-1 (JIG)"(w2163) -> ()
                    n1383 = local write "LAB05-2 (JIG)"(w2172) -> ()
                    n1384 = local write "LAB04-1 (JIG)"(w2169) -> ()
                    n1385 = local write "LAB05-1 (JIG)"(w2171) -> ()
                    n1386 = local write "LAB04-2 (JIG)"(w2170) -> ()
                  }
                }
              }
            }
          }
          frame #9 {
            # "drive digital output"
            n1387 = local read "LAB05-2 (O/I)"() -> (w2191:bool)
            n1388 = local read "LAB05-2 (JIG)"() -> (w2190:bool)
            n1389 = local read "LAB05-1 (O/I)"() -> (w2193:bool)
            n1390 = local read "LAB05-1 (JIG)"() -> (w2192:bool)
            n1391 = local read "LAB04-2 (O/I)"() -> (w2195:bool)
            n1392 = local read "LAB04-2 (JIG)"() -> (w2194:bool)
            n1393 = local read "LAB03-1 (O/I)"() -> (w2200:bool)
            n1394 = local read "LAB04-1 (O/I)"() -> (w2196:bool)
            n1395 = local read "LAB04-1 (JIG)"() -> (w2189:bool)
            n1396 = local read "LAB02-1 (O/I)"() -> (w2204:bool)
            n1397 = local read "LAB02-2 (O/I)"() -> (w2202:bool)
            n1398 = local read "LAB03-2 (O/I)"() -> (w2198:bool)
            n1399 = local read "LAB03-2 (JIG)"() -> (w2197:bool)
            n1400 = local read "LAB02-1 (JIG)"() -> (w2203:bool)
            n1401 = local read "LAB02-2 (JIG)"() -> (w2201:bool)
            n1402 = local read "LAB03-1 (JIG)"() -> (w2199:bool)
            n1403 = local read "LAB01-2 (O/I)"() -> (w2206:bool)
            n1404 = local read "LAB01-2 (JIG)"() -> (w2205:bool)
            n1405 = local read "LAB01-1 (O/I)"() -> (w2208:bool)
            n1406 = local read "LAB01-1 (JIG)"() -> (w2207:bool)
            n1407 = Build Array(w2195, w2194, w2193, w2192, w2191, w2190) -> (w2186:bool[])
            n1408 = Build Array(w2201, w2200, w2199, w2198, w2197, w2196, w2189) -> (w2187:bool[])
            n1409 = Build Array(w2208, w2207, w2206, w2205, w2204, w2203, w2202) -> (w2188:bool[])
            n1410 = call "sub vi - Drive Relays All v6.vi"("Array #2"=w2186, "Array #1"=w2187, "Array #0"=w2188) -> ()  [unwired: 8 in, 1 out]
          }
          frame #10 {
            # "get temperature values"
            n1411 = stacked-sequence {
              frame #0 {
                n1412 = local read "jig cycle"() -> (w2209:dbl)
                n1413 = local read "on loops"() -> (w2212:dbl)
                n1414 = local read "jig cycle"() -> (w2214:dbl)
                n1415 = Add(x=w2212, y=2) -> (x+y=w2213:dbl)
                n1416 = Equal?(x=w2214, y=0) -> (x = y?=w2215:bool)
                n1417 = Equal?(x=w2209, y=w2213) -> (x = y?=w2210:bool)
                n1418 = case shown="True" w2215 {
                  frame False {
                  }
                  frame True {
                    w2227 = FALSE
                    w2228 = TRUE
                    n1419 = local write "TEMP update"(TRUE) -> ()
                    n1420 = call "sub vi - GET ALL TEMP v3.vi"("LA01-EN"=w2228, "LA02-EN"=w2228, "LA03-EN"=w2228, "LA04-EN"=w2227, "LA05-EN"=w2227, "Gen Cal Value"=1.0) -> ("LA01 TEMP"=w2226:T17, "LA02 TEMP"=w2224:T17, "LA03 TEMP"=w2223:T17)  [unwired: 4 in, 3 out]
                    n1421 = local write "LAB03 TEMP"(w2223) -> ()
                    n1422 = local write "LAB02 TEMP"(w2224) -> ()
                    n1423 = local write "LAB01 TEMP"(w2226) -> ()
                  }
                }
                n1424 = case shown="True" w2210 {
                  frame False {
                  }
                  frame True {
                    w2220 = TRUE
                    w2221 = FALSE
                    n1425 = local write "TEMP update"(TRUE) -> ()
                    n1426 = call "sub vi - GET ALL TEMP v3.vi"("LA01-EN"=w2221, "LA02-EN"=w2221, "LA03-EN"=w2221, "LA04-EN"=w2220, "LA05-EN"=w2220, "Gen Cal Value"=1.0) -> ("LA04 TEMP"=w2218:T17, "LA05 TEMP"=w2217:T17)  [unwired: 4 in, 4 out]
                    n1427 = local write "LAB04 TEMP"(w2218) -> ()
                    n1428 = local write "LAB05 TEMP"(w2217) -> ()
                  }
                }
              }
              frame #1 {
                n1429 = local read "LAB01 (CAL)"() -> (w2246:T6)
                n1430 = local read "LAB01 TEMP"() -> (w2247:T9)
                n1431 = Unbundle By Name(w2247) -> ("T1 Live"=w2237:dbl, "T1 Neut"=w2236:dbl, "T2 Live"=w2235:dbl, "T2 Neut"=w2234:dbl)  [unwired: 2 out]
                n1432 = Unbundle By Name(w2246) -> ("1 (TL) cal"=w2233:dbl, "1 (TN) cal"=w2232:dbl, "2 (TL) cal"=w2231:dbl, "2 (TN) cal"=w2230:dbl)  [unwired: 6 out]
                n1433 = Multiply(x=w2237, y=w2233) -> (x*y=w2243:dbl)
                n1434 = Multiply(x=w2236, y=w2232) -> (x*y=w2242:dbl)
                n1435 = Multiply(x=w2235, y=w2231) -> (x*y=w2239:dbl)
                n1436 = Multiply(x=w2234, y=w2230) -> (x*y=w2238:dbl)
                n1437 = local read "LAB01-2 (SIG)"() -> (w2241:T2)
                n1438 = local read "LAB01-1 (SIG)"() -> (w2245:T2)
                n1439 = Bundle By Name(cluster=w2245, "Tmp Live"=w2243, "Tmp Neut"=w2242) -> (w2244:T2)
                n1440 = Bundle By Name(cluster=w2241, "Tmp Live"=w2239, "Tmp Neut"=w2238) -> (w2240:T2)
                n1441 = local write "LAB01-1 (SIG)"(w2244) -> ()
                n1442 = local write "LAB01-2 (SIG)"(w2240) -> ()
              }
              frame #2 {
                n1443 = local read "LAB02 (CAL)"() -> (w2264:T7)
                n1444 = local read "LAB02 TEMP"() -> (w2265:T9)
                n1445 = Unbundle By Name(w2265) -> ("T1 Live"=w2255:dbl, "T1 Neut"=w2254:dbl, "T2 Live"=w2253:dbl, "T2 Neut"=w2252:dbl)  [unwired: 2 out]
                n1446 = Unbundle By Name(w2264) -> ("1 (TL) cal"=w2251:dbl, "1 (TN) cal"=w2250:dbl, "2 (TL) cal"=w2249:dbl, "2 (TN) cal"=w2248:dbl)  [unwired: 6 out]
                n1447 = Multiply(x=w2255, y=w2251) -> (x*y=w2261:dbl)
                n1448 = Multiply(x=w2254, y=w2250) -> (x*y=w2260:dbl)
                n1449 = Multiply(x=w2253, y=w2249) -> (x*y=w2257:dbl)
                n1450 = Multiply(x=w2252, y=w2248) -> (x*y=w2256:dbl)
                n1451 = local read "LAB02-2 (SIG)"() -> (w2259:T2)
                n1452 = local read "LAB02-1 (SIG)"() -> (w2263:T2)
                n1453 = Bundle By Name(cluster=w2263, "Tmp Live"=w2261, "Tmp Neut"=w2260) -> (w2262:T2)
                n1454 = Bundle By Name(cluster=w2259, "Tmp Live"=w2257, "Tmp Neut"=w2256) -> (w2258:T2)
                n1455 = local write "LAB02-1 (SIG)"(w2262) -> ()
                n1456 = local write "LAB02-2 (SIG)"(w2258) -> ()
              }
              frame #3 {
                n1457 = local read "LAB03 (CAL)"() -> (w2282:T6)
                n1458 = local read "LAB03 TEMP"() -> (w2283:T9)
                n1459 = Unbundle By Name(w2283) -> ("T1 Live"=w2273:dbl, "T1 Neut"=w2272:dbl, "T2 Live"=w2271:dbl, "T2 Neut"=w2270:dbl)  [unwired: 2 out]
                n1460 = Unbundle By Name(w2282) -> ("1 (TL) cal"=w2269:dbl, "1 (TN) cal"=w2268:dbl, "2 (TL) cal"=w2267:dbl, "2 (TN) cal"=w2266:dbl)  [unwired: 6 out]
                n1461 = Multiply(x=w2273, y=w2269) -> (x*y=w2279:dbl)
                n1462 = Multiply(x=w2272, y=w2268) -> (x*y=w2278:dbl)
                n1463 = Multiply(x=w2271, y=w2267) -> (x*y=w2275:dbl)
                n1464 = Multiply(x=w2270, y=w2266) -> (x*y=w2274:dbl)
                n1465 = local read "LAB03-2 (SIG)"() -> (w2277:T2)
                n1466 = local read "LAB03-1 (SIG)"() -> (w2281:T2)
                n1467 = Bundle By Name(cluster=w2281, "Tmp Live"=w2279, "Tmp Neut"=w2278) -> (w2280:T2)
                n1468 = Bundle By Name(cluster=w2277, "Tmp Live"=w2275, "Tmp Neut"=w2274) -> (w2276:T2)
                n1469 = local write "LAB03-1 (SIG)"(w2280) -> ()
                n1470 = local write "LAB03-2 (SIG)"(w2276) -> ()
              }
              frame #4 {
                n1471 = local read "LAB04 (CAL)"() -> (w2300:T6)
                n1472 = local read "LAB04 TEMP"() -> (w2301:T9)
                n1473 = Unbundle By Name(w2301) -> ("T1 Live"=w2291:dbl, "T1 Neut"=w2290:dbl, "T2 Live"=w2289:dbl, "T2 Neut"=w2288:dbl)  [unwired: 2 out]
                n1474 = Unbundle By Name(w2300) -> ("1 (TL) cal"=w2287:dbl, "1 (TN) cal"=w2286:dbl, "2 (TL) cal"=w2285:dbl, "2 (TN) cal"=w2284:dbl)  [unwired: 6 out]
                n1475 = Multiply(x=w2291, y=w2287) -> (x*y=w2297:dbl)
                n1476 = Multiply(x=w2290, y=w2286) -> (x*y=w2296:dbl)
                n1477 = Multiply(x=w2289, y=w2285) -> (x*y=w2293:dbl)
                n1478 = Multiply(x=w2288, y=w2284) -> (x*y=w2292:dbl)
                n1479 = local read "LAB04-2 (SIG)"() -> (w2295:T2)
                n1480 = local read "LAB04-1 (SIG)"() -> (w2299:T2)
                n1481 = Bundle By Name(cluster=w2299, "Tmp Live"=w2297, "Tmp Neut"=w2296) -> (w2298:T2)
                n1482 = Bundle By Name(cluster=w2295, "Tmp Live"=w2293, "Tmp Neut"=w2292) -> (w2294:T2)
                n1483 = local write "LAB04-1 (SIG)"(w2298) -> ()
                n1484 = local write "LAB04-2 (SIG)"(w2294) -> ()
              }
              frame #5 {
                n1485 = local read "LAB05 (CAL)"() -> (w2318:T6)
                n1486 = local read "LAB05 TEMP"() -> (w2319:T9)
                n1487 = Unbundle By Name(w2319) -> ("T1 Live"=w2309:dbl, "T1 Neut"=w2308:dbl, "T2 Live"=w2307:dbl, "T2 Neut"=w2306:dbl)  [unwired: 2 out]
                n1488 = Unbundle By Name(w2318) -> ("1 (TL) cal"=w2305:dbl, "1 (TN) cal"=w2304:dbl, "2 (TL) cal"=w2303:dbl, "2 (TN) cal"=w2302:dbl)  [unwired: 6 out]
                n1489 = Multiply(x=w2309, y=w2305) -> (x*y=w2315:dbl)
                n1490 = Multiply(x=w2308, y=w2304) -> (x*y=w2314:dbl)
                n1491 = Multiply(x=w2307, y=w2303) -> (x*y=w2311:dbl)
                n1492 = Multiply(x=w2306, y=w2302) -> (x*y=w2310:dbl)
                n1493 = local read "LAB05-2 (SIG)"() -> (w2313:T2)
                n1494 = local read "LAB05-1 (SIG)"() -> (w2317:T2)
                n1495 = Bundle By Name(cluster=w2317, "Tmp Live"=w2315, "Tmp Neut"=w2314) -> (w2316:T2)
                n1496 = Bundle By Name(cluster=w2313, "Tmp Live"=w2311, "Tmp Neut"=w2310) -> (w2312:T2)
                n1497 = local write "LAB05-1 (SIG)"(w2316) -> ()
                n1498 = local write "LAB05-2 (SIG)"(w2312) -> ()
              }
            }
          }
          frame #11 {
            # "get analog values"
            n1499 = local read "on loops"() -> (w2326:dbl)
            n1500 = local read "jig cycle"() -> (w2323:dbl)
            n1501 = Add(x=w2326, y=1) -> (x+y=w2324:dbl)
            n1502 = Equal?(x=w2323, y=1) -> (x = y?=w2321:bool)
            n1503 = Equal?(x=w2323, y=w2324) -> (x = y?=w2322:bool)
            n1504 = Or(x=w2321, y=w2322) -> (x .or. y?=w2320:bool)
            n1505 = case shown="True" w2320 {
              frame False {
              }
              frame True {
                n1506 = call "sub vi - Read Analog All v8.vi"() -> ("Analog loop time"=w2334:dbl, "array GRAPH"=w2333:dynamicdata[], "LAB01"=w2332:T18, "LAB02"=w2331:T19, "LAB03"=w2330:T20, "LAB04"=w2329:T21, "array ERROR"=w2335:errorcluster[], "LAB05"=w2328:T22)  [unwired: 8 in]
                n1507 = stacked-sequence {
                  tunnel: w2335 -> [w2338 _ _ _ _ _]
                  tunnel: w2334 -> [w2337 _ _ _ _ _]
                  tunnel: w2333 -> [w2336 _ _ _ _ _]
                  tunnel: w2332 -> [_ w2383 _ _ _ _]
                  tunnel: w2331 -> [_ _ w2384 _ _ _]
                  tunnel: w2330 -> [_ _ _ w2409 _ _]
                  tunnel: w2329 -> [_ _ _ _ w2432 _]
                  tunnel: w2328 -> [_ _ _ _ _ w2457]
                  frame #0 {
                    n1508 = local write "AI update"(TRUE) -> ()
                    n1509 = Index Array(array=w2336, index=6) -> (element=→"LAB04-1 (GRAPH)":dynamicdata)
                    n1510 = Index Array(array=w2336, index=7) -> (element=→"LAB04-2 (GRAPH)":dynamicdata)
                    n1511 = Index Array(array=w2336, index=9) -> (element=→"LAB05-2 (GRAPH)":dynamicdata)
                    n1512 = Index Array(array=w2336, index=8) -> (element=→"LAB05-1 (GRAPH)":dynamicdata)
                    n1513 = Index Array(array=w2336, index=5) -> (element=→"LAB03-2 (GRAPH)":dynamicdata)
                    n1514 = Index Array(array=w2336, index=0) -> (element=→"LAB01-1 (GRAPH)":dynamicdata)
                    n1515 = Index Array(array=w2336, index=1) -> (element=→"LAB01-2 (GRAPH)":dynamicdata)
                    n1516 = Index Array(array=w2336, index=2) -> (element=→"LAB02-1 (GRAPH)":dynamicdata)
                    n1517 = Index Array(array=w2336, index=3) -> (element=→"LAB02-2 (GRAPH)":dynamicdata)
                    n1518 = Index Array(array=w2336, index=4) -> (element=→"LAB03-1 (GRAPH)":dynamicdata)
                    "AI loop time" <- w2337
                    "Analog Error Array" <- w2338
                  }
                  frame #1 {
                    n1519 = local read "LAB01 (CAL)"() -> (w2382:T6)
                    n1520 = Unbundle By Name(w2383) -> ("LAB01-1 (A)"=w2381:dbl, "LAB01-1 (V)"=w2380:dbl, "LAB01-1 (PF)"=w2379:dbl, "LAB01-2 (A)"=w2378:dbl, "LAB01-2 (V)"=w2377:dbl, "LAB01-2 (PF)"=w2376:dbl)
                    n1521 = Unbundle By Name(w2382) -> ("1  (A) cal"=w2375:dbl, "1 (V) cal"=w2374:dbl, "1 (PF) cal"=w2373:dbl, "2 (A) cal"=w2372:dbl, "2 (V) cal"=w2371:dbl, "2 (PF) cal"=w2370:dbl)  [unwired: 4 out]
                    n1522 = Multiply(x=w2381, y=w2375) -> (x*y=w2368:dbl)
                    n1523 = Multiply(x=w2380, y=w2374) -> (x*y=w2367:dbl)
                    n1524 = Multiply(x=w2379, y=w2373) -> (x*y=w2366:dbl)
                    n1525 = Multiply(x=w2378, y=w2372) -> (x*y=w2362:dbl)
                    n1526 = local read "LAB01-1 (SIG)"() -> (w2369:T2)
                    n1527 = Multiply(x=w2377, y=w2371) -> (x*y=w2361:dbl)
                    n1528 = Multiply(x=w2376, y=w2370) -> (x*y=w2360:dbl)
                    n1529 = local read "LAB01-2 (SIG)"() -> (w2364:T2)
                    n1530 = Bundle By Name(cluster=w2369, "AMPS"=w2368, "VOLTS"=w2367, "PF"=w2366) -> (w2365:T2)
                    n1531 = Bundle By Name(cluster=w2364, "AMPS"=w2362, "VOLTS"=w2361, "PF"=w2360) -> (w2363:T2)
                    n1532 = local write "LAB01-2 (SIG)"(w2363) -> ()
                    n1533 = local write "LAB01-1 (SIG)"(w2365) -> ()
                  }
                  frame #2 {
                    n1534 = local read "LAB02 (CAL)"() -> (w2407:T7)
                    n1535 = Unbundle By Name(w2384) -> ("LAB02-1 (A)"=w2406:dbl, "LAB02-1 (V)"=w2405:dbl, "LAB02-1 (PF)"=w2404:dbl, "LAB02-2 (A)"=w2403:dbl, "LAB02-2 (V)"=w2402:dbl, "LAB02-2 (PF)"=w2401:dbl)
                    n1536 = Unbundle By Name(w2407) -> ("1 (A) cal"=w2400:dbl, "1 (V) cal"=w2399:dbl, "1 (PF) cal"=w2398:dbl, "2 (A) cal"=w2397:dbl, "2 (V) cal"=w2396:dbl, "2 (PF) cal"=w2395:dbl)  [unwired: 4 out]
                    n1537 = Multiply(x=w2406, y=w2400) -> (x*y=w2393:dbl)
                    n1538 = Multiply(x=w2405, y=w2399) -> (x*y=w2392:dbl)
                    n1539 = Multiply(x=w2404, y=w2398) -> (x*y=w2391:dbl)
                    n1540 = Multiply(x=w2403, y=w2397) -> (x*y=w2387:dbl)
                    n1541 = local read "LAB02-1 (SIG)"() -> (w2394:T2)
                    n1542 = Multiply(x=w2402, y=w2396) -> (x*y=w2386:dbl)
                    n1543 = Multiply(x=w2401, y=w2395) -> (x*y=w2385:dbl)
                    n1544 = local read "LAB02-2 (SIG)"() -> (w2389:T2)
                    n1545 = Bundle By Name(cluster=w2394, "AMPS"=w2393, "VOLTS"=w2392, "PF"=w2391) -> (w2390:T2)
                    n1546 = Bundle By Name(cluster=w2389, "AMPS"=w2387, "VOLTS"=w2386, "PF"=w2385) -> (w2388:T2)
                    n1547 = local write "LAB02-2 (SIG)"(w2388) -> ()
                    n1548 = local write "LAB02-1 (SIG)"(w2390) -> ()
                  }
                  frame #3 {
                    n1549 = local read "LAB03 (CAL)"() -> (w2431:T6)
                    n1550 = Unbundle By Name(w2409) -> ("LAB03-1 (A)"=w2430:dbl, "LAB03-1 (V)"=w2429:dbl, "LAB03-1 (PF)"=w2428:dbl, "LAB03-2 (A)"=w2427:dbl, "LAB03-2 (V)"=w2426:dbl, "LAB03-2 (PF)"=w2425:dbl)
                    n1551 = Unbundle By Name(w2431) -> ("1  (A) cal"=w2424:dbl, "1 (V) cal"=w2423:dbl, "1 (PF) cal"=w2422:dbl, "2 (A) cal"=w2421:dbl, "2 (V) cal"=w2420:dbl, "2 (PF) cal"=w2419:dbl)  [unwired: 4 out]
                    n1552 = Multiply(x=w2430, y=w2424) -> (x*y=w2417:dbl)
                    n1553 = Multiply(x=w2429, y=w2423) -> (x*y=w2408:dbl)
                    n1554 = Multiply(x=w2428, y=w2422) -> (x*y=w2416:dbl)
                    n1555 = Multiply(x=w2427, y=w2421) -> (x*y=w2412:dbl)
                    n1556 = local read "LAB03-1 (SIG)"() -> (w2418:T2)
                    n1557 = Multiply(x=w2426, y=w2420) -> (x*y=w2411:dbl)
                    n1558 = Multiply(x=w2425, y=w2419) -> (x*y=w2410:dbl)
                    n1559 = local read "LAB03-2 (SIG)"() -> (w2414:T2)
                    n1560 = Bundle By Name(cluster=w2418, "AMPS"=w2417, "VOLTS"=w2408, "PF"=w2416) -> (w2415:T2)
                    n1561 = Bundle By Name(cluster=w2414, "AMPS"=w2412, "VOLTS"=w2411, "PF"=w2410) -> (w2413:T2)
                    n1562 = local write "LAB03-2 (SIG)"(w2413) -> ()
                    n1563 = local write "LAB03-1 (SIG)"(w2415) -> ()
                  }
                  frame #4 {
                    n1564 = local read "LAB04 (CAL)"() -> (w2455:T6)
                    n1565 = Unbundle By Name(w2432) -> ("LAB04-1 (A)"=w2454:dbl, "LAB04-1 (V)"=w2453:dbl, "LAB04-1 (PF)"=w2452:dbl, "LAB04-2 (A)"=w2451:dbl, "LAB04-2 (V)"=w2450:dbl, "LAB04-2 (PF)"=w2449:dbl)
                    n1566 = Unbundle By Name(w2455) -> ("1  (A) cal"=w2448:dbl, "1 (V) cal"=w2447:dbl, "1 (PF) cal"=w2446:dbl, "2 (A) cal"=w2445:dbl, "2 (V) cal"=w2444:dbl, "2 (PF) cal"=w2443:dbl)  [unwired: 4 out]
                    n1567 = Multiply(x=w2454, y=w2448) -> (x*y=w2441:dbl)
                    n1568 = Multiply(x=w2453, y=w2447) -> (x*y=w2440:dbl)
                    n1569 = Multiply(x=w2452, y=w2446) -> (x*y=w2439:dbl)
                    n1570 = Multiply(x=w2451, y=w2445) -> (x*y=w2435:dbl)
                    n1571 = local read "LAB04-1 (SIG)"() -> (w2442:T2)
                    n1572 = Multiply(x=w2450, y=w2444) -> (x*y=w2434:dbl)
                    n1573 = Multiply(x=w2449, y=w2443) -> (x*y=w2433:dbl)
                    n1574 = local read "LAB04-2 (SIG)"() -> (w2437:T2)
                    n1575 = Bundle By Name(cluster=w2442, "AMPS"=w2441, "VOLTS"=w2440, "PF"=w2439) -> (w2438:T2)
                    n1576 = Bundle By Name(cluster=w2437, "AMPS"=w2435, "VOLTS"=w2434, "PF"=w2433) -> (w2436:T2)
                    n1577 = local write "LAB04-2 (SIG)"(w2436) -> ()
                    n1578 = local write "LAB04-1 (SIG)"(w2438) -> ()
                  }
                  frame #5 {
                    n1579 = local read "LAB05 (CAL)"() -> (w2479:T6)
                    n1580 = Unbundle By Name(w2457) -> ("LAB05-1 (A)"=w2478:dbl, "LAB05-1 (V)"=w2456:dbl, "LAB05-1 (PF)"=w2477:dbl, "LAB05-2 (A)"=w2476:dbl, "LAB05-2 (V)"=w2475:dbl, "LAB05-2 (PF)"=w2474:dbl)
                    n1581 = Unbundle By Name(w2479) -> ("1  (A) cal"=w2473:dbl, "1 (V) cal"=w2472:dbl, "1 (PF) cal"=w2471:dbl, "2 (A) cal"=w2470:dbl, "2 (V) cal"=w2469:dbl, "2 (PF) cal"=w2468:dbl)  [unwired: 4 out]
                    n1582 = Multiply(x=w2478, y=w2473) -> (x*y=w2466:dbl)
                    n1583 = Multiply(x=w2456, y=w2472) -> (x*y=w2465:dbl)
                    n1584 = Multiply(x=w2477, y=w2471) -> (x*y=w2464:dbl)
                    n1585 = Multiply(x=w2476, y=w2470) -> (x*y=w2460:dbl)
                    n1586 = local read "LAB05-1 (SIG)"() -> (w2467:T2)
                    n1587 = Multiply(x=w2475, y=w2469) -> (x*y=w2459:dbl)
                    n1588 = Multiply(x=w2474, y=w2468) -> (x*y=w2458:dbl)
                    n1589 = local read "LAB05-2 (SIG)"() -> (w2462:T2)
                    n1590 = Bundle By Name(cluster=w2467, "AMPS"=w2466, "VOLTS"=w2465, "PF"=w2464) -> (w2463:T2)
                    n1591 = Bundle By Name(cluster=w2462, "AMPS"=w2460, "VOLTS"=w2459, "PF"=w2458) -> (w2461:T2)
                    n1592 = local write "LAB05-2 (SIG)"(w2461) -> ()
                    n1593 = local write "LAB05-1 (SIG)"(w2463) -> ()
                  }
                }
              }
            }
          }
          frame #12 {
            # "save test data to file"
            n1594 = local read "on loops"() -> (w2496:dbl)
            n1595 = local read "jig cycle"() -> (w2493:dbl)
            n1596 = Add(x=w2496, y=2) -> (x+y=w2494:dbl)
            n1597 = Equal?(x=w2493, y=1) -> (x = y?=w2491:bool)
            n1598 = Equal?(x=w2493, y=w2494) -> (x = y?=w2492:bool)
            n1599 = Or(x=w2491, y=w2492) -> (x .or. y?=w2490:bool)
            n1600 = case shown="True" w2490 {
              tunnel: w2489 -> [_ w2507]
              tunnel: w2488 -> [_ w2506]
              tunnel: w2487 -> [_ w2505]
              tunnel: w2486 -> [_ w2504]
              tunnel: w2485 -> [_ w2503]
              tunnel: w2484 -> [_ w2502]
              tunnel: w2483 -> [_ w2501]
              tunnel: w2482 -> [_ w2500]
              tunnel: w2481 -> [_ w2499]
              tunnel: w2480 -> [_ w2498]
              frame False {
              }
              frame True {
                n1601 = stacked-sequence {
                  tunnel: w2507 -> [w2508 _ _ _ _ _ _ _ _ _]
                  tunnel: w2506 -> [_ w2553 _ _ _ _ _ _ _ _]
                  tunnel: w2505 -> [_ _ w2598 _ _ _ _ _ _ _]
                  tunnel: w2504 -> [_ _ _ w2643 _ _ _ _ _ _]
                  tunnel: w2503 -> [_ _ _ _ w2688 _ _ _ _ _]
                  tunnel: w2502 -> [_ _ _ _ _ w2733 _ _ _ _]
                  tunnel: w2501 -> [_ _ _ _ _ _ w2778 _ _ _]
                  tunnel: w2500 -> [_ _ _ _ _ _ _ w2823 _ _]
                  tunnel: w2499 -> [_ _ _ _ _ _ _ _ w2868 _]
                  tunnel: w2498 -> [_ _ _ _ _ _ _ _ _ w2913]
                  frame #0 {
                    # "LAB01-1"
                    n1602 = case shown="True" w2508 {
                      frame False {
                      }
                      frame True {
                        n1603 = local read "LAB01-1 (DISP)"() -> (w2550:T4)
                        n1604 = local read "LAB01-1 (SIG)"() -> (w2551:T2)
                        n1605 = local read "LAB01-1 (TDMS)"() -> (w2552:refnum<k34>)
                        n1606 = Build Array("TEMP Neut") -> (w2516:string[])
                        n1607 = Build Array("CYCLE") -> (w2511:string[])
                        n1608 = Build Array("TEMP Live") -> (w2521:string[])
                        n1609 = Build Array("PF") -> (w2526:string[])
                        n1610 = Build Array("AMPS") -> (w2547:string[])
                        n1611 = Build Array("VOLTS") -> (w2538:string[])
                        n1612 = Unbundle(w2551) -> ("AMPS"=w2546:dbl, "VOLTS"=w2535:dbl, "PF"=w2534:dbl, "Tmp Live"=w2533:dbl, "Tmp Neut"=w2536:dbl)
                        n1613 = Unbundle(w2550) -> ("CYCLE"=w2531:dbl)  [unwired: 2 out]
                        n1614 = Build Array(w2535) -> (w2532:dbl[])
                        n1615 = Build Array(w2534) -> (w2525:dbl[])
                        n1616 = Build Array(w2533) -> (w2520:dbl[])
                        n1617 = Build Array(w2536) -> (w2515:dbl[])
                        n1618 = Build Array(w2546) -> (w2545:dbl[])
                        n1619 = Build Array(w2531) -> (w2510:dbl[])
                        n1620 = TDMS Write(0:w2552, 5:"LAB01-1 TEST VALUES", 7:w2547, 9:w2545) -> (4:w2540:refnum<k34>, 6:w2539:string, 15:w2527:errorcluster)  [unwired: 2 in, 1 out]
                        n1621 = TDMS Write(0:w2540, 5:w2539, 7:w2538, 9:w2532, 11:w2527) -> (4:w2530:refnum<k34>, 6:w2529:string, 15:w2528:errorcluster)  [unwired: 1 in, 1 out]
                        n1622 = TDMS Write(0:w2530, 5:w2529, 7:w2526, 9:w2525, 11:w2528) -> (4:w2524:refnum<k34>, 6:w2523:string, 15:w2522:errorcluster)  [unwired: 1 in, 1 out]
                        n1623 = TDMS Write(0:w2524, 5:w2523, 7:w2521, 9:w2520, 11:w2522) -> (4:w2519:refnum<k34>, 6:w2518:string, 15:w2517:errorcluster)  [unwired: 1 in, 1 out]
                        n1624 = TDMS Write(0:w2519, 5:w2518, 7:w2516, 9:w2515, 11:w2517) -> (4:w2514:refnum<k34>, 6:w2513:string, 15:w2512:errorcluster)  [unwired: 1 in, 1 out]
                        n1625 = TDMS Write(0:w2514, 5:w2513, 7:w2511, 9:w2510, 11:w2512) -> (15:w2509:errorcluster)  [unwired: 1 in, 3 out]
                        n1626 = local write "data file error"(w2509) -> ()
                      }
                    }
                  }
                  frame #1 {
                    # "LAB01-2"
                    n1627 = case shown="True" w2553 {
                      frame False {
                      }
                      frame True {
                        n1628 = local read "LAB01-2 (DISP)"() -> (w2595:T4)
                        n1629 = local read "LAB01-2 (SIG)"() -> (w2596:T2)
                        n1630 = local read "LAB01-2 (TDMS)"() -> (w2597:refnum<k34>)
                        n1631 = Build Array("TEMP Neut") -> (w2561:string[])
                        n1632 = Build Array("CYCLE") -> (w2556:string[])
                        n1633 = Build Array("TEMP Live") -> (w2566:string[])
                        n1634 = Build Array("PF") -> (w2571:string[])
                        n1635 = Build Array("AMPS") -> (w2592:string[])
                        n1636 = Build Array("VOLTS") -> (w2583:string[])
                        n1637 = Unbundle(w2596) -> ("AMPS"=w2591:dbl, "VOLTS"=w2580:dbl, "PF"=w2579:dbl, "Tmp Live"=w2578:dbl, "Tmp Neut"=w2581:dbl)
                        n1638 = Unbundle(w2595) -> ("CYCLE"=w2576:dbl)  [unwired: 2 out]
                        n1639 = Build Array(w2580) -> (w2577:dbl[])
                        n1640 = Build Array(w2579) -> (w2570:dbl[])
                        n1641 = Build Array(w2578) -> (w2565:dbl[])
                        n1642 = Build Array(w2581) -> (w2560:dbl[])
                        n1643 = Build Array(w2591) -> (w2590:dbl[])
                        n1644 = Build Array(w2576) -> (w2555:dbl[])
                        n1645 = TDMS Write(0:w2597, 5:"LAB01-2 TEST VALUES", 7:w2592, 9:w2590) -> (4:w2585:refnum<k34>, 6:w2584:string, 15:w2572:errorcluster)  [unwired: 2 in, 1 out]
                        n1646 = TDMS Write(0:w2585, 5:w2584, 7:w2583, 9:w2577, 11:w2572) -> (4:w2575:refnum<k34>, 6:w2574:string, 15:w2573:errorcluster)  [unwired: 1 in, 1 out]
                        n1647 = TDMS Write(0:w2575, 5:w2574, 7:w2571, 9:w2570, 11:w2573) -> (4:w2569:refnum<k34>, 6:w2568:string, 15:w2567:errorcluster)  [unwired: 1 in, 1 out]
                        n1648 = TDMS Write(0:w2569, 5:w2568, 7:w2566, 9:w2565, 11:w2567) -> (4:w2564:refnum<k34>, 6:w2563:string, 15:w2562:errorcluster)  [unwired: 1 in, 1 out]
                        n1649 = TDMS Write(0:w2564, 5:w2563, 7:w2561, 9:w2560, 11:w2562) -> (4:w2559:refnum<k34>, 6:w2558:string, 15:w2557:errorcluster)  [unwired: 1 in, 1 out]
                        n1650 = TDMS Write(0:w2559, 5:w2558, 7:w2556, 9:w2555, 11:w2557) -> (15:w2554:errorcluster)  [unwired: 1 in, 3 out]
                        n1651 = local write "data file error"(w2554) -> ()
                      }
                    }
                  }
                  frame #2 {
                    # "LAB02-1"
                    n1652 = case shown="True" w2598 {
                      frame False {
                      }
                      frame True {
                        n1653 = local read "LAB02-1 (DISP)"() -> (w2640:T4)
                        n1654 = local read "LAB02-1 (SIG)"() -> (w2641:T2)
                        n1655 = local read "LAB02-1 (TDMS)"() -> (w2642:refnum<k34>)
                        n1656 = Build Array("TEMP Neut") -> (w2606:string[])
                        n1657 = Build Array("CYCLE") -> (w2601:string[])
                        n1658 = Build Array("TEMP Live") -> (w2611:string[])
                        n1659 = Build Array("PF") -> (w2616:string[])
                        n1660 = Build Array("AMPS") -> (w2637:string[])
                        n1661 = Build Array("VOLTS") -> (w2628:string[])
                        n1662 = Unbundle(w2641) -> ("AMPS"=w2636:dbl, "VOLTS"=w2625:dbl, "PF"=w2624:dbl, "Tmp Live"=w2623:dbl, "Tmp Neut"=w2626:dbl)
                        n1663 = Unbundle(w2640) -> ("CYCLE"=w2621:dbl)  [unwired: 2 out]
                        n1664 = Build Array(w2625) -> (w2622:dbl[])
                        n1665 = Build Array(w2624) -> (w2615:dbl[])
                        n1666 = Build Array(w2623) -> (w2610:dbl[])
                        n1667 = Build Array(w2626) -> (w2605:dbl[])
                        n1668 = Build Array(w2636) -> (w2635:dbl[])
                        n1669 = Build Array(w2621) -> (w2600:dbl[])
                        n1670 = TDMS Write(0:w2642, 5:"LAB02-1 TEST VALUES", 7:w2637, 9:w2635) -> (4:w2630:refnum<k34>, 6:w2629:string, 15:w2617:errorcluster)  [unwired: 2 in, 1 out]
                        n1671 = TDMS Write(0:w2630, 5:w2629, 7:w2628, 9:w2622, 11:w2617) -> (4:w2620:refnum<k34>, 6:w2619:string, 15:w2618:errorcluster)  [unwired: 1 in, 1 out]
                        n1672 = TDMS Write(0:w2620, 5:w2619, 7:w2616, 9:w2615, 11:w2618) -> (4:w2614:refnum<k34>, 6:w2613:string, 15:w2612:errorcluster)  [unwired: 1 in, 1 out]
                        n1673 = TDMS Write(0:w2614, 5:w2613, 7:w2611, 9:w2610, 11:w2612) -> (4:w2609:refnum<k34>, 6:w2608:string, 15:w2607:errorcluster)  [unwired: 1 in, 1 out]
                        n1674 = TDMS Write(0:w2609, 5:w2608, 7:w2606, 9:w2605, 11:w2607) -> (4:w2604:refnum<k34>, 6:w2603:string, 15:w2602:errorcluster)  [unwired: 1 in, 1 out]
                        n1675 = TDMS Write(0:w2604, 5:w2603, 7:w2601, 9:w2600, 11:w2602) -> (15:w2599:errorcluster)  [unwired: 1 in, 3 out]
                        n1676 = local write "data file error"(w2599) -> ()
                      }
                    }
                  }
                  frame #3 {
                    # "LAB02-2"
                    n1677 = case shown="True" w2643 {
                      frame False {
                      }
                      frame True {
                        n1678 = local read "LAB02-2 (DISP)"() -> (w2685:T4)
                        n1679 = local read "LAB02-2 (SIG)"() -> (w2686:T2)
                        n1680 = local read "LAB02-2 (TDMS)"() -> (w2687:refnum<k34>)
                        n1681 = Build Array("TEMP Neut") -> (w2651:string[])
                        n1682 = Build Array("CYCLE") -> (w2646:string[])
                        n1683 = Build Array("TEMP Live") -> (w2656:string[])
                        n1684 = Build Array("PF") -> (w2661:string[])
                        n1685 = Build Array("AMPS") -> (w2682:string[])
                        n1686 = Build Array("VOLTS") -> (w2673:string[])
                        n1687 = Unbundle(w2686) -> ("AMPS"=w2681:dbl, "VOLTS"=w2670:dbl, "PF"=w2669:dbl, "Tmp Live"=w2668:dbl, "Tmp Neut"=w2671:dbl)
                        n1688 = Unbundle(w2685) -> ("CYCLE"=w2666:dbl)  [unwired: 2 out]
                        n1689 = Build Array(w2670) -> (w2667:dbl[])
                        n1690 = Build Array(w2669) -> (w2660:dbl[])
                        n1691 = Build Array(w2668) -> (w2655:dbl[])
                        n1692 = Build Array(w2671) -> (w2650:dbl[])
                        n1693 = Build Array(w2681) -> (w2680:dbl[])
                        n1694 = Build Array(w2666) -> (w2645:dbl[])
                        n1695 = TDMS Write(0:w2687, 5:"LAB02-2 TEST VALUES", 7:w2682, 9:w2680) -> (4:w2675:refnum<k34>, 6:w2674:string, 15:w2662:errorcluster)  [unwired: 2 in, 1 out]
                        n1696 = TDMS Write(0:w2675, 5:w2674, 7:w2673, 9:w2667, 11:w2662) -> (4:w2665:refnum<k34>, 6:w2664:string, 15:w2663:errorcluster)  [unwired: 1 in, 1 out]
                        n1697 = TDMS Write(0:w2665, 5:w2664, 7:w2661, 9:w2660, 11:w2663) -> (4:w2659:refnum<k34>, 6:w2658:string, 15:w2657:errorcluster)  [unwired: 1 in, 1 out]
                        n1698 = TDMS Write(0:w2659, 5:w2658, 7:w2656, 9:w2655, 11:w2657) -> (4:w2654:refnum<k34>, 6:w2653:string, 15:w2652:errorcluster)  [unwired: 1 in, 1 out]
                        n1699 = TDMS Write(0:w2654, 5:w2653, 7:w2651, 9:w2650, 11:w2652) -> (4:w2649:refnum<k34>, 6:w2648:string, 15:w2647:errorcluster)  [unwired: 1 in, 1 out]
                        n1700 = TDMS Write(0:w2649, 5:w2648, 7:w2646, 9:w2645, 11:w2647) -> (15:w2644:errorcluster)  [unwired: 1 in, 3 out]
                        n1701 = local write "data file error"(w2644) -> ()
                      }
                    }
                  }
                  frame #4 {
                    # "LAB03-1"
                    n1702 = case shown="True" w2688 {
                      frame False {
                      }
                      frame True {
                        n1703 = local read "LAB03-1 (DISP)"() -> (w2730:T4)
                        n1704 = local read "LAB03-1 (SIG)"() -> (w2731:T2)
                        n1705 = local read "LAB03-1 (TDMS)"() -> (w2732:refnum<k34>)
                        n1706 = Build Array("TEMP Neut") -> (w2696:string[])
                        n1707 = Build Array("CYCLE") -> (w2691:string[])
                        n1708 = Build Array("TEMP Live") -> (w2701:string[])
                        n1709 = Build Array("PF") -> (w2706:string[])
                        n1710 = Build Array("AMPS") -> (w2727:string[])
                        n1711 = Build Array("VOLTS") -> (w2718:string[])
                        n1712 = Unbundle(w2731) -> ("AMPS"=w2726:dbl, "VOLTS"=w2715:dbl, "PF"=w2714:dbl, "Tmp Live"=w2713:dbl, "Tmp Neut"=w2716:dbl)
                        n1713 = Unbundle(w2730) -> ("CYCLE"=w2711:dbl)  [unwired: 2 out]
                        n1714 = Build Array(w2715) -> (w2712:dbl[])
                        n1715 = Build Array(w2714) -> (w2705:dbl[])
                        n1716 = Build Array(w2713) -> (w2700:dbl[])
                        n1717 = Build Array(w2716) -> (w2695:dbl[])
                        n1718 = Build Array(w2726) -> (w2725:dbl[])
                        n1719 = Build Array(w2711) -> (w2690:dbl[])
                        n1720 = TDMS Write(0:w2732, 5:"LAB03-1 TEST VALUES", 7:w2727, 9:w2725) -> (4:w2720:refnum<k34>, 6:w2719:string, 15:w2707:errorcluster)  [unwired: 2 in, 1 out]
                        n1721 = TDMS Write(0:w2720, 5:w2719, 7:w2718, 9:w2712, 11:w2707) -> (4:w2710:refnum<k34>, 6:w2709:string, 15:w2708:errorcluster)  [unwired: 1 in, 1 out]
                        n1722 = TDMS Write(0:w2710, 5:w2709, 7:w2706, 9:w2705, 11:w2708) -> (4:w2704:refnum<k34>, 6:w2703:string, 15:w2702:errorcluster)  [unwired: 1 in, 1 out]
                        n1723 = TDMS Write(0:w2704, 5:w2703, 7:w2701, 9:w2700, 11:w2702) -> (4:w2699:refnum<k34>, 6:w2698:string, 15:w2697:errorcluster)  [unwired: 1 in, 1 out]
                        n1724 = TDMS Write(0:w2699, 5:w2698, 7:w2696, 9:w2695, 11:w2697) -> (4:w2694:refnum<k34>, 6:w2693:string, 15:w2692:errorcluster)  [unwired: 1 in, 1 out]
                        n1725 = TDMS Write(0:w2694, 5:w2693, 7:w2691, 9:w2690, 11:w2692) -> (15:w2689:errorcluster)  [unwired: 1 in, 3 out]
                        n1726 = local write "data file error"(w2689) -> ()
                      }
                    }
                  }
                  frame #5 {
                    # "LAB03-2"
                    n1727 = case shown="True" w2733 {
                      frame False {
                      }
                      frame True {
                        n1728 = local read "LAB03-2 (DISP)"() -> (w2775:T4)
                        n1729 = local read "LAB03-2 (SIG)"() -> (w2776:T2)
                        n1730 = local read "LAB03-2 (TDMS)"() -> (w2777:refnum<k34>)
                        n1731 = Build Array("TEMP Neut") -> (w2741:string[])
                        n1732 = Build Array("CYCLE") -> (w2736:string[])
                        n1733 = Build Array("TEMP Live") -> (w2746:string[])
                        n1734 = Build Array("PF") -> (w2751:string[])
                        n1735 = Build Array("AMPS") -> (w2772:string[])
                        n1736 = Build Array("VOLTS") -> (w2763:string[])
                        n1737 = Unbundle(w2776) -> ("AMPS"=w2771:dbl, "VOLTS"=w2760:dbl, "PF"=w2759:dbl, "Tmp Live"=w2758:dbl, "Tmp Neut"=w2761:dbl)
                        n1738 = Unbundle(w2775) -> ("CYCLE"=w2756:dbl)  [unwired: 2 out]
                        n1739 = Build Array(w2760) -> (w2757:dbl[])
                        n1740 = Build Array(w2759) -> (w2750:dbl[])
                        n1741 = Build Array(w2758) -> (w2745:dbl[])
                        n1742 = Build Array(w2761) -> (w2740:dbl[])
                        n1743 = Build Array(w2771) -> (w2770:dbl[])
                        n1744 = Build Array(w2756) -> (w2735:dbl[])
                        n1745 = TDMS Write(0:w2777, 5:"LAB03-2 TEST VALUES", 7:w2772, 9:w2770) -> (4:w2765:refnum<k34>, 6:w2764:string, 15:w2752:errorcluster)  [unwired: 2 in, 1 out]
                        n1746 = TDMS Write(0:w2765, 5:w2764, 7:w2763, 9:w2757, 11:w2752) -> (4:w2755:refnum<k34>, 6:w2754:string, 15:w2753:errorcluster)  [unwired: 1 in, 1 out]
                        n1747 = TDMS Write(0:w2755, 5:w2754, 7:w2751, 9:w2750, 11:w2753) -> (4:w2749:refnum<k34>, 6:w2748:string, 15:w2747:errorcluster)  [unwired: 1 in, 1 out]
                        n1748 = TDMS Write(0:w2749, 5:w2748, 7:w2746, 9:w2745, 11:w2747) -> (4:w2744:refnum<k34>, 6:w2743:string, 15:w2742:errorcluster)  [unwired: 1 in, 1 out]
                        n1749 = TDMS Write(0:w2744, 5:w2743, 7:w2741, 9:w2740, 11:w2742) -> (4:w2739:refnum<k34>, 6:w2738:string, 15:w2737:errorcluster)  [unwired: 1 in, 1 out]
                        n1750 = TDMS Write(0:w2739, 5:w2738, 7:w2736, 9:w2735, 11:w2737) -> (15:w2734:errorcluster)  [unwired: 1 in, 3 out]
                        n1751 = local write "data file error"(w2734) -> ()
                      }
                    }
                  }
                  frame #6 {
                    # "LAB04-1"
                    n1752 = case shown="True" w2778 {
                      frame False {
                      }
                      frame True {
                        n1753 = local read "LAB04-1 (DISP)"() -> (w2820:T4)
                        n1754 = local read "LAB04-1 (SIG)"() -> (w2821:T2)
                        n1755 = local read "LAB04-1 (TDMS)"() -> (w2822:refnum<k34>)
                        n1756 = Build Array("TEMP Neut") -> (w2786:string[])
                        n1757 = Build Array("CYCLE") -> (w2781:string[])
                        n1758 = Build Array("TEMP Live") -> (w2791:string[])
                        n1759 = Build Array("PF") -> (w2796:string[])
                        n1760 = Build Array("AMPS") -> (w2817:string[])
                        n1761 = Build Array("VOLTS") -> (w2808:string[])
                        n1762 = Unbundle(w2821) -> ("AMPS"=w2816:dbl, "VOLTS"=w2805:dbl, "PF"=w2804:dbl, "Tmp Live"=w2803:dbl, "Tmp Neut"=w2806:dbl)
                        n1763 = Unbundle(w2820) -> ("CYCLE"=w2801:dbl)  [unwired: 2 out]
                        n1764 = Build Array(w2805) -> (w2802:dbl[])
                        n1765 = Build Array(w2804) -> (w2795:dbl[])
                        n1766 = Build Array(w2803) -> (w2790:dbl[])
                        n1767 = Build Array(w2806) -> (w2785:dbl[])
                        n1768 = Build Array(w2816) -> (w2815:dbl[])
                        n1769 = Build Array(w2801) -> (w2780:dbl[])
                        n1770 = TDMS Write(0:w2822, 5:"LAB04-1 TEST VALUES", 7:w2817, 9:w2815) -> (4:w2810:refnum<k34>, 6:w2809:string, 15:w2797:errorcluster)  [unwired: 2 in, 1 out]
                        n1771 = TDMS Write(0:w2810, 5:w2809, 7:w2808, 9:w2802, 11:w2797) -> (4:w2800:refnum<k34>, 6:w2799:string, 15:w2798:errorcluster)  [unwired: 1 in, 1 out]
                        n1772 = TDMS Write(0:w2800, 5:w2799, 7:w2796, 9:w2795, 11:w2798) -> (4:w2794:refnum<k34>, 6:w2793:string, 15:w2792:errorcluster)  [unwired: 1 in, 1 out]
                        n1773 = TDMS Write(0:w2794, 5:w2793, 7:w2791, 9:w2790, 11:w2792) -> (4:w2789:refnum<k34>, 6:w2788:string, 15:w2787:errorcluster)  [unwired: 1 in, 1 out]
                        n1774 = TDMS Write(0:w2789, 5:w2788, 7:w2786, 9:w2785, 11:w2787) -> (4:w2784:refnum<k34>, 6:w2783:string, 15:w2782:errorcluster)  [unwired: 1 in, 1 out]
                        n1775 = TDMS Write(0:w2784, 5:w2783, 7:w2781, 9:w2780, 11:w2782) -> (15:w2779:errorcluster)  [unwired: 1 in, 3 out]
                        n1776 = local write "data file error"(w2779) -> ()
                      }
                    }
                  }
                  frame #7 {
                    # "LAB04-2"
                    n1777 = case shown="True" w2823 {
                      frame False {
                      }
                      frame True {
                        n1778 = local read "LAB04-2 (DISP)"() -> (w2865:T4)
                        n1779 = local read "LAB04-2 (SIG)"() -> (w2866:T2)
                        n1780 = local read "LAB04-2 (TDMS)"() -> (w2867:refnum<k34>)
                        n1781 = Build Array("TEMP Neut") -> (w2831:string[])
                        n1782 = Build Array("CYCLE") -> (w2826:string[])
                        n1783 = Build Array("TEMP Live") -> (w2836:string[])
                        n1784 = Build Array("PF") -> (w2841:string[])
                        n1785 = Build Array("AMPS") -> (w2862:string[])
                        n1786 = Build Array("VOLTS") -> (w2853:string[])
                        n1787 = Unbundle(w2866) -> ("AMPS"=w2861:dbl, "VOLTS"=w2850:dbl, "PF"=w2849:dbl, "Tmp Live"=w2848:dbl, "Tmp Neut"=w2851:dbl)
                        n1788 = Unbundle(w2865) -> ("CYCLE"=w2846:dbl)  [unwired: 2 out]
                        n1789 = Build Array(w2850) -> (w2847:dbl[])
                        n1790 = Build Array(w2849) -> (w2840:dbl[])
                        n1791 = Build Array(w2848) -> (w2835:dbl[])
                        n1792 = Build Array(w2851) -> (w2830:dbl[])
                        n1793 = Build Array(w2861) -> (w2860:dbl[])
                        n1794 = Build Array(w2846) -> (w2825:dbl[])
                        n1795 = TDMS Write(0:w2867, 5:"LAB04-2 TEST VALUES", 7:w2862, 9:w2860) -> (4:w2855:refnum<k34>, 6:w2854:string, 15:w2842:errorcluster)  [unwired: 2 in, 1 out]
                        n1796 = TDMS Write(0:w2855, 5:w2854, 7:w2853, 9:w2847, 11:w2842) -> (4:w2845:refnum<k34>, 6:w2844:string, 15:w2843:errorcluster)  [unwired: 1 in, 1 out]
                        n1797 = TDMS Write(0:w2845, 5:w2844, 7:w2841, 9:w2840, 11:w2843) -> (4:w2839:refnum<k34>, 6:w2838:string, 15:w2837:errorcluster)  [unwired: 1 in, 1 out]
                        n1798 = TDMS Write(0:w2839, 5:w2838, 7:w2836, 9:w2835, 11:w2837) -> (4:w2834:refnum<k34>, 6:w2833:string, 15:w2832:errorcluster)  [unwired: 1 in, 1 out]
                        n1799 = TDMS Write(0:w2834, 5:w2833, 7:w2831, 9:w2830, 11:w2832) -> (4:w2829:refnum<k34>, 6:w2828:string, 15:w2827:errorcluster)  [unwired: 1 in, 1 out]
                        n1800 = TDMS Write(0:w2829, 5:w2828, 7:w2826, 9:w2825, 11:w2827) -> (15:w2824:errorcluster)  [unwired: 1 in, 3 out]
                        n1801 = local write "data file error"(w2824) -> ()
                      }
                    }
                  }
                  frame #8 {
                    # "LAB05-1"
                    n1802 = case shown="True" w2868 {
                      frame False {
                      }
                      frame True {
                        n1803 = local read "LAB05-1 (DISP)"() -> (w2910:T4)
                        n1804 = local read "LAB05-1 (SIG)"() -> (w2911:T2)
                        n1805 = local read "LAB05-1 (TDMS)"() -> (w2912:refnum<k34>)
                        n1806 = Build Array("TEMP Neut") -> (w2876:string[])
                        n1807 = Build Array("CYCLE") -> (w2871:string[])
                        n1808 = Build Array("TEMP Live") -> (w2881:string[])
                        n1809 = Build Array("PF") -> (w2886:string[])
                        n1810 = Build Array("AMPS") -> (w2907:string[])
                        n1811 = Build Array("VOLTS") -> (w2898:string[])
                        n1812 = Unbundle(w2911) -> ("AMPS"=w2906:dbl, "VOLTS"=w2895:dbl, "PF"=w2894:dbl, "Tmp Live"=w2893:dbl, "Tmp Neut"=w2896:dbl)
                        n1813 = Unbundle(w2910) -> ("CYCLE"=w2891:dbl)  [unwired: 2 out]
                        n1814 = Build Array(w2895) -> (w2892:dbl[])
                        n1815 = Build Array(w2894) -> (w2885:dbl[])
                        n1816 = Build Array(w2893) -> (w2880:dbl[])
                        n1817 = Build Array(w2896) -> (w2875:dbl[])
                        n1818 = Build Array(w2906) -> (w2905:dbl[])
                        n1819 = Build Array(w2891) -> (w2870:dbl[])
                        n1820 = TDMS Write(0:w2912, 5:"LAB05-1 TEST VALUES", 7:w2907, 9:w2905) -> (4:w2900:refnum<k34>, 6:w2899:string, 15:w2887:errorcluster)  [unwired: 2 in, 1 out]
                        n1821 = TDMS Write(0:w2900, 5:w2899, 7:w2898, 9:w2892, 11:w2887) -> (4:w2890:refnum<k34>, 6:w2889:string, 15:w2888:errorcluster)  [unwired: 1 in, 1 out]
                        n1822 = TDMS Write(0:w2890, 5:w2889, 7:w2886, 9:w2885, 11:w2888) -> (4:w2884:refnum<k34>, 6:w2883:string, 15:w2882:errorcluster)  [unwired: 1 in, 1 out]
                        n1823 = TDMS Write(0:w2884, 5:w2883, 7:w2881, 9:w2880, 11:w2882) -> (4:w2879:refnum<k34>, 6:w2878:string, 15:w2877:errorcluster)  [unwired: 1 in, 1 out]
                        n1824 = TDMS Write(0:w2879, 5:w2878, 7:w2876, 9:w2875, 11:w2877) -> (4:w2874:refnum<k34>, 6:w2873:string, 15:w2872:errorcluster)  [unwired: 1 in, 1 out]
                        n1825 = TDMS Write(0:w2874, 5:w2873, 7:w2871, 9:w2870, 11:w2872) -> (15:w2869:errorcluster)  [unwired: 1 in, 3 out]
                        n1826 = local write "data file error"(w2869) -> ()
                      }
                    }
                  }
                  frame #9 {
                    # "LAB05-2"
                    n1827 = case shown="True" w2913 {
                      frame False {
                      }
                      frame True {
                        n1828 = local read "LAB05-2 (DISP)"() -> (w2955:T4)
                        n1829 = local read "LAB05-2 (SIG)"() -> (w2956:T2)
                        n1830 = local read "LAB05-2 (TDMS)"() -> (w2957:refnum<k34>)
                        n1831 = Build Array("TEMP Neut") -> (w2921:string[])
                        n1832 = Build Array("CYCLE") -> (w2916:string[])
                        n1833 = Build Array("TEMP Live") -> (w2926:string[])
                        n1834 = Build Array("PF") -> (w2931:string[])
                        n1835 = Build Array("AMPS") -> (w2952:string[])
                        n1836 = Build Array("VOLTS") -> (w2943:string[])
                        n1837 = Unbundle(w2956) -> ("AMPS"=w2951:dbl, "VOLTS"=w2940:dbl, "PF"=w2939:dbl, "Tmp Live"=w2938:dbl, "Tmp Neut"=w2941:dbl)
                        n1838 = Unbundle(w2955) -> ("CYCLE"=w2936:dbl)  [unwired: 2 out]
                        n1839 = Build Array(w2940) -> (w2937:dbl[])
                        n1840 = Build Array(w2939) -> (w2930:dbl[])
                        n1841 = Build Array(w2938) -> (w2925:dbl[])
                        n1842 = Build Array(w2941) -> (w2920:dbl[])
                        n1843 = Build Array(w2951) -> (w2950:dbl[])
                        n1844 = Build Array(w2936) -> (w2915:dbl[])
                        n1845 = TDMS Write(0:w2957, 5:"LAB05-2 TEST VALUES", 7:w2952, 9:w2950) -> (4:w2945:refnum<k34>, 6:w2944:string, 15:w2932:errorcluster)  [unwired: 2 in, 1 out]
                        n1846 = TDMS Write(0:w2945, 5:w2944, 7:w2943, 9:w2937, 11:w2932) -> (4:w2935:refnum<k34>, 6:w2934:string, 15:w2933:errorcluster)  [unwired: 1 in, 1 out]
                        n1847 = TDMS Write(0:w2935, 5:w2934, 7:w2931, 9:w2930, 11:w2933) -> (4:w2929:refnum<k34>, 6:w2928:string, 15:w2927:errorcluster)  [unwired: 1 in, 1 out]
                        n1848 = TDMS Write(0:w2929, 5:w2928, 7:w2926, 9:w2925, 11:w2927) -> (4:w2924:refnum<k34>, 6:w2923:string, 15:w2922:errorcluster)  [unwired: 1 in, 1 out]
                        n1849 = TDMS Write(0:w2924, 5:w2923, 7:w2921, 9:w2920, 11:w2922) -> (4:w2919:refnum<k34>, 6:w2918:string, 15:w2917:errorcluster)  [unwired: 1 in, 1 out]
                        n1850 = TDMS Write(0:w2919, 5:w2918, 7:w2916, 9:w2915, 11:w2917) -> (15:w2914:errorcluster)  [unwired: 1 in, 3 out]
                        n1851 = local write "data file error"(w2914) -> ()
                      }
                    }
                  }
                }
              }
            }
          }
          frame #13 {
            # "check for amps fail"
            # "check for cycle test & temperature rise fail conditions"
            n1852 = local read "on loops"() -> (w2983:dbl)
            n1853 = local read "jig cycle"() -> (w2980:dbl)
            n1854 = local read "jig cycle"() -> (w2985:dbl)
            n1855 = Add(x=w2983, y=3.0) -> (x+y=w2981:dbl)
            n1856 = Equal?(x=w2980, y=w2981) -> (x = y?=w2976:bool)
            n1857 = Equal?(x=w2985, y=1.0) -> (x = y?=w2978:bool)
            n1858 = stacked-sequence {
              tunnel: w2979 -> [w2988 _ _ _ _ _ _ _ _ _]
              tunnel: w2978 -> [w2989 w3008 w3027 w3046 w3065 w3084 w3103 w3122 w3141 w3160]
              tunnel: w2977 -> [w2986 _ _ _ _ _ _ _ _ _]
              tunnel: w2976 -> [w2987 w3007 w3026 w3045 w3064 w3083 w3102 w3121 w3140 w3159]
              tunnel: w2975 -> [_ w3006 _ _ _ _ _ _ _ _]
              tunnel: w2974 -> [_ w3005 _ _ _ _ _ _ _ _]
              tunnel: w2973 -> [_ _ w3025 _ _ _ _ _ _ _]
              tunnel: w2972 -> [_ _ w3024 _ _ _ _ _ _ _]
              tunnel: w2971 -> [_ _ _ w3044 _ _ _ _ _ _]
              tunnel: w2970 -> [_ _ _ w3043 _ _ _ _ _ _]
              tunnel: w2969 -> [_ _ _ _ w3063 _ _ _ _ _]
              tunnel: w2968 -> [_ _ _ _ w3062 _ _ _ _ _]
              tunnel: w2967 -> [_ _ _ _ _ w3082 _ _ _ _]
              tunnel: w2966 -> [_ _ _ _ _ w3081 _ _ _ _]
              tunnel: w2965 -> [_ _ _ _ _ _ w3101 _ _ _]
              tunnel: w2964 -> [_ _ _ _ _ _ w3100 _ _ _]
              tunnel: w2963 -> [_ _ _ _ _ _ _ w3120 _ _]
              tunnel: w2962 -> [_ _ _ _ _ _ _ w3119 _ _]
              tunnel: w2961 -> [_ _ _ _ _ _ _ _ w3139 _]
              tunnel: w2960 -> [_ _ _ _ _ _ _ _ w3138 _]
              tunnel: w2959 -> [_ _ _ _ _ _ _ _ _ w3158]
              tunnel: w2958 -> [_ _ _ _ _ _ _ _ _ w3157]
              frame #0 {
                # "LAB01-1"
                n1859 = case shown="True" w2986 {
                  tunnel: w2989 -> [_ w3001]
                  tunnel: w2988 -> [_ w2998]
                  tunnel: w2987 -> [_ w2997]
                  frame False {
                  }
                  frame True {
                    n1860 = local read "LAB01-1 (TEMP START)"() -> (w3003:cluster{"TL":dbl, "TN":dbl})
                    n1861 = local read "LAB01-1 (RESULT)"() -> (w2990:bool)
                    n1862 = local read "LAB01-1 (FAIL)"() -> (w2994:cluster{"LO":dbl, "HI":dbl})
                    n1863 = local read "LAB01-1 (TDMS)"() -> (w3002:refnum<k34>)
                    n1864 = local read "LAB01-1 (SET)"() -> (w2999:T5)
                    n1865 = local read "LAB01-1 (DISP)"() -> (w3000:T4)
                    n1866 = local read "LAB01-1 (SIG)"() -> (w3004:T2)
                    n1867 = Bundle("LAB01-1 (FAIL)"=w2994, "LAB01-1 (SIG)"=w3004, "LAB01-1 (TEMP START)"=w3003, "LAB01-1 (DISP)"=w3000, "LAB01-1 (SET)"=w2999, "LAB01-1 (TDMS)"=w3002) -> (w2992:T23)  [unwired: 1 in]
                    n1868 = call "sub vi - cycle&temp fail v5.vi"("Amps Lo?"=w3001, "Input Cluster"=w2992, "SELECT"=w2998, "Amps Hi?"=w2997, "Result In"=w2990) -> ("(FAIL) out"=w2993:cluster{"FAIL LO":dbl, "FAIL HI":dbl}, "(DISP) out"=w2996:T4, "Result Out"=w2991:bool, "file error"=w2995:errorcluster)  [unwired: 11 in]
                    n1869 = local write "LAB01-1 (FAIL)"(w2993) -> ()
                    n1870 = local write "LAB01-1 (DISP)"(w2996) -> ()
                    n1871 = local write "LAB01-1 (RESULT)"(w2991) -> ()
                    n1872 = local write "data file error"(w2995) -> ()
                  }
                }
              }
              frame #1 {
                # "LAB01-2"
                n1873 = case shown="True" w3006 {
                  tunnel: w3008 -> [_ w3020]
                  tunnel: w3005 -> [_ w3017]
                  tunnel: w3007 -> [_ w3016]
                  frame False {
                  }
                  frame True {
                    n1874 = local read "LAB01-2 (TEMP START)"() -> (w3022:cluster{"TL":dbl, "TN":dbl})
                    n1875 = local read "LAB01-2 (FAIL)"() -> (w3013:cluster{"LO":dbl, "HI":dbl})
                    n1876 = local read "LAB01-2 (TDMS)"() -> (w3021:refnum<k34>)
                    n1877 = local read "LAB01-2 (SET)"() -> (w3018:T5)
                    n1878 = local read "LAB01-2 (DISP)"() -> (w3019:T4)
                    n1879 = local read "LAB01-2 (RESULT)"() -> (w3009:bool)
                    n1880 = local read "LAB01-2 (SIG)"() -> (w3023:T2)
                    n1881 = Bundle("LAB01-2 (FAIL)"=w3013, "LAB01-2 (SIG)"=w3023, "LAB01-2 (TEMP START)"=w3022, "LAB01-2 (DISP)"=w3019, "LAB01-2 (SET)"=w3018, "LAB01-2 (TDMS)"=w3021) -> (w3011:T24)  [unwired: 1 in]
                    n1882 = call "sub vi - cycle&temp fail v5.vi"("Amps Lo?"=w3020, "Input Cluster"=w3011, "SELECT"=w3017, "Amps Hi?"=w3016, "Result In"=w3009) -> ("(FAIL) out"=w3012:cluster{"FAIL LO":dbl, "FAIL HI":dbl}, "(DISP) out"=w3015:T4, "Result Out"=w3010:bool, "file error"=w3014:errorcluster)  [unwired: 11 in]
                    n1883 = local write "LAB01-2 (FAIL)"(w3012) -> ()
                    n1884 = local write "LAB01-2 (DISP)"(w3015) -> ()
                    n1885 = local write "LAB01-2 (RESULT)"(w3010) -> ()
                    n1886 = local write "data file error"(w3014) -> ()
                  }
                }
              }
              frame #2 {
                # "LAB02-1"
                n1887 = case shown="True" w3025 {
                  tunnel: w3027 -> [_ w3039]
                  tunnel: w3024 -> [_ w3036]
                  tunnel: w3026 -> [_ w3035]
                  frame False {
                  }
                  frame True {
                    n1888 = local read "LAB02-1 (TEMP START)"() -> (w3041:cluster{"TL":dbl, "TN":dbl})
                    n1889 = local read "LAB02-1 (FAIL)"() -> (w3032:cluster{"LO":dbl, "HI":dbl})
                    n1890 = local read "LAB02-1 (TDMS)"() -> (w3040:refnum<k34>)
                    n1891 = local read "LAB02-1 (SET)"() -> (w3037:T5)
                    n1892 = local read "LAB02-1 (DISP)"() -> (w3038:T4)
                    n1893 = local read "LAB02-1 (SIG)"() -> (w3042:T2)
                    n1894 = local read "LAB02-1 (RESULT)"() -> (w3028:bool)
                    n1895 = Bundle("LAB02-1 (FAIL)"=w3032, "LAB02-1 (SIG)"=w3042, "LAB02-1 (TEMP START)"=w3041, "LAB02-1 (DISP)"=w3038, "LAB02-1 (SET)"=w3037, "LAB02-1 (TDMS)"=w3040) -> (w3030:T25)  [unwired: 1 in]
                    n1896 = call "sub vi - cycle&temp fail v5.vi"("Amps Lo?"=w3039, "Input Cluster"=w3030, "SELECT"=w3036, "Amps Hi?"=w3035, "Result In"=w3028) -> ("(FAIL) out"=w3031:cluster{"FAIL LO":dbl, "FAIL HI":dbl}, "(DISP) out"=w3034:T4, "Result Out"=w3029:bool, "file error"=w3033:errorcluster)  [unwired: 11 in]
                    n1897 = local write "LAB02-1 (FAIL)"(w3031) -> ()
                    n1898 = local write "LAB02-1 (DISP)"(w3034) -> ()
                    n1899 = local write "LAB02-1 (RESULT)"(w3029) -> ()
                    n1900 = local write "data file error"(w3033) -> ()
                  }
                }
              }
              frame #3 {
                # "LAB02-2"
                n1901 = case shown="True" w3044 {
                  tunnel: w3046 -> [_ w3058]
                  tunnel: w3043 -> [_ w3055]
                  tunnel: w3045 -> [_ w3054]
                  frame False {
                  }
                  frame True {
                    n1902 = local read "LAB02-2 (TEMP START)"() -> (w3060:cluster{"TL":dbl, "TN":dbl})
                    n1903 = local read "LAB02-2 (FAIL)"() -> (w3051:cluster{"LO":dbl, "HI":dbl})
                    n1904 = local read "LAB02-2 (TDMS)"() -> (w3059:refnum<k34>)
                    n1905 = local read "LAB02-2 (SET)"() -> (w3056:T5)
                    n1906 = local read "LAB02-2 (DISP)"() -> (w3057:T4)
                    n1907 = local read "LAB02-2 (SIG)"() -> (w3061:T2)
                    n1908 = local read "LAB02-2 (RESULT)"() -> (w3047:bool)
                    n1909 = Bundle("LAB02-2 (FAIL)"=w3051, "LAB02-2 (SIG)"=w3061, "LAB02-2 (TEMP START)"=w3060, "LAB02-2 (DISP)"=w3057, "LAB02-2 (SET)"=w3056, "LAB02-2 (TDMS)"=w3059) -> (w3049:T26)  [unwired: 1 in]
                    n1910 = call "sub vi - cycle&temp fail v5.vi"("Amps Lo?"=w3058, "Input Cluster"=w3049, "SELECT"=w3055, "Amps Hi?"=w3054, "Result In"=w3047) -> ("(FAIL) out"=w3050:cluster{"FAIL LO":dbl, "FAIL HI":dbl}, "(DISP) out"=w3053:T4, "Result Out"=w3048:bool, "file error"=w3052:errorcluster)  [unwired: 11 in]
                    n1911 = local write "LAB02-2 (FAIL)"(w3050) -> ()
                    n1912 = local write "LAB02-2 (DISP)"(w3053) -> ()
                    n1913 = local write "LAB02-2 (RESULT)"(w3048) -> ()
                    n1914 = local write "data file error"(w3052) -> ()
                  }
                }
              }
              frame #4 {
                # "LAB03-1"
                n1915 = case shown="True" w3063 {
                  tunnel: w3065 -> [_ w3077]
                  tunnel: w3062 -> [_ w3074]
                  tunnel: w3064 -> [_ w3073]
                  frame False {
                  }
                  frame True {
                    n1916 = local read "LAB03-1 (TEMP START)"() -> (w3079:cluster{"TL":dbl, "TN":dbl})
                    n1917 = local read "LAB03-1 (FAIL)"() -> (w3070:cluster{"LO":dbl, "HI":dbl})
                    n1918 = local read "LAB03-1 (TDMS)"() -> (w3078:refnum<k34>)
                    n1919 = local read "LAB03-1 (SET)"() -> (w3075:T5)
                    n1920 = local read "LAB03-1 (DISP)"() -> (w3076:T4)
                    n1921 = local read "LAB03-1 (SIG)"() -> (w3080:T2)
                    n1922 = local read "LAB03-1 (RESULT)"() -> (w3066:bool)
                    n1923 = Bundle("LAB03-1 (FAIL)"=w3070, "LAB03-1 (SIG)"=w3080, "LAB03-1 (TEMP START)"=w3079, "LAB03-1 (DISP)"=w3076, "LAB03-1 (SET)"=w3075, "LAB03-1 (TDMS)"=w3078) -> (w3068:T27)  [unwired: 1 in]
                    n1924 = call "sub vi - cycle&temp fail v5.vi"("Amps Lo?"=w3077, "Input Cluster"=w3068, "SELECT"=w3074, "Amps Hi?"=w3073, "Result In"=w3066) -> ("(FAIL) out"=w3069:cluster{"FAIL LO":dbl, "FAIL HI":dbl}, "(DISP) out"=w3072:T4, "Result Out"=w3067:bool, "file error"=w3071:errorcluster)  [unwired: 11 in]
                    n1925 = local write "LAB03-1 (FAIL)"(w3069) -> ()
                    n1926 = local write "LAB03-1 (DISP)"(w3072) -> ()
                    n1927 = local write "LAB03-1 (RESULT)"(w3067) -> ()
                    n1928 = local write "data file error"(w3071) -> ()
                  }
                }
              }
              frame #5 {
                # "LAB03-2"
                n1929 = case shown="True" w3082 {
                  tunnel: w3084 -> [_ w3096]
                  tunnel: w3081 -> [_ w3093]
                  tunnel: w3083 -> [_ w3092]
                  frame False {
                  }
                  frame True {
                    n1930 = local read "LAB03-2 (TEMP START)"() -> (w3098:cluster{"TL":dbl, "TN":dbl})
                    n1931 = local read "LAB03-2 (FAIL)"() -> (w3089:cluster{"LO":dbl, "HI":dbl})
                    n1932 = local read "LAB03-2 (TDMS)"() -> (w3097:refnum<k34>)
                    n1933 = local read "LAB03-2 (SET)"() -> (w3094:T5)
                    n1934 = local read "LAB03-2 (DISP)"() -> (w3095:T4)
                    n1935 = local read "LAB03-2 (RESULT)"() -> (w3085:bool)
                    n1936 = local read "LAB03-2 (SIG)"() -> (w3099:T2)
                    n1937 = Bundle("LAB03-2 (FAIL)"=w3089, "LAB03-2 (SIG)"=w3099, "LAB03-2 (TEMP START)"=w3098, "LAB03-2 (DISP)"=w3095, "LAB03-2 (SET)"=w3094, "LAB03-2 (TDMS)"=w3097) -> (w3087:T28)  [unwired: 1 in]
                    n1938 = call "sub vi - cycle&temp fail v5.vi"("Amps Lo?"=w3096, "Input Cluster"=w3087, "SELECT"=w3093, "Amps Hi?"=w3092, "Result In"=w3085) -> ("(FAIL) out"=w3088:cluster{"FAIL LO":dbl, "FAIL HI":dbl}, "(DISP) out"=w3091:T4, "Result Out"=w3086:bool, "file error"=w3090:errorcluster)  [unwired: 11 in]
                    n1939 = local write "LAB03-2 (FAIL)"(w3088) -> ()
                    n1940 = local write "LAB03-2 (DISP)"(w3091) -> ()
                    n1941 = local write "LAB03-2 (RESULT)"(w3086) -> ()
                    n1942 = local write "data file error"(w3090) -> ()
                  }
                }
              }
              frame #6 {
                # "LAB04-1"
                n1943 = case shown="True" w3101 {
                  tunnel: w3103 -> [_ w3115]
                  tunnel: w3100 -> [_ w3112]
                  tunnel: w3102 -> [_ w3111]
                  frame False {
                  }
                  frame True {
                    n1944 = local read "LAB04-1 (TEMP START)"() -> (w3117:cluster{"TL":dbl, "TN":dbl})
                    n1945 = local read "LAB04-1 (FAIL)"() -> (w3108:cluster{"LO":dbl, "HI":dbl})
                    n1946 = local read "LAB04-1 (TDMS)"() -> (w3116:refnum<k34>)
                    n1947 = local read "LAB04-1 (SET)"() -> (w3113:T5)
                    n1948 = local read "LAB04-1 (DISP)"() -> (w3114:T4)
                    n1949 = local read "LAB04-1 (SIG)"() -> (w3118:T2)
                    n1950 = local read "LAB04-1 (RESULT)"() -> (w3104:bool)
                    n1951 = Bundle("LAB04-1 (FAIL)"=w3108, "LAB04-1 (SIG)"=w3118, "LAB04-1 (TEMP START)"=w3117, "LAB04-1 (DISP)"=w3114, "LAB04-1 (SET)"=w3113, "LAB04-1 (TDMS)"=w3116) -> (w3106:T29)  [unwired: 1 in]
                    n1952 = call "sub vi - cycle&temp fail v5.vi"("Amps Lo?"=w3115, "Input Cluster"=w3106, "SELECT"=w3112, "Amps Hi?"=w3111, "Result In"=w3104) -> ("(FAIL) out"=w3107:cluster{"FAIL LO":dbl, "FAIL HI":dbl}, "(DISP) out"=w3110:T4, "Result Out"=w3105:bool, "file error"=w3109:errorcluster)  [unwired: 11 in]
                    n1953 = local write "LAB04-1 (FAIL)"(w3107) -> ()
                    n1954 = local write "LAB04-1 (DISP)"(w3110) -> ()
                    n1955 = local write "LAB04-1 (RESULT)"(w3105) -> ()
                    n1956 = local write "data file error"(w3109) -> ()
                  }
                }
              }
              frame #7 {
                # "LAB04-2"
                n1957 = case shown="True" w3120 {
                  tunnel: w3122 -> [_ w3134]
                  tunnel: w3119 -> [_ w3131]
                  tunnel: w3121 -> [_ w3130]
                  frame False {
                  }
                  frame True {
                    n1958 = local read "LAB04-2 (TEMP START)"() -> (w3136:cluster{"TL":dbl, "TN":dbl})
                    n1959 = local read "LAB04-2 (FAIL)"() -> (w3127:cluster{"LO":dbl, "HI":dbl})
                    n1960 = local read "LAB04-2 (TDMS)"() -> (w3135:refnum<k34>)
                    n1961 = local read "LAB04-2 (SET)"() -> (w3132:T5)
                    n1962 = local read "LAB04-2 (DISP)"() -> (w3133:T4)
                    n1963 = local read "LAB04-2 (SIG)"() -> (w3137:T2)
                    n1964 = local read "LAB04-2 (RESULT)"() -> (w3123:bool)
                    n1965 = Bundle("LAB04-2 (FAIL)"=w3127, "LAB04-2 (SIG)"=w3137, "LAB04-2 (TEMP START)"=w3136, "LAB04-2 (DISP)"=w3133, "LAB04-2 (SET)"=w3132, "LAB04-2 (TDMS)"=w3135) -> (w3125:T30)  [unwired: 1 in]
                    n1966 = call "sub vi - cycle&temp fail v5.vi"("Amps Lo?"=w3134, "Input Cluster"=w3125, "SELECT"=w3131, "Amps Hi?"=w3130, "Result In"=w3123) -> ("(FAIL) out"=w3126:cluster{"FAIL LO":dbl, "FAIL HI":dbl}, "(DISP) out"=w3129:T4, "Result Out"=w3124:bool, "file error"=w3128:errorcluster)  [unwired: 11 in]
                    n1967 = local write "LAB04-2 (FAIL)"(w3126) -> ()
                    n1968 = local write "LAB04-2 (DISP)"(w3129) -> ()
                    n1969 = local write "LAB04-2 (RESULT)"(w3124) -> ()
                    n1970 = local write "data file error"(w3128) -> ()
                  }
                }
              }
              frame #8 {
                # "LAB05-1"
                n1971 = case shown="True" w3139 {
                  tunnel: w3141 -> [_ w3153]
                  tunnel: w3138 -> [_ w3150]
                  tunnel: w3140 -> [_ w3149]
                  frame False {
                  }
                  frame True {
                    n1972 = local read "LAB05-1 (TEMP START)"() -> (w3155:cluster{"TL":dbl, "TN":dbl})
                    n1973 = local read "LAB05-1 (FAIL)"() -> (w3146:cluster{"LO":dbl, "HI":dbl})
                    n1974 = local read "LAB05-1 (TDMS)"() -> (w3154:refnum<k34>)
                    n1975 = local read "LAB05-1 (SET)"() -> (w3151:T5)
                    n1976 = local read "LAB05-1 (DISP)"() -> (w3152:T4)
                    n1977 = local read "LAB05-1 (SIG)"() -> (w3156:T2)
                    n1978 = local read "LAB05-1 (RESULT)"() -> (w3142:bool)
                    n1979 = Bundle("LAB05-1 (FAIL)"=w3146, "LAB05-1 (SIG)"=w3156, "LAB05-1 (TEMP START)"=w3155, "LAB05-1 (DISP)"=w3152, "LAB05-1 (SET)"=w3151, "LAB05-1 (TDMS)"=w3154) -> (w3144:T31)  [unwired: 1 in]
                    n1980 = call "sub vi - cycle&temp fail v5.vi"("Amps Lo?"=w3153, "Input Cluster"=w3144, "SELECT"=w3150, "Amps Hi?"=w3149, "Result In"=w3142) -> ("(FAIL) out"=w3145:cluster{"FAIL LO":dbl, "FAIL HI":dbl}, "(DISP) out"=w3148:T4, "Result Out"=w3143:bool, "file error"=w3147:errorcluster)  [unwired: 11 in]
                    n1981 = local write "LAB05-1 (FAIL)"(w3145) -> ()
                    n1982 = local write "LAB05-1 (DISP)"(w3148) -> ()
                    n1983 = local write "LAB05-1 (RESULT)"(w3143) -> ()
                    n1984 = local write "data file error"(w3147) -> ()
                  }
                }
              }
              frame #9 {
                # "LAB05-2"
                n1985 = case shown="True" w3158 {
                  tunnel: w3160 -> [_ w3172]
                  tunnel: w3157 -> [_ w3169]
                  tunnel: w3159 -> [_ w3168]
                  frame False {
                  }
                  frame True {
                    n1986 = local read "LAB05-2 (TEMP START)"() -> (w3174:cluster{"TL":dbl, "TN":dbl})
                    n1987 = local read "LAB05-2 (FAIL)"() -> (w3165:cluster{"LO":dbl, "HI":dbl})
                    n1988 = local read "LAB05-2 (TDMS)"() -> (w3173:refnum<k34>)
                    n1989 = local read "LAB05-2 (SET)"() -> (w3170:T5)
                    n1990 = local read "LAB05-2 (DISP)"() -> (w3171:T4)
                    n1991 = local read "LAB05-2 (SIG)"() -> (w3175:T2)
                    n1992 = local read "LAB05-2 (RESULT)"() -> (w3161:bool)
                    n1993 = Bundle("LAB05-2 (FAIL)"=w3165, "LAB05-2 (SIG)"=w3175, "LAB05-2 (TEMP START)"=w3174, "LAB05-2 (DISP)"=w3171, "LAB05-2 (SET)"=w3170, "LAB05-2 (TDMS)"=w3173) -> (w3163:T32)  [unwired: 1 in]
                    n1994 = call "sub vi - cycle&temp fail v5.vi"("Amps Lo?"=w3172, "Input Cluster"=w3163, "SELECT"=w3169, "Amps Hi?"=w3168, "Result In"=w3161) -> ("(FAIL) out"=w3164:cluster{"FAIL LO":dbl, "FAIL HI":dbl}, "(DISP) out"=w3167:T4, "Result Out"=w3162:bool, "file error"=w3166:errorcluster)  [unwired: 11 in]
                    n1995 = local write "LAB05-2 (FAIL)"(w3164) -> ()
                    n1996 = local write "LAB05-2 (DISP)"(w3167) -> ()
                    n1997 = local write "LAB05-2 (RESULT)"(w3162) -> ()
                    n1998 = local write "data file error"(w3166) -> ()
                  }
                }
              }
            }
          }
          frame #14 {
            # "run calibration routine"
            n1999 = local read "CALIBRATE"() -> (w3176:bool)
            n2000 = case shown="True" w3176 {
              frame False {
              }
              frame True {
                n2001 = stacked-sequence {
                  seq-local: [w3177 _ _] -> [_ w3179 _]
                  frame #0 {
                    n2002 = call "CALIBRATION PASSWORD"() -> ("PASSWORD"=w3177:string)  [unwired: 17 in, 2 out]
                  }
                  frame #1 {
                    n2003 = Equal?(x=w3179, y="7777") -> (x = y?=w3178:bool)
                    n2004 = case shown="True" w3178 {
                      frame False {
                      }
                      frame True {
                        n2005 = stacked-sequence {
                          frame #0 {
                            n2006 = call "sub vi - calibration v1.vi"() -> ()  [unwired: 12 in]
                          }
                          frame #1 {
                            n2007 = call "sub vi - get calibration values v1.vi"() -> ("LAB01 (CAL)"=w3185:T6, "LAB02 (CAL)"=w3184:T7, "LAB03 (CAL)"=w3183:T6, "LAB04 (CAL)"=w3182:T6, "calibration file error out"=w3186:errorcluster, "LAB05 (CAL)"=w3181:T6)  [unwired: 10 in]
                            n2008 = local write "calibration file error out"(w3186) -> ()
                            n2009 = local write "LAB04 (CAL)"(w3182) -> ()
                            n2010 = local write "LAB05 (CAL)"(w3181) -> ()
                            n2011 = local write "LAB01 (CAL)"(w3185) -> ()
                            n2012 = local write "LAB02 (CAL)"(w3184) -> ()
                            n2013 = local write "LAB03 (CAL)"(w3183) -> ()
                          }
                        }
                      }
                    }
                  }
                  frame #2 {
                    n2014 = local write "CALIBRATE"(FALSE) -> ()
                  }
                }
              }
            }
          }
          frame #15 {
            # "save certain settings to file"
            n2015 = String To Path(string="c:\\crabtree\\Set Up\\") -> (path=w3190:path)
            n2016 = Build Path(base path=w3190, name or relative path="settings.bin") -> (appended path=w3188:path)
            n2017 = Create Folder(path (use dialog)=w3190) -> (error out=w3192:errorcluster)  [unwired: 2 in, 2 out]
            n2018 = call <vilib>:"Clear Errors.vi"("error in (no error)"=w3192) -> ()  [unwired: 6 in, 1 out]
            n2019 = stacked-sequence {
              seq-local: [w3193 _] -> [_ w3205]
              tunnel: w3188 -> [_ w3206]
              frame #0 {
                n2020 = local read "Network Directory"() -> (w3198:path)
                n2021 = local read "LAB05-2 (SET)"() -> (w3197:T5)
                n2022 = local read "LAB05-1 (SET)"() -> (w3196:T5)
                n2023 = local read "LAB04-2 (SET)"() -> (w3195:T5)
                n2024 = local read "LAB03-2 (SET)"() -> (w3199:T5)
                n2025 = local read "LAB04-1 (SET)"() -> (w3194:T5)
                n2026 = local read "LAB03-1 (SET)"() -> (w3200:T5)
                n2027 = local read "LAB02-2 (SET)"() -> (w3201:T5)
                n2028 = local read "LAB02-1 (SET)"() -> (w3202:T5)
                n2029 = local read "LAB01-2 (SET)"() -> (w3203:T5)
                n2030 = local read "LAB01-1 (SET)"() -> (w3204:T5)
                n2031 = Bundle("LAB01-1 (SET)"=w3204, "LAB01-2 (SET)"=w3203, "LAB02-1 (SET)"=w3202, "LAB02-2 (SET)"=w3201, "LAB03-1 (SET)"=w3200, "LAB03-2 (SET)"=w3199, "LAB04-1 (SET)"=w3194, "LAB04-2 (SET)"=w3195, "LAB05-1 (SET)"=w3196, "LAB05-2 (SET)"=w3197, "Network Directory"=w3198) -> (w3193:T16)  [unwired: 1 in]
              }
              frame #1 {
                n2032 = event shown="[1] \"LAB01-1 (SET)\", \"LAB01-2 (SET)\", \"LAB02-1 (SET)\", \"LAB02-2 (SET)\", \"LAB03-1 (SET)\", \"LAB03-2 (SET)\", \"LAB04-1 (SET)\", \"LAB04-2 (SET)\", \"LAB05-1 (SET)\", \"LAB05-2 (SET)\", \"Network Directory\": Value Change" {
                  selector: _ -> [_ _]
                  dyn-events: _ -> [_ _]
                  timeout: 10.0 -> [_ _]
                  tunnel: w3206 -> [_ w3208]
                  tunnel: w3205 -> [_ w3209]
                  event Timeout {
                    n2033 = event-data() -> ()  [unwired: 1 in, 3 out]
                  }
                  event "LAB01-1 (SET)", "LAB01-2 (SET)", "LAB02-1 (SET)", "LAB02-2 (SET)", "LAB03-1 (SET)", "LAB03-2 (SET)", "LAB04-1 (SET)", "LAB04-2 (SET)", "LAB05-1 (SET)", "LAB05-2 (SET)", "Network Directory": Value Change {
                    n2034 = event-data() -> ()  [unwired: 1 in, 6 out]
                    n2035 = Open/Create/Replace File(file path (use dialog)=w3208, operation (0:open)=T15."replace or create") -> (refnum out=w3214:refnum<file>, error out=w3213:errorcluster)  [unwired: 4 in, 1 out]
                    n2036 = Write to Binary File(file (use dialog)=w3214, data=w3209, error in=w3213) -> (refnum out=w3212:refnum<file>, error out=w3211:errorcluster)  [unwired: 3 in, 1 out]
                    n2037 = Close File(refnum=w3212, error in=w3211) -> (error out=w3210:errorcluster)  [unwired: 1 out]
                    n2038 = local write "data file error"(w3210) -> ()
                  }
                }
              }
            }
          }
        }
        n2039 = node-c288() -> ()  [unwired: 1 in, 1 out]
        "loops" <- w70
      }
      n2040 = node-c288(w47) -> ()  [unwired: 1 out]
    }
  }
